vi "MultiOpto_1.1_Host.vi"() -> ()   [LabVIEW 2018]
uses:
  D:/NI LabVIEW/MultiOpto 1.1/AT lib/Spels.AutomationTools.Utility.Wcf.dll
  AT lib/Spels.AutomationTools.Utility.Wcf.dll
  D:/NI LabVIEW/MultiOpto 1.1/AT lib/AmateurStepperMotor.dll
  AT lib/AmateurStepperMotor.dll
  <instrlib>/niDMM/nidmm.llb/niDMM Resolution in Digits.ctl
  <instrlib>/niDMM/nidmm.llb/niDMM Function.ctl
  <instrlib>/niDCPower/nidcpower.llb/niDCPower Measurement Type.ctl
  <instrlib>/niDMM/nidmm.llb/niDMM Configure Measurement Digits.vi
  <instrlib>/niScope/Configure/Trigger/niScope Configure Trigger Window.vi
  <instrlib>/niScope/Acquire/Fetch/niScope Multi Fetch Cluster.vi
  <instrlib>/niScope/Acquire/Fetch/niScope Fetch.vi
panel:
  in  "Table Tab":enum32{"Glass Table", "Var"}(tab)
  in  "Add Log Remark":bool
  in  "Glass Table":string[][](table)=[["", "455 nm", "808 nm", "1550 nm"], ["Glass 1 (H-ZLaF90)", "", "", ""], ["Glass 2 (H-K9L)", "", "", ""], ["Glass 3 (H-ZF7LA)", "", "", ""], ["Glass 4 (H-LaK7A)", "", "", ""]]
  in  "Clear Table":bool
  out "Num of Meas":u32
  in  "Log Remark":string
  out "WL 808":dbl format="%#_4g"
  out "WL 455":dbl format="%#_4g"
  out "WL 1550":dbl format="%#_4g"
  out "WL 1550 Ref":dbl=1.0 format="%#_4g"
  out "WL 455 Ref":dbl=1.0 format="%#_4g"
  out "WL 808 Ref":dbl=1.0 format="%#_4g"
  out "WL 455 Absolute/Reference":string="-" caption="WL 455 Abs/Ref"
  out "WL 808 Absolute/Reference":string="-" caption="WL 808 Abs/Ref"
  out "WL 1550 Absolute/Reference":string="-" caption="WL 1550 Abs/Ref"
  in  "Set Last Meas As Ref":bool
  in  "HMI Stop":bool
  in  "NI Scope":refnum<k15>="PXI1Slot9_2" caption="Scope"
  in  "NI DMM 3":refnum<k15>="PXI1Slot6_3" caption="NI DMM 2"
  in  "Stepper Motor Control":enum32{"Stepper Motor", "System Panel", "Var"}(tab)
  out "Текущая позиция":dbl
  in  "Куда едем?":T1(ring)
  in  "Glass Meas":bool caption="Glass Measurement"
  out "Meas Running":bool
  out "Glass Meas Cycle Running":bool caption="Cycle Running"
  in  "Погнали!":bool
  out "Готово":bool
  in  "Glass Meas Cycle":bool caption="Glass Measament Cycle"
  out "Meas Progress Bar":u8(slide) caption="Measurement Progress Bar" scale=0.0..100.0
  out "Stepper Motor Status":bool=TRUE
  in  "StepDivisor":i32(ring)=8 items=["D1"=1, "D2"=2, "D4"=4, "D8"=8, "D16"=16, "D32"=32]
  in  "Speed":dbl=1000.0
  in  "StepMultiplicationFactor":dbl=1.0
  in  "Стоп_тест":bool
  in  "Тест":bool
  in  "Стоп GoTo":bool
  in  "Meas Wait":u32=500
  out "Av Cur Data String":string="0,000016350563\t"
  out "Glass Num Output File":refnum<file>
  out "Glass 1 Output File":refnum<file>
  out "CH Data String":string="1,200000000000\t0,040047418764\t"
  out "All Cur Data String":string="0,000016366024\t0,000016373619\t0,000016386890\t0,000016310874\t0,000016315407\t"
  out "Meas Time String":string="19:17:01:,978\t"
  out "Glass Meas Path":refnum<file>
  out "Glass 2 Output File":refnum<file>
  out "Glass 3 Output File":refnum<file>
  out "Glass 4 Output File":refnum<file>
  out "Glass Full Log Output File":refnum<file>
  out "Save Glass Log Done":bool=TRUE
  in  "Save Glass Log Data":bool
  out "WL-i":i32
  out "Single Meas Output File":refnum<file>
  in  "NI DMM 3 Tab":enum32{"Amp", "Ohm", "System Panel", "Var"}(tab)
  in  "NI DMM 3 Ampermeter path":path=path "D:/NI LabVIEW/MultiOpto 1.1/Logs/DMM 3" caption="Ampermeter Path"
  out "NI DMM 3 Current Char":dbl(graph)=0.00060711613514286
  in  "NI DMM 3 Current Wait":u32=100 caption="Wait"
  out "NI DMM 3 Current":dbl=0.00060711613514286 caption="Current" format="%_6g"
  in  "NI DMM 3 units":string(combo)="1000000" caption="Units"
  in  "NI DMM 3 Current Range":string(combo)="-1" caption="Range"
  in  "NI DMM 3 Ohmmeter path":path=path "C:/AAB/MultiOpto/NI DMM 2" caption="Ohmmeter Path"
  out "NI DMM 3 Resistance Char":dbl(graph)=6.67426339573744e-05
  in  "NI DMM 3 Resistance Wait":u32=100 caption="Wait"
  out "NI DMM 3 Resistance":dbl caption="Resistance" format="%_6g"
  in  "NI DMM 3 Resistance units":string(combo)="1" caption="Units"
  in  "NI DMM 3 Resistance Range":string(combo)="-1" caption="Range"
  out "NI DMM 3 Current output file":refnum<file>
  out "NI DMM 3 Resistance output file":refnum<file>
  in  "NI DMM 3 error in":errorcluster
  out "NI DMM 3 Status":bool=TRUE
  out "NI DMM 3 Option Return":enum32{"Ampermeter button", "Ohmmeter button"}(ring)
  out "NI DMM 3 error out":errorcluster
  out "DMM 3 Real Current":dbl=6.0711613514286e-10 format="%.5f"
  in  "NI DMM 1":refnum<k15>="PXI1Slot4"
  in  "NI DMM 2":refnum<k15>="PXI1Slot5"
  in  "All Glass Path":path=path "D:/NI LabVIEW/MultiOpto 1.1/Logs/All Glass"
  in  "Ophir 2 Tab":enum32{"Ophir 2", "System Panel"}(tab)
  out "Ophir 2 Initialization":bool caption="Initialization"
  in  "Ophir 2 Clear":bool caption="Clear"
  out "Ophir 2 MAX":dbl caption="MAX" format="%#_5g"
  out "Ophir 2 Optical Power":dbl caption="Power" format="%#_4g"
  in  "Ophir 2 units":string(combo)="1000" caption="Units"
  in  "Ophir 2 Info":u16(ring)=1 caption="Info" items=["Device : JUNO; s/n:903794", "Head : PD300-IRG-v1; s/n:908004"]
  in  "Ophir 2 Wait":u32=100 caption="Wait"
  out "Ophir 2 Char":dbl(graph)=6.67426339573744e-05
  out "Ophir 2 Over Range":bool caption="Over Range"
  out "Ophir 2 dup Visa Session":refnum<visa-resource-name>="USB0::0x0BD3::0x0777::NI-VISA-10003::RAW" caption="dup Visa Session"
  in  "Ophir 2 GPIB Address (10)":string="10" caption="GPIB Address (10)"
  in  "Ophir 2 Select Communication Protocol":u16(ring) caption="Select Communication Protocol" items=["USB", "RS232", "GPIB"]
  in  "Ophir 2 usb channel":i16 caption="usb channel"
  in  "Ophir 2 Baud Rate (3:9600)":i16(ring)=3 caption="Baud Rate (3:9600)" items=["300", "1200", "4800", "9600", "19200", "38400"]
  in  "Ophir 2 Port Number (default 2)":i16=2 caption="Port Number (default 2)" min=0 max=20
  out "Ophir 2 Status":bool caption="Status"
  out "Ophir 2 Real Optical Power":dbl format="%.6e"
  in  "Ophir 1 Tab":enum32{"Ophir 1", "System Panel"}(tab)
  out "Ophir 1 Initialization":bool caption="Initialization"
  in  "Ophir 1 units":string(combo)="1000" caption="Units"
  out "Ophir 1 Optical Power":dbl caption="Power" format="%#_4g"
  out "Ophir 1 MAX":dbl caption="MAX" format="%#_5g"
  in  "Ophir 1 Clear":bool caption="Clear"
  in  "Ophir 1 Info":u16(ring)=1 caption="Info" items=["Device : JUNO; s/n:903795", "Head : PD300R-IR   ; s/n:873888"]
  in  "Ophir 1 Wait":u32=100 caption="Wait"
  out "Ophir 1 Char":dbl(graph)=6.67426339573744e-05
  out "Ophir 1 Over Range":bool caption="Over Range"
  in  "Ophir 1 Select Communication Protocol":u16(ring) caption="Select Communication Protocol" items=["USB", "RS232", "GPIB"]
  in  "Ophir 1 usb channel":i16 caption="usb channel"
  in  "Ophir 1 Port Number (default 2)":i16=1 caption="Port Number (default 2)" min=0 max=20
  in  "Ophir 1 Baud Rate (3:9600)":i16(ring)=3 caption="Baud Rate (3:9600)" items=["300", "1200", "4800", "9600", "19200", "38400"]
  in  "Ophir 1 GPIB Address (10)":string="10" caption="GPIB Address (10)"
  out "Ophir 1 dup Visa Session":refnum<visa-resource-name>="USB0::0x0BD3::0x0777::NI-VISA-10003::RAW" caption="dup Visa Session"
  out "Ophir 1 Status":bool caption="Status"
  out "Ophir 1 Real Optical Power":dbl format="%.6e"
  out "Образец №":string="0"
  in  "NI DMM 2 Tab":enum32{"Amp", "Ohm", "System Panel", "Var"}(tab)
  out "NI DMM 2 Current":dbl=0.7074877999002638 caption="Current" format="%_4g"
  out "NI DMM 2 Current Char":dbl(graph)=0.7074877999002638
  in  "NI DMM 2 Ampermeter path":path=path "D:/NI LabVIEW/MultiOpto 1.1/Logs/DMM 2" caption="Ampermeter Path"
  in  "NI DMM 2 units":string(combo)="1000000" caption="Units"
  in  "NI DMM 2 Current Range":string(combo)="-1" caption="Range"
  in  "NI DMM 2 Current Wait":u32=100 caption="Wait"
  in  "NI DMM 2 Ohmmeter path":path=path "C:/AAB/MultiOpto/NI DMM 2" caption="Ohmmeter Path"
  out "NI DMM 2 Resistance":dbl caption="Resistance" format="%_6g"
  out "NI DMM 2 Resistance Char":dbl(graph)=6.67426339573744e-05
  in  "NI DMM 2 Resistance units":string(combo)="1" caption="Units"
  in  "NI DMM 2 Resistance Range":string(combo)="-1" caption="Range"
  in  "NI DMM 2 Resistance Wait":u32=100 caption="Wait"
  out "NI DMM 2 Status":bool=TRUE
  out "NI DMM 2 Current output file":refnum<file>
  out "NI DMM 2 error out":errorcluster
  in  "NI DMM 2 error in":errorcluster
  out "NI DMM 2 Option Return":enum32{"Ampermeter button", "Ohmmeter button"}(ring)
  out "NI DMM 2 Resistance output file":refnum<file>
  out "DMM 2 Real Current":dbl=7.074877999002638e-07 format="%.5f"
  in  "NI DMM 1 Tab":enum32{"Amp", "Ohm", "System Panel", "Var"}(tab)
  out "NI DMM 1 Current Char":dbl(graph)=0.6705812438667635
  out "NI DMM 1 Current":dbl=0.6705812438667635 caption="Current" format="%_6g"
  in  "NI DMM 1 Ampermeter path":path=path "D:/NI LabVIEW/MultiOpto 1.1/Logs/DMM 1" caption="Ampermeter Path"
  in  "NI DMM 1 units":string(combo)="1000000" caption="Units"
  in  "NI DMM 1 Current Range":string(combo)="-1" caption="Range"
  in  "NI DMM 1 Current Wait":u32=100 caption="Wait"
  in  "NI DMM 1 Ohmmeter path":path=path "C:/AAB/MultiOpto/NI DMM 1" caption="Ohmmeter Path"
  out "NI DMM 1 Resistance":dbl caption="Resistance" format="%_6g"
  out "NI DMM 1 Resistance Char":dbl(graph)=6.67426339573744e-05
  in  "NI DMM 1 Resistance units":string(combo)="1" caption="Units"
  in  "NI DMM 1 Resistance Range":string(combo)="-1" caption="Range"
  in  "NI DMM 1 Resistance Wait":u32=100 caption="Wait"
  out "NI DMM 1 Status":bool=TRUE
  out "NI DMM 1 Current output file":refnum<file>
  out "NI DMM 1 error out":errorcluster
  in  "NI DMM 1 error in":errorcluster
  out "NI DMM 1 Option Return":enum32{"Ampermeter button", "Ohmmeter button"}(ring)
  out "NI DMM 1 Resistance output file":refnum<file>
  out "DMM 1 Real Current":dbl=6.705812438667635e-07 format="%.5f"
  out "SEL":bool
  out "SEU":bool caption="SEL"
  in  "NI Scope Tab":enum32{"NI Scope", "System Panel"}(tab)
  in  "vertical range":dbl=2.0 caption="Vertical Range" format="%.2f"
  out "RealTime Waveform":T2(graph) caption="PC_MON Waveform"
  out "SEU Waveform":T2(graph) caption="SHUTDOWN Waveform"
  in  "Low Level":dbl=0.35 format="%.2f"
  in  "High Level":dbl=0.65 format="%.2f"
  in  "AC/DC/Groun":i32(ring)=1 items=["AC", "DC", "Ground"]
  in  "Trigger Source":string(combo)="0"
  in  "SEU path":path=path "D:/NI LabVIEW/MultiOpto 1.1/Logs/SEU" caption="SEU Path"
  in  "Channel for SEU":T3(radio)
  out "SEU Last Level":dbl
  out "SEU_Counter":u32 caption="SEU counter"
  out "SEU_warning":bool caption="Find SEL"
  out "SEU output file refnum":refnum<file>
  out "NI Scope Status":bool
  out "NI Scope error out":errorcluster
  in  "NI Scope error in":errorcluster
  in  "DC Power Tab":enum32{"DC-Power", "System Panel"}(tab)
  out "P2 CH1_warning":bool caption="VCC_warning"
  out "P2 CH1_counter":u32 caption="VCC_counter"
  in  "P2 CH1_selcur, A":dbl=0.6 caption="current limit" format="%_6p"
  in  "P2 CH1 Used":bool caption="CH1"
  in  "P2 CH1":bool
  out "P2 CH1_char":dbl(graph)=-6.586231837824974e-06
  in  "P2 CH1, V":dbl=20.0 caption="voltage level" min=0.0 max=20.0 format="%_6p"
  out "P2 CH1_cur, A":dbl=-6.586231837824974e-06 caption="measurement" format="%_6g"
  in  "P2 CH1_curlim, A":dbl=0.1 caption="current limit" min=0.01 max=1.0 format="%_6p"
  in  "P1 CH0_selcur, A":dbl=0.2 caption="current limit" format="%_6p"
  in  "P1 CH1_selcur, A":dbl=0.2 caption="current limit" format="%_6p"
  in  "P2 CH0_selcur, A":dbl=0.2 caption="current limit" format="%_6p"
  out "P2 CH0_counter":u32 caption="VCC_counter"
  out "P2 CH0_warning":bool caption="VCC_warning"
  out "P1 CH1_counter":u32 caption="VCC_counter"
  out "P1 CH1_warning":bool caption="VCC_warning"
  out "P1 CH0_counter":u32 caption="VCC_counter"
  out "P1 CH0_warning":bool caption="VCC_warning"
  in  "P2 CH0":bool
  in  "P1 CH1":bool
  in  "P1 CH0":bool
  in  "P2 CH0_curlim, A":dbl=0.04 caption="current limit" min=0.01 max=1.0 format="%_6p"
  out "P2 CH0_cur, A":dbl=0.00011627237241327378 caption="measurement" format="%_6g"
  in  "P2 CH0, V":dbl=1.2000000000000002 caption="voltage level" min=0.0 max=6.0 format="%_6p"
  out "P2 CH0_char":dbl(graph)=0.00011627237241327378
  in  "P1 CH1_curlim, A":dbl=0.1 caption="current limit" min=0.01 max=1.0 format="%_6p"
  out "P1 CH1_cur, A":dbl=9.464711192498274e-07 caption="measurement" format="%_6g"
  in  "P1 CH1, V":dbl=2.0 caption="voltage level" min=0.0 max=20.0 format="%_6p"
  out "P1 CH1_char":dbl(graph)=9.464711192498274e-07
  in  "P1 CH0_curlim, A":dbl=0.08 caption="current limit" min=0.01 max=1.0 format="%_6p"
  out "P1 CH0_cur, A":dbl=8.200132019086688e-05 caption="measurement" format="%_6g"
  in  "P1 CH0, V":dbl=3.3000000000000003 caption="voltage level" min=0.0 max=6.0 format="%_6p"
  out "P1 CH0_char":dbl(graph)=8.200132019086688e-05
  in  "DC POWER 2":refnum<k15>="PXI1Slot3_3" caption="PRBS"
  in  "DC POWER 1":refnum<k15>="PXI1Slot2_2" caption="VСС_+5"
  in  "P1 CH0 Used":bool caption="CH0"
  in  "P2 CH0 Used":bool caption="CH0"
  in  "P1 CH1 Used":bool caption="CH1"
  in  "SIM_SEL":bool
  in  "SEL path":path=path "D:/NI LabVIEW/MultiOpto 1.1/Logs/SEL" caption="SEL Path"
  in  "P1 CH2":bool
  out "P1 CH2_char":dbl(graph)=1.4003158139382402e-06
  in  "P1 CH2, V":dbl=-5.0 caption="voltage level" min=-20.0 max=0.0 format="%_6p"
  out "P1 CH2_cur, A":dbl=1.4003158139382402e-06 caption="measurement" format="%_6g"
  in  "P1 CH2_curlim, A":dbl=0.01 caption="current limit" min=0.01 max=1.0 format="%_6p"
  in  "P2 CH2":bool
  out "P2 CH2_char":dbl(graph)=-2.6497095286784e-07
  in  "P2 CH2, V":dbl caption="voltage level" min=-20.0 max=0.0 format="%_6p"
  out "P2 CH2_cur, A":dbl=-2.6497095286784e-07 caption="measurement" format="%_6g"
  in  "P2 CH2_curlim, A":dbl=0.015 caption="current limit" min=0.01 max=1.0 format="%_6p"
  in  "P1 CH2 Used":bool caption="CH2"
  in  "P2 CH2 Used":bool caption="CH2"
  in  "SEL Time Cycle":u32=100
  in  "P1 CH2_selcur, A":dbl=0.2 caption="current limit" format="%_6p"
  out "P1 CH2_warning":bool caption="VCC_warning"
  out "P1 CH2_counter":u32 caption="VCC_counter"
  out "P2 CH2_counter":u32 caption="VCC_counter"
  out "P2 CH2_warning":bool caption="VCC_warning"
  in  "P2 CH2_selcur, A":dbl=0.2 caption="current limit" format="%_6p"
  out "Power OFF":bool=TRUE
  in  "Считать SIM_SEL":bool
  out "Ready Status":bool=TRUE
  out "DC Power 2 error out":errorcluster
  out "DC Power 1 error out":errorcluster
  out "SEL output file refnum":refnum<file>
  out "Ophir 1 error out":errorcluster caption="error out"
  in  "Ophir 1 error in (no error)":errorcluster caption="error in (no error)"
  in  "Ophir 2 error in (no error)":errorcluster caption="error in (no error)"
  out "Ophir 2 error out":errorcluster caption="error out"
  in  "System Stop":bool=TRUE
  # "Че там?"
  # "P1 CH0, DMM1 = 455 нм"
  # "P1 CH1, DMM2 = 808 нм"
  # "P2 CH0, DMM3 = 1550 нм"
  # "P1 CH2 = Фотодиоды"
  # "P2 CH1 = Шаговик"
  # "Отожми кнопку для\nединичного промера!"
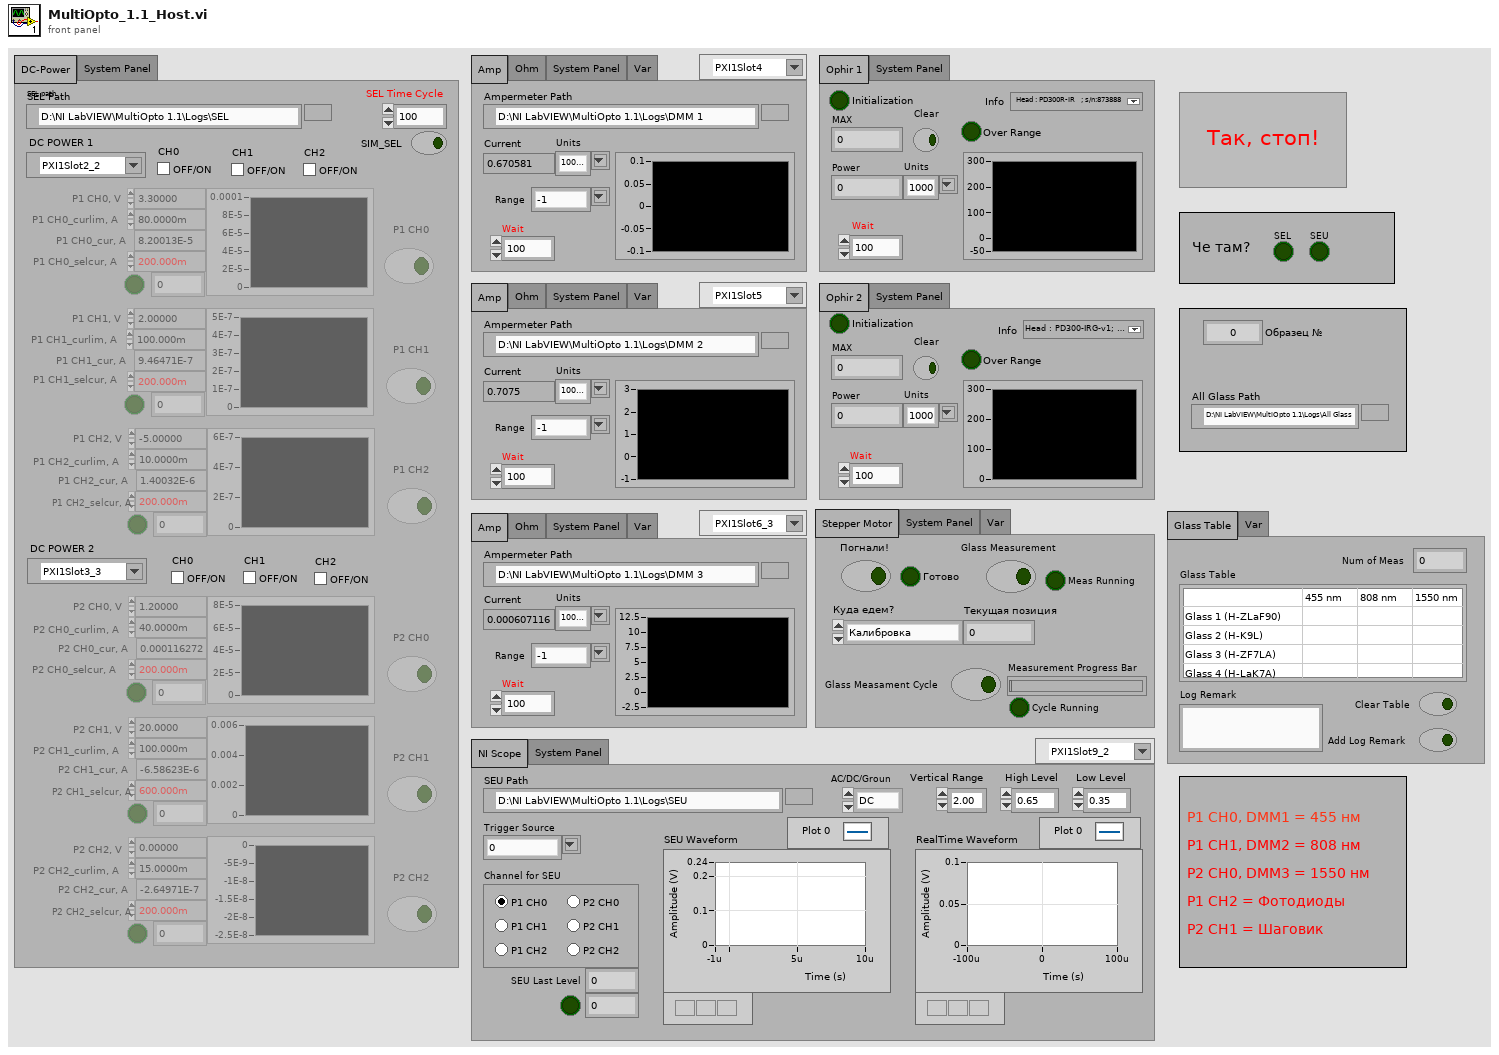
[diagram p1: front panel]
types:
  T1 = enum16{"Калибровка", "Первое стекло", "Второе стекло", "Третье стекло", "Четвертое стекло"}
  T2 = cluster{"relativeInitialX":dbl, "xIncrement":dbl, "wfm":dbl[]}[]
  T3 = enum32{"Radio Selection P1 CH0", "Radio Selection P1 CH1", "Radio Selection P2 CH0", "Radio Selection P2 CH1", "Radio Selection P2 CH2", "Radio Selection P1 CH2"}
  T4 = enum16{"open", "replace", "create", "open or create", "replace or create", "replace or create with confirmation"}
  T5 = enum8{"Enabled", "Disabled", "Disabled and Grayed Out"}
  T6 = typedef "niDMM Function.ctl" = enum16{"DC Volts", "AC Volts", "DC Current", "AC Current", "2-wire Resistance", "4-wire Resistance", "Diode", "Frequency", "Period", "AC Volts DC Coupled", "Capacitance", "Inductance", "Temperature"}
  T7 = typedef "niDMM Resolution in Digits.ctl" = dbl
  T8 = typedef "niDCPower Measurement Type.ctl" = i32
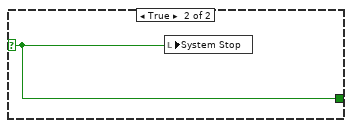
[diagram p3: hidden frame]
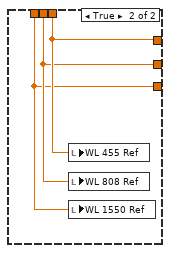
[diagram p7: hidden frame]
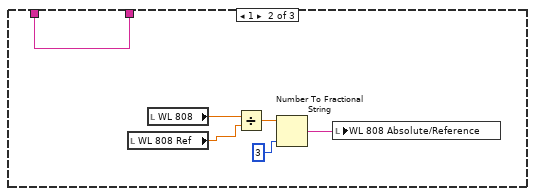
[diagram p8: hidden frame]
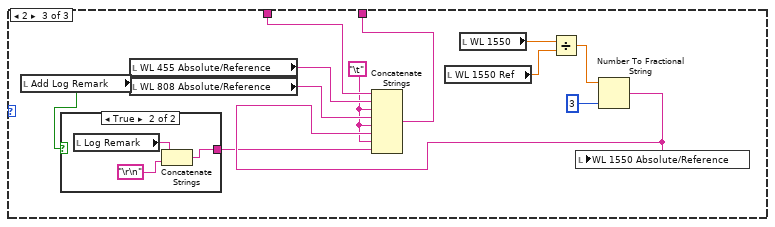
[diagram p9: hidden frame]
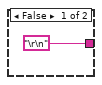
[diagram p10: hidden frame]
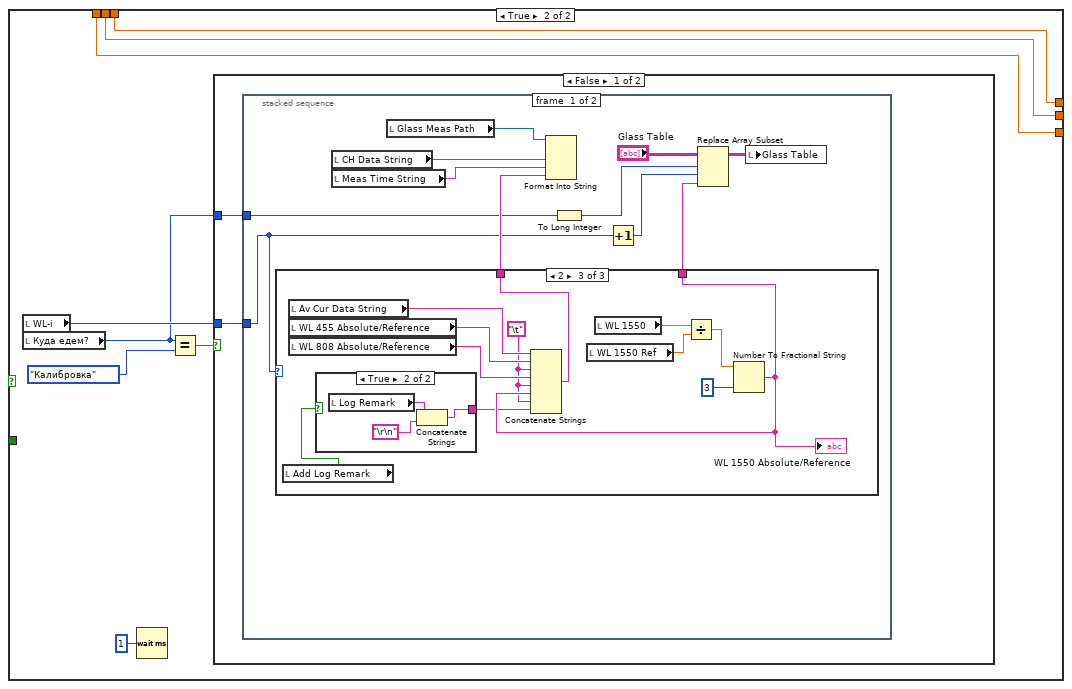
[diagram p11: hidden frame]
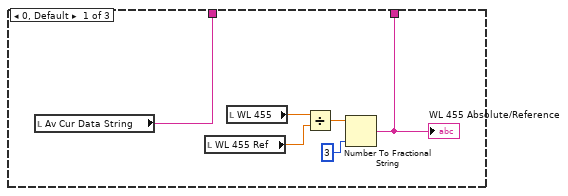
[diagram p12: hidden frame]
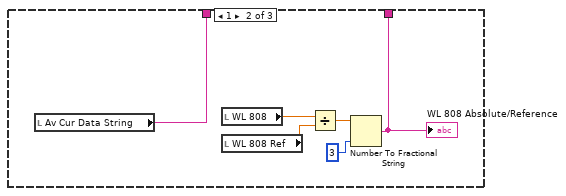
[diagram p13: hidden frame]
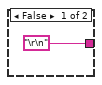
[diagram p14: hidden frame]
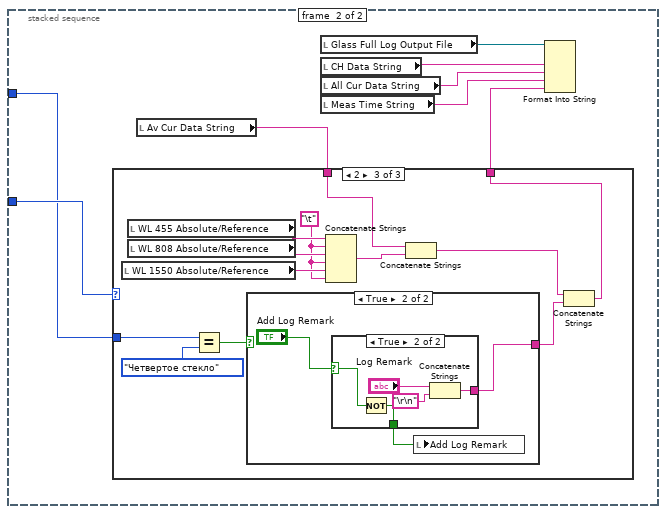
[diagram p15: hidden frame]
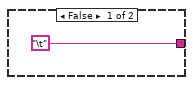
[diagram p18: hidden frame]
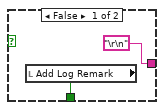
[diagram p19: hidden frame]
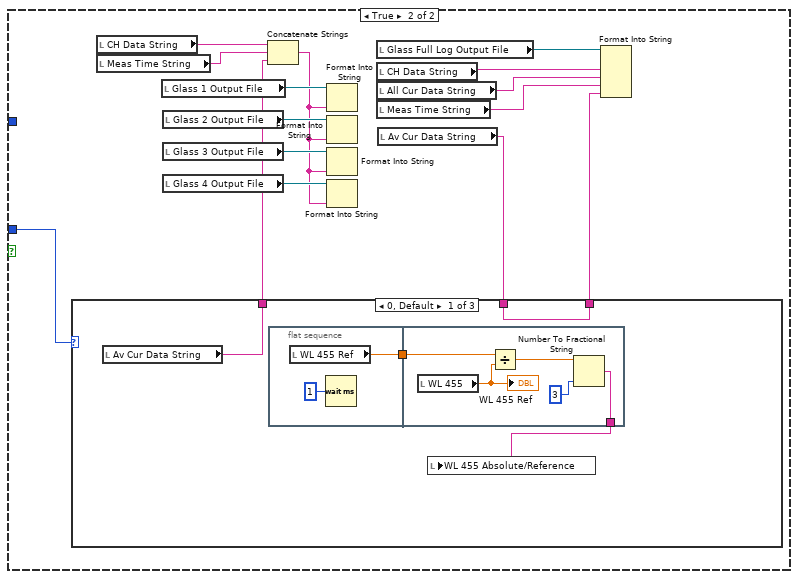
[diagram p20: hidden frame]
diagram:
  # "DMM 3"
  # "DMM 2"
  # "DMM 1"
  n1 = stacked-sequence {
    tunnel: [_ _ _ _ _ w322 _ _ _ _ _ _] -> w33
    tunnel: [_ _ _ _ _ w321 _ _ _ _ _ _] -> w32
    tunnel: [_ _ _ _ _ w320 _ _ _ _ _ _] -> w28
    tunnel: [_ _ _ _ _ w319 _ _ _ _ _ _] -> w27
    tunnel: [_ _ _ _ _ _ _ _ _ _ _ w661] -> w1
    tunnel: [_ _ _ _ _ _ _ _ _ _ _ w661] -> w3
    tunnel: [_ _ _ _ _ _ w335 _ _ _ _ _] -> w26
    tunnel: [_ _ _ _ _ _ _ w394 _ _ _ _] -> w25
    tunnel: [_ _ _ _ _ _ _ w397 _ _ _ _] -> w24
    tunnel: [_ _ _ _ _ _ w334 _ _ _ _ _] -> w23
    tunnel: [_ _ _ _ _ _ _ w393 _ _ _ _] -> w22
    tunnel: [_ _ _ _ _ _ _ w392 _ _ _ _] -> w21
    tunnel: [_ _ _ _ _ _ w333 _ _ _ _ _] -> w20
    tunnel: [_ _ _ _ _ _ _ w396 _ _ _ _] -> w19
    tunnel: [_ _ _ _ _ _ _ w395 _ _ _ _] -> w18
    tunnel: [_ _ _ _ _ _ _ _ w590 _ _ _] -> w17
    tunnel: [_ _ _ _ _ _ _ _ _ w613 _ _] -> w16
    tunnel: [_ _ _ _ _ _ _ w391 _ _ _ _] -> w2
    tunnel: [_ _ _ _ _ _ _ w390 _ _ _ _] -> w15
    tunnel: [_ _ _ _ _ _ _ w389 _ _ _ _] -> w14
    tunnel: [_ _ _ _ _ _ _ _ _ _ w639 _] -> w13
    tunnel: [_ _ _ _ _ _ _ _ _ _ w638 _] -> w12
    tunnel: [_ _ _ _ _ _ _ _ _ _ w637 _] -> w11
    tunnel: [_ _ _ _ _ _ _ _ _ _ w636 _] -> w10
    frame #0 {
      w49 = FALSE ("Clear Table")
      w52 = "-" ("WL 455 Absolute/Reference")
      w53 = 0.0 ("WL 455 Ref")
      w54 = 1.0 ("WL 455")
      w56 = "\t" ("Meas Time String")
      w58 = FALSE ("Save Glass Log Done")
      w60 = FALSE ("Погнали!")
      w64 = FALSE
      w63 = FALSE ("NI Scope Status")
      w67 = u32 0 ("SEU_Counter")
      w57 = FALSE ("STOP")
      # "Начальная конфигурация переменных"
      n2 = local write "Текущая позиция"(0.0 ("Текущая позиция")) -> ()
      n3 = local write "Куда едем?"(T1."Калибровка" ("Куда едем?")) -> ()
      n4 = local write "Погнали!"(w60) -> ()
      n5 = local write "Тест"(w60) -> ()
      n6 = local write "Стоп GoTo"(w60) -> ()
      n7 = local write "Стоп_тест"(w60) -> ()
      n8 = local write "Готово"(w60) -> ()
      n9 = local write "Num of Meas"(u32 0 ("Num of Meas")) -> ()
      n10 = local write "WL 455"(w54) -> ()
      n11 = local write "WL 808"(w54) -> ()
      n12 = local write "WL 1550"(w54) -> ()
      n13 = local write "WL 455 Ref"(w53) -> ()
      n14 = local write "WL 808 Ref"(w53) -> ()
      n15 = local write "WL 1550 Ref"(w53) -> ()
      n16 = local write "WL 455 Absolute/Reference"(w52) -> ()
      n17 = local write "WL 808 Absolute/Reference"(w52) -> ()
      n18 = local write "WL 1550 Absolute/Reference"(w52) -> ()
      n19 = local write "Ophir 2 Over Range"(w64) -> ()
      n20 = local write "Ophir 1 Over Range"(w64) -> ()
      n21 = local write "Ophir 1 Initialization"(w64) -> ()
      n22 = local write "Ophir 2 Initialization"(w64) -> ()
      n23 = local write "Ophir 1 Clear"(w64) -> ()
      n24 = local write "Ophir 2 Clear"(w64) -> ()
      n25 = local write "Meas Time String"(w56) -> ()
      n26 = local write "All Cur Data String"(w56) -> ()
      n27 = local write "Av Cur Data String"(w56) -> ()
      n28 = local write "CH Data String"(w56) -> ()
      n29 = local write "WL-i"(0 ("i-WL")) -> ()
      n30 = local write "Save Glass Log Data"(w58) -> ()
      n31 = local write "Save Glass Log Done"(w58) -> ()
      n32 = local write "Glass Meas Cycle"(w58) -> ()
      n33 = local write "Glass Meas"(w58) -> ()
      n34 = local write "Meas Running"(w58) -> ()
      n35 = local write "Glass Meas Cycle Running"(w58) -> ()
      n36 = local write "HMI Stop"(w57) -> ()
      n37 = local write "System Stop"(w57) -> ()
      n38 = local write "P1 CH0"(w57) -> ()
      n39 = local write "P1 CH1"(w57) -> ()
      n40 = local write "P2 CH0"(w57) -> ()
      n41 = local write "P2 CH1"(w57) -> ()
      n42 = local write "Power OFF"(w57) -> ()
      n43 = local write "P1 CH0 Used"(w57) -> ()
      n44 = local write "P1 CH1 Used"(w57) -> ()
      n45 = local write "P1 CH2 Used"(w57) -> ()
      n46 = local write "P2 CH0 Used"(w57) -> ()
      n47 = local write "P2 CH1 Used"(w57) -> ()
      n48 = local write "P2 CH2 Used"(w57) -> ()
      n49 = local write "Считать SIM_SEL"(w57) -> ()
      n50 = local write "SEL"(w57) -> ()
      n51 = local write "SEU"(w57) -> ()
      n52 = local write "SEU_warning"(w57) -> ()
      n53 = local write "P1 CH0_warning"(w57) -> ()
      n54 = local write "P1 CH1_warning"(w57) -> ()
      n55 = local write "P2 CH0_warning"(w57) -> ()
      n56 = local write "P2 CH1_warning"(w57) -> ()
      n57 = local write "SEU_warning"(w57) -> ()
      n58 = local write "Log Remark"("" ("Log Remark")) -> ()
      n59 = local write "Set Last Meas As Ref"(w49) -> ()
      n60 = local write "Clear Table"(w49) -> ()
      n61 = local write "Add Log Remark"(w49) -> ()
      n62 = local write "SEU Last Level"(0.0 ("SEU Level")) -> ()
      n63 = local write "SEU_Counter"(w67) -> ()
      n64 = local write "P1 CH0_counter"(w67) -> ()
      n65 = local write "P1 CH1_counter"(w67) -> ()
      n66 = local write "P2 CH0_counter"(w67) -> ()
      n67 = local write "P2 CH1_counter"(w67) -> ()
      n68 = local write "Образец №"("" ("Образец №")) -> ()
      n69 = local write "Ready Status"(FALSE ("Ready Status")) -> ()
      n70 = local write "NI Scope Status"(w63) -> ()
      n71 = local write "NI DMM 2 Status"(w63) -> ()
      n72 = local write "NI DMM 1 Status"(w63) -> ()
      n73 = local write "NI DMM 3 Status"(w63) -> ()
      n74 = local write "Ophir 1 Status"(w63) -> ()
      n75 = local write "Ophir 2 Status"(w63) -> ()
      n76 = local write "Stepper Motor Status"(w63) -> ()
      "Meas Progress Bar" <- u8 0 ("Measuering Progress Bar")
    }
    frame #1 {
      n77 = stacked-sequence {
        frame #0 {
          w69 = T5."Disabled and Grayed Out" ("Disabled")
          n78 = property on="P1 CH0" class="Bool (strict)"("DisabledEnum"=w69) -> ()  [unwired: 2 in, 2 out]
          n79 = property on="P1 CH0_char" class="WFChart (strict)"("DisabledEnum"=w69) -> ()  [unwired: 2 in, 2 out]
          n80 = property on="P1 CH0, V" class="DigNum (strict)"("DisabledEnum"=w69) -> ()  [unwired: 2 in, 2 out]
          n81 = property on="P1 CH0_curlim, A" class="DigNum (strict)"("DisabledEnum"=w69) -> ()  [unwired: 2 in, 2 out]
          n82 = property on="P1 CH0_cur, A" class="DigNum (strict)"("DisabledEnum"=w69) -> ()  [unwired: 2 in, 2 out]
          n83 = property on="P1 CH0_selcur, A" class="DigNum (strict)"("DisabledEnum"=w69) -> ()  [unwired: 2 in, 2 out]
          n84 = property on="P1 CH0_counter" class="DigNum (strict)"("DisabledEnum"=w69) -> ()  [unwired: 2 in, 2 out]
          n85 = property on="P1 CH0_warning" class="Bool (strict)"("DisabledEnum"=w69) -> ()  [unwired: 2 in, 2 out]
        }
        frame #1 {
          w70 = T5."Disabled and Grayed Out" ("Disabled")
          n86 = property on="P1 CH1" class="Bool (strict)"("DisabledEnum"=w70) -> ()  [unwired: 2 in, 2 out]
          n87 = property on="P1 CH1_char" class="WFChart (strict)"("DisabledEnum"=w70) -> ()  [unwired: 2 in, 2 out]
          n88 = property on="P1 CH1, V" class="DigNum (strict)"("DisabledEnum"=w70) -> ()  [unwired: 2 in, 2 out]
          n89 = property on="P1 CH1_curlim, A" class="DigNum (strict)"("DisabledEnum"=w70) -> ()  [unwired: 2 in, 2 out]
          n90 = property on="P1 CH1_cur, A" class="DigNum (strict)"("DisabledEnum"=w70) -> ()  [unwired: 2 in, 2 out]
          n91 = property on="P1 CH1_selcur, A" class="DigNum (strict)"("DisabledEnum"=w70) -> ()  [unwired: 2 in, 2 out]
          n92 = property on="P1 CH1_counter" class="DigNum (strict)"("DisabledEnum"=w70) -> ()  [unwired: 2 in, 2 out]
          n93 = property on="P1 CH1_warning" class="Bool (strict)"("DisabledEnum"=w70) -> ()  [unwired: 2 in, 2 out]
        }
        frame #2 {
          w71 = T5."Disabled and Grayed Out" ("Disabled")
          n94 = property on="P1 CH2" class="Bool (strict)"("DisabledEnum"=w71) -> ()  [unwired: 2 in, 2 out]
          n95 = property on="P1 CH2_char" class="WFChart (strict)"("DisabledEnum"=w71) -> ()  [unwired: 2 in, 2 out]
          n96 = property on="P1 CH2, V" class="DigNum (strict)"("DisabledEnum"=w71) -> ()  [unwired: 2 in, 2 out]
          n97 = property on="P1 CH2_curlim, A" class="DigNum (strict)"("DisabledEnum"=w71) -> ()  [unwired: 2 in, 2 out]
          n98 = property on="P1 CH2_cur, A" class="DigNum (strict)"("DisabledEnum"=w71) -> ()  [unwired: 2 in, 2 out]
          n99 = property on="P1 CH2_selcur, A" class="DigNum (strict)"("DisabledEnum"=w71) -> ()  [unwired: 2 in, 2 out]
          n100 = property on="P1 CH2_counter" class="DigNum (strict)"("DisabledEnum"=w71) -> ()  [unwired: 2 in, 2 out]
          n101 = property on="P1 CH2_warning" class="Bool (strict)"("DisabledEnum"=w71) -> ()  [unwired: 2 in, 2 out]
        }
        frame #3 {
          w72 = T5."Disabled and Grayed Out" ("Disabled")
          n102 = property on="P2 CH0" class="Bool (strict)"("DisabledEnum"=w72) -> ()  [unwired: 2 in, 2 out]
          n103 = property on="P2 CH0_char" class="WFChart (strict)"("DisabledEnum"=w72) -> ()  [unwired: 2 in, 2 out]
          n104 = property on="P2 CH0, V" class="DigNum (strict)"("DisabledEnum"=w72) -> ()  [unwired: 2 in, 2 out]
          n105 = property on="P2 CH0_curlim, A" class="DigNum (strict)"("DisabledEnum"=w72) -> ()  [unwired: 2 in, 2 out]
          n106 = property on="P2 CH0_cur, A" class="DigNum (strict)"("DisabledEnum"=w72) -> ()  [unwired: 2 in, 2 out]
          n107 = property on="P2 CH0_selcur, A" class="DigNum (strict)"("DisabledEnum"=w72) -> ()  [unwired: 2 in, 2 out]
          n108 = property on="P2 CH0_counter" class="DigNum (strict)"("DisabledEnum"=w72) -> ()  [unwired: 2 in, 2 out]
          n109 = property on="P2 CH0_warning" class="Bool (strict)"("DisabledEnum"=w72) -> ()  [unwired: 2 in, 2 out]
        }
        frame #4 {
          w73 = T5."Disabled and Grayed Out" ("Disabled")
          n110 = property on="P2 CH1" class="Bool (strict)"("DisabledEnum"=w73) -> ()  [unwired: 2 in, 2 out]
          n111 = property on="P2 CH1_char" class="WFChart (strict)"("DisabledEnum"=w73) -> ()  [unwired: 2 in, 2 out]
          n112 = property on="P2 CH1, V" class="DigNum (strict)"("DisabledEnum"=w73) -> ()  [unwired: 2 in, 2 out]
          n113 = property on="P2 CH1_curlim, A" class="DigNum (strict)"("DisabledEnum"=w73) -> ()  [unwired: 2 in, 2 out]
          n114 = property on="P2 CH1_cur, A" class="DigNum (strict)"("DisabledEnum"=w73) -> ()  [unwired: 2 in, 2 out]
          n115 = property on="P2 CH1_selcur, A" class="DigNum (strict)"("DisabledEnum"=w73) -> ()  [unwired: 2 in, 2 out]
          n116 = property on="P2 CH1_counter" class="DigNum (strict)"("DisabledEnum"=w73) -> ()  [unwired: 2 in, 2 out]
          n117 = property on="P2 CH1_warning" class="Bool (strict)"("DisabledEnum"=w73) -> ()  [unwired: 2 in, 2 out]
        }
        frame #5 {
          w74 = T5."Disabled and Grayed Out" ("Disabled")
          n118 = property on="P2 CH2" class="Bool (strict)"("DisabledEnum"=w74) -> ()  [unwired: 2 in, 2 out]
          n119 = property on="P2 CH2_char" class="WFChart (strict)"("DisabledEnum"=w74) -> ()  [unwired: 2 in, 2 out]
          n120 = property on="P2 CH2, V" class="DigNum (strict)"("DisabledEnum"=w74) -> ()  [unwired: 2 in, 2 out]
          n121 = property on="P2 CH2_curlim, A" class="DigNum (strict)"("DisabledEnum"=w74) -> ()  [unwired: 2 in, 2 out]
          n122 = property on="P2 CH2_cur, A" class="DigNum (strict)"("DisabledEnum"=w74) -> ()  [unwired: 2 in, 2 out]
          n123 = property on="P2 CH2_selcur, A" class="DigNum (strict)"("DisabledEnum"=w74) -> ()  [unwired: 2 in, 2 out]
          n124 = property on="P2 CH2_counter" class="DigNum (strict)"("DisabledEnum"=w74) -> ()  [unwired: 2 in, 2 out]
          n125 = property on="P2 CH2_warning" class="Bool (strict)"("DisabledEnum"=w74) -> ()  [unwired: 2 in, 2 out]
        }
        frame #6 {
          w75 = T5."Enabled" ("Disabled")
          n126 = property on="P1 CH0 Used" class="Bool (strict)"("DisabledEnum"=w75) -> ()  [unwired: 2 in, 2 out]
          n127 = property on="P1 CH1 Used" class="Bool (strict)"("DisabledEnum"=w75) -> ()  [unwired: 2 in, 2 out]
          n128 = property on="P1 CH2 Used" class="Bool (strict)"("DisabledEnum"=w75) -> ()  [unwired: 2 in, 2 out]
          n129 = property on="P2 CH0 Used" class="Bool (strict)"("DisabledEnum"=w75) -> ()  [unwired: 2 in, 2 out]
          n130 = property on="P2 CH1 Used" class="Bool (strict)"("DisabledEnum"=w75) -> ()  [unwired: 2 in, 2 out]
          n131 = property on="P2 CH2 Used" class="Bool (strict)"("DisabledEnum"=w75) -> ()  [unwired: 2 in, 2 out]
          n132 = property on="Glass Meas" class="Bool (strict)"("DisabledEnum"=w75) -> ()  [unwired: 2 in, 2 out]
        }
      }
    }
    frame #2 {
      n133 = call "MultiOpto_1.1_Begin.vi"() -> ("NI Scope Status"=→"NI Scope Status":bool, "Stepper Motor Status"=→"Stepper Motor Status":bool, "Ophir 2 Status"=→"Ophir 2 Status":bool, "Ophir 1 Status"=→"Ophir 1 Status":bool, "Текущий Образец №"=→"Образец №":string, "NI DMM 2 option return"=→"NI DMM 2 Option Return":enum32{"Ampermeter button", "Ohmmeter button"}, "NI DMM 3 option return"=→"NI DMM 3 Option Return":enum32{"Ampermeter button", "Ohmmeter button"}, "NI DMM 1 option return"=→"NI DMM 1 Option Return":enum32{"Ampermeter button", "Ohmmeter button"}, "NI DMM 3 Status"=→"NI DMM 3 Status":bool, "NI DMM 2 Status"=→"NI DMM 2 Status":bool, "NI DMM 1 Status"=→"NI DMM 1 Status":bool)  [unwired: 1 in]
    }
    frame #3 {
      n134 = local read "Образец №"() -> (w92:string)
      n135 = Build Path(base path="All Glass Path", name or relative path=w92) -> (appended path=w89:path)
      n136 = call <vilib>:"Check if File or Folder Exists.vi"("path"=w89) -> ("file or folder exists?"=w90:bool, "dup path"=w91:path)  [unwired: 8 in, 1 out]
      n137 = case shown="False" w90 {
        tunnel: w91 -> [w94 w95]
        tunnel: [w93 w95] -> w88
        frame False {
          n138 = Create Folder(path (use dialog)=w94) -> (created path=w93:path)  [unwired: 2 in, 2 out]
        }
        frame True {
        }
      }
      n139 = stacked-sequence {
        tunnel: w88 -> [w148 w178 w225]
        frame #0 {
          w146 = "\t"
          w98 = "\t"
          n140 = local read "Glass Table"() -> (w104:string[][])
          n141 = Index Array(array=w104, index (row)=4 ("disabled index (row)"), index (col)=0 ("disabled index (col)")) -> (element=w102:string)
          n142 = local read "Glass Table"() -> (w109:string[][])
          n143 = Index Array(array=w109, index (row)=3 ("disabled index (row)"), index (col)=0 ("disabled index (col)")) -> (element=w103:string)
          n144 = local read "Glass Table"() -> (w115:string[][])
          n145 = Index Array(array=w115, index (row)=2 ("disabled index (row)"), index (col)=0 ("disabled index (col)")) -> (element=w114:string)
          n146 = Build Path(base path=w148, name or relative path="Full Log") -> (appended path=w165:path)
          n147 = Get Date/Time In Seconds() -> (seconds since 1Jan1904=w161:timestamp)
          n148 = local read "Glass Table"() -> (w113:string[][])
          n149 = call <vilib>:"Check if File or Folder Exists.vi"("path"=w165) -> ("file or folder exists?"=w164:bool, "dup path"=w163:path)  [unwired: 8 in, 1 out]
          n150 = Index Array(array=w113, index (row)=1 ("disabled index (row)"), index (col)=0 ("disabled index (col)")) -> (element=w110:string)
          n151 = Format Date/Time String(time format string (%c)="Full Log %d %m %y %H.%M.%S", seconds (now)=w161) -> (date/time string=w160:string)  [unwired: 1 in]
          n152 = case shown="False" w164 {
            tunnel: w163 -> [w167 w168]
            tunnel: [w166 w168] -> w162
            frame False {
              n153 = Create Folder(path (use dialog)=w167) -> (created path=w166:path)  [unwired: 2 in, 2 out]
            }
            frame True {
            }
          }
          n154 = Concatenate Strings(w160, ".xls" ("string")) -> (w159:string)
          n155 = Build Path(base path=w162, name or relative path=w159) -> (appended path=w158:path)
          n156 = Concatenate Strings("P1 CH0, V" ("string"), w98, "P1 CH0 Current, A" ("string"), w98, "DMM1_1" ("string"), w98, "DMM1_2" ("string"), w98, "DMM1_3" ("string"), w98, "DMM1_4" ("string"), w98, "DMM1_5" ("string"), w98, "Time" ("string"), w98, "455 nm Current Averaged, A" ("string"), w98, "P2 CH0, V" ("string"), w98, "P2 CH0 Current, A" ("string"), w98, "DMM2_1" ("string"), w98, "DMM2_2" ("string"), w98, "DMM2_3" ("string"), w98, "DMM2_4" ("string"), w98, "DMM2_5" ("string"), w98, "Time" ("string"), w98, "808 nm Current Averaged, A" ("string"), w98, "P2 CH1, V" ("string"), w98, "P2 CH2 Current, A" ("string"), w98, "DMM3_1" ("string"), w98, "DMM3_2" ("string"), w98, "DMM3_3" ("string"), w98, "DMM3_4" ("string"), w98, "DMM3_5" ("string"), w98, "Time" ("string"), w98, "1550 nm Current Averaged, A" ("string"), w98, "455 nm Absolute/Reference" ("string"), w98, "808 nm Absolute/Reference" ("string"), w98, "1550 nm Absolute/Reference" ("string"), w98) -> (w145:string)
          n157 = Open/Create/Replace File(file path (use dialog)=w158, operation (0:open)=T4."open or create", access (0:read/write)=enum16{"read/write", "read-only", "write-only"}."read/write") -> (refnum out=w157:refnum<file>)  [unwired: 3 in, 2 out]
          n158 = Set File Position(refnum=w157, from (0:start)=enum16{"start", "end", "current"}."end") -> (refnum out=w155:refnum<file>)  [unwired: 2 in, 1 out]
          n159 = Concatenate Strings(w145, w110, w146, w145, w114, w146, w145, w103, w146, w145, w102, w146, w145, "Log Remarks" ("string"), "\r\n") -> (w154:string)
          n160 = Format Into String(initial string=w155, w154) -> (resulting string=→"Glass Full Log Output File":refnum<file>)  [unwired: 2 in, 1 out]
        }
        frame #1 {
          w171 = "\t"
          n161 = Build Path(base path=w178, name or relative path="Single Measurements") -> (appended path=w220:path)
          n162 = Get Date/Time In Seconds() -> (seconds since 1Jan1904=w216:timestamp)
          n163 = call <vilib>:"Check if File or Folder Exists.vi"("path"=w220) -> ("file or folder exists?"=w219:bool, "dup path"=w218:path)  [unwired: 8 in, 1 out]
          n164 = Format Date/Time String(time format string (%c)="Single Measurements %d %m %y %H.%M.%S", seconds (now)=w216) -> (date/time string=w215:string)  [unwired: 1 in]
          n165 = case shown="False" w219 {
            tunnel: w218 -> [w222 w223]
            tunnel: [w221 w223] -> w217
            frame False {
              n166 = Create Folder(path (use dialog)=w222) -> (created path=w221:path)  [unwired: 2 in, 2 out]
            }
            frame True {
            }
          }
          n167 = Concatenate Strings(w215, ".xls" ("string")) -> (w214:string)
          n168 = Build Path(base path=w217, name or relative path=w214) -> (appended path=w213:path)
          n169 = Concatenate Strings("P1 CH0, V" ("string"), w171, "P1 CH0 Current, A" ("string"), w171, "DMM1_1" ("string"), w171, "DMM1_2" ("string"), w171, "DMM1_3" ("string"), w171, "DMM1_4" ("string"), w171, "DMM1_5" ("string"), w171, "Time" ("string"), w171, "455 nm Current Averaged, A" ("string"), w171, "P1 CH1, V" ("string"), w171, "P1 CH1 Current, A" ("string"), w171, "DMM2_1" ("string"), w171, "DMM2_2" ("string"), w171, "DMM2_3" ("string"), w171, "DMM2_4" ("string"), w171, "DMM2_5" ("string"), w171, "Time" ("string"), w171, "808 nm Current Averaged, A" ("string"), w171, "P2 CH0, V" ("string"), w171, "P2 CH0 Current, A" ("string"), w171, "DMM3_1" ("string"), w171, "DMM3_2" ("string"), w171, "DMM3_3" ("string"), w171, "DMM3_4" ("string"), w171, "DMM3_5" ("string"), w171, "Time" ("string"), w171, "1550 nm Current Averaged, A" ("string"), w171, "455 nm Absolute/Reference" ("string"), w171, "808 nm Absolute/Reference" ("string"), w171, "1550 nm Absolute/Reference" ("string"), w171, "Log Remarks" ("string"), "\r\n") -> (w176:string)
          n170 = Open/Create/Replace File(file path (use dialog)=w213, operation (0:open)=T4."open or create", access (0:read/write)=enum16{"read/write", "read-only", "write-only"}."read/write") -> (refnum out=w212:refnum<file>)  [unwired: 3 in, 2 out]
          n171 = Set File Position(refnum=w212, from (0:start)=enum16{"start", "end", "current"}."end") -> (refnum out=w211:refnum<file>)  [unwired: 2 in, 1 out]
          n172 = Format Into String(initial string=w211, w176) -> (resulting string=→"Single Meas Output File":refnum<file>)  [unwired: 2 in, 1 out]
        }
        frame #2 {
          n173 = for {
            N: 4 -> [_]
            tunnel: w225 -> [w244]
            i -> [w236]
            w228 = "\t"
            w233 = "\t"
            n174 = local read "Glass Table"() -> (w239:string[][])
            n175 = Increment(x=w236) -> (x+1=w235:i32)
            n176 = Index Array(array=w239, index (row)=w235, index (col)=0 ("disabled index (col)")) -> (element=w238:string)
            n177 = Concatenate Strings(w238, " %d %m %y %H.%M.%S" ("time format string (%c)")) -> (w240:string)
            n178 = Build Path(base path=w244, name or relative path=w238) -> (appended path=w271:path)
            n179 = Get Date/Time In Seconds() -> (seconds since 1Jan1904=w267:timestamp)
            n180 = call <vilib>:"Check if File or Folder Exists.vi"("path"=w271) -> ("file or folder exists?"=w270:bool, "dup path"=w269:path)  [unwired: 8 in, 1 out]
            n181 = Format Date/Time String(time format string (%c)=w240, seconds (now)=w267) -> (date/time string=w266:string)  [unwired: 1 in]
            n182 = case shown="False" w270 {
              tunnel: w269 -> [w277 w278]
              tunnel: [w276 w278] -> w268
              frame False {
                n183 = Create Folder(path (use dialog)=w277) -> (created path=w276:path)  [unwired: 2 in, 2 out]
              }
              frame True {
              }
            }
            n184 = Concatenate Strings("P1 CH0, V" ("string"), w233, "P1 CH0 Current, A" ("string"), w233, "Time" ("string"), w233, "455 nm Current Averaged, A" ("string"), w233, "P1 CH1, V" ("string"), w233, "P1 CH1 Current, A" ("string"), w233, "Time" ("string"), w233, "808 nm Current Averaged, A" ("string"), w233, "P2 CH0, V" ("string"), w233, "P2 CH0 Current, A" ("string"), w233, "Time" ("string"), w233, "1550 nm Current Averaged, A" ("string"), w233) -> (w234:string)
            n185 = Concatenate Strings(w266, ".xls" ("string")) -> (w265:string)
            n186 = Build Path(base path=w268, name or relative path=w265) -> (appended path=w264:path)
            n187 = Open/Create/Replace File(file path (use dialog)=w264, operation (0:open)=T4."open or create", access (0:read/write)=enum16{"read/write", "read-only", "write-only"}."read/write") -> (refnum out=w263:refnum<file>)  [unwired: 3 in, 2 out]
            n188 = Concatenate Strings(w234, "455 nm Absolute/Reference" ("string"), w228, "808 nm Absolute/Reference" ("string"), w228, "1550 nm Absolute/Reference" ("string"), w228) -> (w229:string)
            n189 = Set File Position(refnum=w263, from (0:start)=enum16{"start", "end", "current"}."end") -> (refnum out=w258:refnum<file>)  [unwired: 2 in, 1 out]
            n190 = Concatenate Strings(w229, w238, "\t", w229, "Log Remarks" ("string"), "\r\n") -> (w245:string)
            n191 = Format Into String(initial string=w258, w245) -> (resulting string=w243:refnum<file>)  [unwired: 2 in, 1 out]
            n192 = case shown="3" w236 {
              tunnel: w243 -> [w272 w273 w274 w275]
              frame 0, Default {
                "Glass 1 Output File" <- w272
              }
              frame 1 {
                "Glass 2 Output File" <- w273
              }
              frame 2 {
                "Glass 3 Output File" <- w274
              }
              frame 3 {
                "Glass 4 Output File" <- w275
              }
            }
          }
        }
      }
    }
    frame #4 {
      w281 = "\t"
      # "Инициализация файла SEL"
      n193 = local read "Образец №"() -> (w300:string)
      n194 = Build Path(base path="SEL path", name or relative path=w300) -> (appended path=w315:path)
      n195 = Get Date/Time In Seconds() -> (seconds since 1Jan1904=w311:timestamp)
      n196 = call <vilib>:"Check if File or Folder Exists.vi"("path"=w315) -> ("file or folder exists?"=w314:bool, "dup path"=w313:path)  [unwired: 8 in, 1 out]
      n197 = Format Date/Time String(time format string (%c)="SEL %d %m %y %H.%M.%S", seconds (now)=w311) -> (date/time string=w310:string)  [unwired: 1 in]
      n198 = case shown="False" w314 {
        tunnel: w313 -> [w317 w318]
        tunnel: [w316 w318] -> w312
        frame False {
          n199 = Create Folder(path (use dialog)=w317) -> (created path=w316:path)  [unwired: 2 in, 2 out]
        }
        frame True {
        }
      }
      n200 = Concatenate Strings(w310, ".xls" ("string")) -> (w307:string)
      n201 = Build Path(base path=w312, name or relative path=w307) -> (appended path=w304:path)
      n202 = Open/Create/Replace File(file path (use dialog)=w304, operation (0:open)=T4."open or create", access (0:read/write)=enum16{"read/write", "read-only", "write-only"}."read/write") -> (refnum out=w303:refnum<file>)  [unwired: 3 in, 2 out]
      n203 = Set File Position(refnum=w303, from (0:start)=enum16{"start", "end", "current"}."end") -> (refnum out=w282:refnum<file>)  [unwired: 2 in, 1 out]
      n204 = Format Into String(initial string=w282, "Time" ("string"), w281, "P1 CH0, V" ("string"), w281, "P1 CH0_cur, A" ("string"), w281, "P1 CH0_counter" ("string"), w281, "!!!0" ("input 7"), w281, "P1 CH1, V" ("string"), w281, "P1 CH1_cur, A" ("string"), w281, "P1 CH1_counter" ("string"), w281, "!!!1" ("input 7"), w281, "P2 CH0, V" ("string"), w281, "P2 CH0_cur, A" ("string"), w281, "P2 CH0_counter" ("string"), w281, "!!!2" ("input 7"), w281, "P2 CH1, V" ("string"), w281, "P2 CH1_cur, A" ("string"), w281, "P2 CH1_counter" ("string"), "!!!3" ("input 7"), "\r\n") -> (resulting string=→"SEL output file refnum":refnum<file>)  [unwired: 2 in, 1 out]
    }
    frame #5 {
      # "Инициализация источника"
      n205 = call <instrlib>:"niDCPower Initialize.vi"("resource name"="DC POWER 1") -> ("error out"=w331:errorcluster, "instrument handle out"=w332:refnum<k15>)  [unwired: 3 in, 6 out]
      n206 = call <instrlib>:"niDCPower Initialize.vi"("resource name"="DC POWER 2") -> ("error out"=w328:errorcluster, "instrument handle out"=w329:refnum<k15>)  [unwired: 3 in, 6 out]
      n207 = call <instrlib>:"niDCPower Configure Voltage Level.vi"("error in (no error)"=w331, "voltage level"=0.0, "channel name"="0,1", "instrument handle"=w332) -> ("error out"=w320:errorcluster, "instrument handle out"=w322:refnum<k15>)  [unwired: 6 in]
      n208 = call <instrlib>:"niDCPower Configure Voltage Level.vi"("error in (no error)"=w328, "voltage level"=0.0, "channel name"="0,1", "instrument handle"=w329) -> ("error out"=w319:errorcluster, "instrument handle out"=w321:refnum<k15>)  [unwired: 6 in]
    }
    frame #6 {
      n209 = local read "NI Scope Status"() -> (w333:bool)
      n210 = case shown="True" w333 {
        tunnel: [refnum<k15> refnum ("instrument handle out") w341] -> w335
        tunnel: [errorcluster {"status"=FALSE, "code"=0, "source"=""} ("error out") w340] -> w334
        frame False {
          n211 = Wait (ms)(milliseconds to wait=u32 1) -> ()  [unwired: 1 out]
          n212 = property on="NI Scope Tab" class="TabCtl (strict)"("DisabledEnum"=T5."Disabled and Grayed Out" ("Disabled")) -> ()  [unwired: 2 in, 2 out]
        }
        frame True {
          n213 = stacked-sequence {
            tunnel: [_ w373] -> w341
            tunnel: [_ w372] -> w340
            frame #0 {
              w352 = "\t"
              # "Инициализация файла SEU"
              n214 = local read "Образец №"() -> (w357:string)
              n215 = Build Path(base path="SEU path", name or relative path=w357) -> (appended path=w367:path)
              n216 = Get Date/Time In Seconds() -> (seconds since 1Jan1904=w363:timestamp)
              n217 = call <vilib>:"Check if File or Folder Exists.vi"("path"=w367) -> ("file or folder exists?"=w366:bool, "dup path"=w365:path)  [unwired: 8 in, 1 out]
              n218 = Format Date/Time String(time format string (%c)="SEU %d %m %y %H.%M.%S", seconds (now)=w363) -> (date/time string=w362:string)  [unwired: 1 in]
              n219 = case shown="True" w366 {
                tunnel: w365 -> [w369 w370]
                tunnel: [w368 w370] -> w364
                frame False {
                  n220 = Create Folder(path (use dialog)=w369) -> (created path=w368:path)  [unwired: 2 in, 2 out]
                }
                frame True {
                }
              }
              n221 = Concatenate Strings(w362, ".xls" ("string")) -> (w361:string)
              n222 = Build Path(base path=w364, name or relative path=w361) -> (appended path=w360:path)
              n223 = Open/Create/Replace File(file path (use dialog)=w360, operation (0:open)=T4."open or create", access (0:read/write)=enum16{"read/write", "read-only", "write-only"}."read/write") -> (refnum out=w359:refnum<file>)  [unwired: 3 in, 2 out]
              n224 = property on="NI Scope Tab" class="TabCtl (strict)"("DisabledEnum"=T5."Enabled" ("Disabled")) -> ()  [unwired: 2 in, 2 out]
              n225 = Set File Position(refnum=w359, from (0:start)=enum16{"start", "end", "current"}."end") -> (refnum out=w356:refnum<file>)  [unwired: 2 in, 1 out]
              n226 = Format Into String(initial string=w356, "Time" ("string"), w352, "Voltage, V" ("string"), w352, "Current, A" ("string"), w352, "SEU counter" ("string"), w352, "!!!" ("input 7"), "\r\n") -> (resulting string=→"SEU output file refnum":refnum<file>)  [unwired: 2 in, 1 out]
            }
            frame #1 {
              w378 = 2 items=["None"=1, "Auto Trigger"=2] ("Triggering:Trigger Modifier")
              w376 = u32 0 items=["1 mega ohm"=0, "50 ohms"=2] ("Input Impedance")
              w374 = FALSE  # Reset Device
              n227 = call <instrlib>:"niScope Initialize.vi"("resource name"="NI Scope", "reset device"=w374, "error in"="NI Scope error in") -> ("instrument handle"=w385:refnum<k15>, "error out"=w384:errorcluster)  [unwired: 11 in]
              n228 = call <instrlib>:"niScope Configure Chan Characteristics.vi"("instrument handle"=w385, "channels"="0" ("Channel Name"), "input impedance"=w376, "maximum input frequency"=20000000.0 ("Maximum Input Frequency"), "error in"=w384) -> ("instrument handle out"=w387:refnum<k15>, "error out"=w383:errorcluster)  [unwired: 9 in]
              n229 = call <instrlib>:"niScope Configure Horizontal Timing.vi"("instrument handle"=w387, "enforce realtime"=TRUE ("Enforce Realtime"), "min sample rate"=250000000.0 ("Min Sample Rate"), "reference position"=50.0 ("Reference\nPosition"), "error in"=w383, "min record length"=1000000 ("Min Record Length")) -> ("instrument handle out"=w386:refnum<k15>, "error out"=w372:errorcluster)  [unwired: 8 in]
              n230 = property on="Property Node" class="niScope"(reference=w386, "Trigger Modifier"=w378) -> (reference out=w373:refnum<k15>)  [unwired: 1 in, 1 out]
            }
          }
        }
      }
    }
    frame #7 {
      # "Инициализация DMM"
      n231 = local read "NI DMM 1 Status"() -> (w396:bool)
      n232 = local read "NI DMM 2 Status"() -> (w395:bool)
      n233 = local read "NI DMM 3 Status"() -> (w391:bool)
      n234 = case shown="True" w391 {
        tunnel: [refnum<k15> refnum ("instrument handle out") w402] -> w389
        tunnel: [errorcluster {"status"=FALSE, "code"=0, "source"=""} ("error out") w403] -> w390
        frame False {
          n235 = property on="NI DMM 3 Tab" class="TabCtl (strict)"("DisabledEnum"=T5."Disabled and Grayed Out" ("Disabled")) -> ()  [unwired: 2 in, 2 out]
        }
        frame True {
          n236 = local read "NI DMM 3 Option Return"() -> (w404:enum32{"Ampermeter button", "Ohmmeter button"})
          n237 = property on="NI DMM 3 Tab" class="TabCtl (strict)"("DisabledEnum"=T5."Enabled" ("Disabled")) -> ()  [unwired: 2 in, 2 out]
          n238 = stacked-sequence {
            tunnel: w404 -> [w405 _]
            tunnel: [_ w459] -> w403
            tunnel: [_ w458] -> w402
            frame #0 {
              n239 = case shown="\"Ampermeter button\", Default" w405 {
                frame "Ampermeter button", Default {
                  # "Инициализация файла SEU"
                  n240 = local read "Образец №"() -> (w421:string)
                  n241 = Build Path(base path="NI DMM 3 Ampermeter path", name or relative path=w421) -> (appended path=w428:path)
                  n242 = Get Date/Time In Seconds() -> (seconds since 1Jan1904=w424:timestamp)
                  n243 = call <vilib>:"Check if File or Folder Exists.vi"("path"=w428) -> ("file or folder exists?"=w427:bool, "dup path"=w426:path)  [unwired: 8 in, 1 out]
                  n244 = Format Date/Time String(time format string (%c)="NI DMM 3 %d %m %y %H.%M.%S", seconds (now)=w424) -> (date/time string=w423:string)  [unwired: 1 in]
                  n245 = case shown="True" w427 {
                    tunnel: w426 -> [w430 w431]
                    tunnel: [w429 w431] -> w425
                    frame False {
                      n246 = Create Folder(path (use dialog)=w430) -> (created path=w429:path)  [unwired: 2 in, 2 out]
                    }
                    frame True {
                    }
                  }
                  n247 = Concatenate Strings(w423, ".xls" ("string")) -> (w422:string)
                  n248 = Build Path(base path=w425, name or relative path=w422) -> (appended path=w407:path)
                  n249 = Open/Create/Replace File(file path (use dialog)=w407, operation (0:open)=T4."open or create", access (0:read/write)=enum16{"read/write", "read-only", "write-only"}."read/write") -> (refnum out=w418:refnum<file>)  [unwired: 3 in, 2 out]
                  n250 = Set File Position(refnum=w418, from (0:start)=enum16{"start", "end", "current"}."end") -> (refnum out=w410:refnum<file>)  [unwired: 2 in, 1 out]
                  n251 = Format Into String(initial string=w410, "Time" ("string"), "\t", "Current, A" ("string"), "\r\n") -> (resulting string=→"NI DMM 3 Current output file":refnum<file>)  [unwired: 2 in, 1 out]
                  n252 = local write "NI DMM 3 Tab"(enum32{"Amp", "Ohm", "System Panel"}."Amp" ("NI DMM 2 Tab")) -> ()
                }
                frame "Ohmmeter button" {
                  n253 = local read "Образец №"() -> (w447:string)
                  n254 = Build Path(base path="NI DMM 3 Ohmmeter path", name or relative path=w447) -> (appended path=w454:path)
                  n255 = Get Date/Time In Seconds() -> (seconds since 1Jan1904=w450:timestamp)
                  n256 = call <vilib>:"Check if File or Folder Exists.vi"("path"=w454) -> ("file or folder exists?"=w453:bool, "dup path"=w452:path)  [unwired: 8 in, 1 out]
                  n257 = Format Date/Time String(time format string (%c)="NI DMM 3 %d %m %y %H.%M.%S", seconds (now)=w450) -> (date/time string=w449:string)  [unwired: 1 in]
                  n258 = case shown="True" w453 {
                    tunnel: w452 -> [w456 w457]
                    tunnel: [w455 w457] -> w451
                    frame False {
                      n259 = Create Folder(path (use dialog)=w456) -> (created path=w455:path)  [unwired: 2 in, 2 out]
                    }
                    frame True {
                    }
                  }
                  n260 = Concatenate Strings(w449, ".xls" ("string")) -> (w448:string)
                  n261 = Build Path(base path=w451, name or relative path=w448) -> (appended path=w433:path)
                  n262 = Open/Create/Replace File(file path (use dialog)=w433, operation (0:open)=T4."open or create", access (0:read/write)=enum16{"read/write", "read-only", "write-only"}."read/write") -> (refnum out=w444:refnum<file>)  [unwired: 3 in, 2 out]
                  n263 = Set File Position(refnum=w444, from (0:start)=enum16{"start", "end", "current"}."end") -> (refnum out=w436:refnum<file>)  [unwired: 2 in, 1 out]
                  n264 = Format Into String(initial string=w436, "Time" ("string"), "\t", "Current, A" ("string"), "\r\n") -> (resulting string=→"NI DMM 3 Resistance output file":refnum<file>)  [unwired: 2 in, 1 out]
                  n265 = local write "NI DMM 3 Tab"(enum32{"Amp", "Ohm", "System Panel"}."Ohm" ("NI DMM 2 Tab")) -> ()
                }
              }
            }
            frame #1 {
              n266 = call <instrlib>:"niDMM Initialize.vi"("error in (no error)"="NI DMM 3 error in", "Instrument Descriptor"="NI DMM 3") -> ("error out"=w459:errorcluster, "instrument handle out"=w458:refnum<k15>)  [unwired: 8 in]
            }
          }
        }
      }
      "NI DMM 3 error out" <- w390
      n267 = case shown="True" w396 {
        tunnel: [refnum<k15> refnum ("instrument handle out") w530] -> w394
        tunnel: [errorcluster {"status"=FALSE, "code"=0, "source"=""} ("error out") w529] -> w393
        frame False {
          n268 = property on="NI DMM 1 Tab" class="TabCtl (strict)"("DisabledEnum"=T5."Disabled and Grayed Out" ("Disabled")) -> ()  [unwired: 2 in, 2 out]
        }
        frame True {
          n269 = local read "NI DMM 1 Option Return"() -> (w532:enum32{"Ampermeter button", "Ohmmeter button"})
          n270 = property on="NI DMM 1 Tab" class="TabCtl (strict)"("DisabledEnum"=T5."Enabled" ("Disabled")) -> ()  [unwired: 2 in, 2 out]
          n271 = stacked-sequence {
            tunnel: w532 -> [w533 _]
            tunnel: [_ w587] -> w530
            tunnel: [_ w586] -> w529
            frame #0 {
              n272 = case shown="\"Ampermeter button\", Default" w533 {
                frame "Ampermeter button", Default {
                  n273 = local read "Образец №"() -> (w549:string)
                  n274 = Build Path(base path="NI DMM 1 Ampermeter path", name or relative path=w549) -> (appended path=w556:path)
                  n275 = Get Date/Time In Seconds() -> (seconds since 1Jan1904=w552:timestamp)
                  n276 = call <vilib>:"Check if File or Folder Exists.vi"("path"=w556) -> ("file or folder exists?"=w555:bool, "dup path"=w554:path)  [unwired: 8 in, 1 out]
                  n277 = Format Date/Time String(time format string (%c)="NI DMM 1 %d %m %y %H.%M.%S", seconds (now)=w552) -> (date/time string=w551:string)  [unwired: 1 in]
                  n278 = case shown="True" w555 {
                    tunnel: w554 -> [w558 w559]
                    tunnel: [w557 w559] -> w553
                    frame False {
                      n279 = Create Folder(path (use dialog)=w558) -> (created path=w557:path)  [unwired: 2 in, 2 out]
                    }
                    frame True {
                    }
                  }
                  n280 = Concatenate Strings(w551, ".xls" ("string")) -> (w550:string)
                  n281 = Build Path(base path=w553, name or relative path=w550) -> (appended path=w535:path)
                  n282 = Open/Create/Replace File(file path (use dialog)=w535, operation (0:open)=T4."open or create", access (0:read/write)=enum16{"read/write", "read-only", "write-only"}."read/write") -> (refnum out=w546:refnum<file>)  [unwired: 3 in, 2 out]
                  n283 = local write "NI DMM 1 Tab"(enum32{"Amp", "Ohm", "System Panel"}."Amp" ("NI DMM 1 Tab")) -> ()
                  n284 = Set File Position(refnum=w546, from (0:start)=enum16{"start", "end", "current"}."end") -> (refnum out=w538:refnum<file>)  [unwired: 2 in, 1 out]
                  n285 = Format Into String(initial string=w538, "Time" ("string"), "\t", "Current, A" ("string"), "\r\n") -> (resulting string=→"NI DMM 1 Current output file":refnum<file>)  [unwired: 2 in, 1 out]
                }
                frame "Ohmmeter button" {
                  # "Инициализация файла SEU"
                  n286 = local read "Образец №"() -> (w575:string)
                  n287 = Build Path(base path="NI DMM 1 Ohmmeter path", name or relative path=w575) -> (appended path=w582:path)
                  n288 = Get Date/Time In Seconds() -> (seconds since 1Jan1904=w578:timestamp)
                  n289 = call <vilib>:"Check if File or Folder Exists.vi"("path"=w582) -> ("file or folder exists?"=w581:bool, "dup path"=w580:path)  [unwired: 8 in, 1 out]
                  n290 = Format Date/Time String(time format string (%c)="NI DMM 1 %d %m %y %H.%M.%S", seconds (now)=w578) -> (date/time string=w577:string)  [unwired: 1 in]
                  n291 = case shown="False" w581 {
                    tunnel: w580 -> [w584 w585]
                    tunnel: [w583 w585] -> w579
                    frame False {
                      n292 = Create Folder(path (use dialog)=w584) -> (created path=w583:path)  [unwired: 2 in, 2 out]
                    }
                    frame True {
                    }
                  }
                  n293 = Concatenate Strings(w577, ".xls" ("string")) -> (w576:string)
                  n294 = Build Path(base path=w579, name or relative path=w576) -> (appended path=w561:path)
                  n295 = Open/Create/Replace File(file path (use dialog)=w561, operation (0:open)=T4."open or create", access (0:read/write)=enum16{"read/write", "read-only", "write-only"}."read/write") -> (refnum out=w572:refnum<file>)  [unwired: 3 in, 2 out]
                  n296 = local write "NI DMM 1 Tab"(enum32{"Amp", "Ohm", "System Panel"}."Ohm" ("NI DMM 1 Tab")) -> ()
                  n297 = Set File Position(refnum=w572, from (0:start)=enum16{"start", "end", "current"}."end") -> (refnum out=w564:refnum<file>)  [unwired: 2 in, 1 out]
                  n298 = Format Into String(initial string=w564, "Time" ("string"), "\t", "Current, A" ("string"), "\r\n") -> (resulting string=→"NI DMM 1 Resistance output file":refnum<file>)  [unwired: 2 in, 1 out]
                }
              }
            }
            frame #1 {
              n299 = call <instrlib>:"niDMM Initialize.vi"("error in (no error)"="NI DMM 1 error in", "Instrument Descriptor"="NI DMM 1") -> ("error out"=w586:errorcluster, "instrument handle out"=w587:refnum<k15>)  [unwired: 8 in]
            }
          }
        }
      }
      "NI DMM 1 error out" <- w393
      n300 = case shown="True" w395 {
        tunnel: [refnum<k15> refnum ("instrument handle out") w465] -> w397
        tunnel: [errorcluster {"status"=FALSE, "code"=0, "source"=""} ("error out") w466] -> w392
        frame False {
          n301 = property on="NI DMM 2 Tab" class="TabCtl (strict)"("DisabledEnum"=T5."Disabled and Grayed Out" ("Disabled")) -> ()  [unwired: 2 in, 2 out]
        }
        frame True {
          n302 = local read "NI DMM 2 Option Return"() -> (w468:enum32{"Ampermeter button", "Ohmmeter button"})
          n303 = property on="NI DMM 2 Tab" class="TabCtl (strict)"("DisabledEnum"=T5."Enabled" ("Disabled")) -> ()  [unwired: 2 in, 2 out]
          n304 = stacked-sequence {
            tunnel: w468 -> [w469 _]
            tunnel: [_ w523] -> w466
            tunnel: [_ w522] -> w465
            frame #0 {
              n305 = case shown="\"Ampermeter button\", Default" w469 {
                frame "Ampermeter button", Default {
                  n306 = local read "Образец №"() -> (w485:string)
                  n307 = Build Path(base path="NI DMM 2 Ampermeter path", name or relative path=w485) -> (appended path=w492:path)
                  n308 = Get Date/Time In Seconds() -> (seconds since 1Jan1904=w488:timestamp)
                  n309 = call <vilib>:"Check if File or Folder Exists.vi"("path"=w492) -> ("file or folder exists?"=w491:bool, "dup path"=w490:path)  [unwired: 8 in, 1 out]
                  n310 = Format Date/Time String(time format string (%c)="NI DMM 2 %d %m %y %H.%M.%S", seconds (now)=w488) -> (date/time string=w487:string)  [unwired: 1 in]
                  n311 = case shown="True" w491 {
                    tunnel: w490 -> [w494 w495]
                    tunnel: [w493 w495] -> w489
                    frame False {
                      n312 = Create Folder(path (use dialog)=w494) -> (created path=w493:path)  [unwired: 2 in, 2 out]
                    }
                    frame True {
                    }
                  }
                  n313 = Concatenate Strings(w487, ".xls" ("string")) -> (w486:string)
                  n314 = Build Path(base path=w489, name or relative path=w486) -> (appended path=w471:path)
                  n315 = Open/Create/Replace File(file path (use dialog)=w471, operation (0:open)=T4."open or create", access (0:read/write)=enum16{"read/write", "read-only", "write-only"}."read/write") -> (refnum out=w482:refnum<file>)  [unwired: 3 in, 2 out]
                  n316 = Set File Position(refnum=w482, from (0:start)=enum16{"start", "end", "current"}."end") -> (refnum out=w474:refnum<file>)  [unwired: 2 in, 1 out]
                  n317 = Format Into String(initial string=w474, "Time" ("string"), "\t", "Current, A" ("string"), "\r\n") -> (resulting string=→"NI DMM 2 Current output file":refnum<file>)  [unwired: 2 in, 1 out]
                  n318 = local write "NI DMM 2 Tab"(enum32{"Amp", "Ohm", "System Panel"}."Amp" ("NI DMM 2 Tab")) -> ()
                }
                frame "Ohmmeter button" {
                  # "Инициализация файла SEU"
                  n319 = local read "Образец №"() -> (w511:string)
                  n320 = Build Path(base path="NI DMM 2 Ohmmeter path", name or relative path=w511) -> (appended path=w518:path)
                  n321 = Get Date/Time In Seconds() -> (seconds since 1Jan1904=w514:timestamp)
                  n322 = call <vilib>:"Check if File or Folder Exists.vi"("path"=w518) -> ("file or folder exists?"=w517:bool, "dup path"=w516:path)  [unwired: 8 in, 1 out]
                  n323 = Format Date/Time String(time format string (%c)="NI DMM 2 %d %m %y %H.%M.%S", seconds (now)=w514) -> (date/time string=w513:string)  [unwired: 1 in]
                  n324 = case shown="True" w517 {
                    tunnel: w516 -> [w520 w521]
                    tunnel: [w519 w521] -> w515
                    frame False {
                      n325 = Create Folder(path (use dialog)=w520) -> (created path=w519:path)  [unwired: 2 in, 2 out]
                    }
                    frame True {
                    }
                  }
                  n326 = Concatenate Strings(w513, ".xls" ("string")) -> (w512:string)
                  n327 = Build Path(base path=w515, name or relative path=w512) -> (appended path=w497:path)
                  n328 = Open/Create/Replace File(file path (use dialog)=w497, operation (0:open)=T4."open or create", access (0:read/write)=enum16{"read/write", "read-only", "write-only"}."read/write") -> (refnum out=w508:refnum<file>)  [unwired: 3 in, 2 out]
                  n329 = Set File Position(refnum=w508, from (0:start)=enum16{"start", "end", "current"}."end") -> (refnum out=w500:refnum<file>)  [unwired: 2 in, 1 out]
                  n330 = Format Into String(initial string=w500, "Time" ("string"), "\t", "Current, A" ("string"), "\r\n") -> (resulting string=→"NI DMM 2 Resistance output file":refnum<file>)  [unwired: 2 in, 1 out]
                  n331 = local write "NI DMM 2 Tab"(enum32{"Amp", "Ohm", "System Panel"}."Ohm" ("NI DMM 2 Tab")) -> ()
                }
              }
            }
            frame #1 {
              n332 = call <instrlib>:"niDMM Initialize.vi"("error in (no error)"="NI DMM 2 error in", "Instrument Descriptor"="NI DMM 2") -> ("error out"=w523:errorcluster, "instrument handle out"=w522:refnum<k15>)  [unwired: 8 in]
            }
          }
        }
      }
      "NI DMM 2 error out" <- w392
    }
    frame #8 {
      n333 = local read "Ophir 1 Status"() -> (w590:bool)
      n334 = case shown="True" w590 {
        frame False {
          n335 = property on="Ophir 1 Tab" class="TabCtl (strict)"("DisabledEnum"=T5."Disabled and Grayed Out" ("Disabled")) -> ()  [unwired: 2 in, 2 out]
        }
        frame True {
          n336 = call "Ophir InitCom.vi"("GPIB Address (default 10)"="Ophir 1 GPIB Address (10)", "Communication (default USB 0)"="Ophir 1 Select Communication Protocol", "USB Channel number (default 0)"="Ophir 1 usb channel", "Port Number (default 2)"="Ophir 1 Port Number (default 2)", "error in (no error)"="Ophir 1 error in (no error)", "Baud Rate (3:9600)"="Ophir 1 Baud Rate (3:9600)") -> ("dup Visa Session"=w598:refnum<visa-resource-name>, "error out"=w597:errorcluster)  [unwired: 1 out]
          n337 = call "Ophir InstrInfo.vi"("Visa Session"=w598, "error in (no error)"=w597) -> ("dup Visa Session"=w611:refnum<visa-resource-name>, "Instrument Info"=w607:string, "error out"=w609:errorcluster)
          n338 = call "Ophir HeadInfo.vi"("Visa Session"=w611, "error in (no error)"=w609) -> ("error out"=w608:errorcluster, "dup Visa Session"=w610:refnum<visa-resource-name>, "Head Info"=w606:string)  [unwired: 6 out]
          n339 = call "Ophir InfoStrings.vi"("error in (no error)"=w608, "Head Info"=w606, "Instrument Info"=w607) -> ("error out"=w605:errorcluster, "Strings Array"=w604:string[])
          n340 = property on="Ophir 1 Info" class="Ring (strict)"("Strings []"=w604) -> ()  [unwired: 2 in, 2 out]
          n341 = property on="Ophir 1 Tab" class="TabCtl (strict)"("DisabledEnum"=T5."Enabled" ("Disabled")) -> ()  [unwired: 2 in, 2 out]
          n342 = call "Ophir ConfigDevice.vi"("Visa Session"=w610, "Measure Choice (0:Power)"=u16 0, "error in (no error)"=w605) -> ("dup Visa Session"=→"Ophir 1 dup Visa Session":refnum<visa-resource-name>, "OK ?"=→"Ophir 1 Initialization":bool, "error out"=→"Ophir 1 error out":errorcluster)  [unwired: 1 out]
        }
      }
    }
    frame #9 {
      n343 = local read "Ophir 2 Status"() -> (w613:bool)
      n344 = case shown="True" w613 {
        frame False {
          n345 = property on="Ophir 2 Tab" class="TabCtl (strict)"("DisabledEnum"=T5."Disabled and Grayed Out" ("Disabled")) -> ()  [unwired: 2 in, 2 out]
        }
        frame True {
          n346 = call "Ophir InitCom.vi"("GPIB Address (default 10)"="Ophir 2 GPIB Address (10)", "Communication (default USB 0)"="Ophir 2 Select Communication Protocol", "USB Channel number (default 0)"="Ophir 2 usb channel", "Port Number (default 2)"="Ophir 2 Port Number (default 2)", "error in (no error)"="Ophir 2 error in (no error)", "Baud Rate (3:9600)"="Ophir 2 Baud Rate (3:9600)") -> ("dup Visa Session"=w621:refnum<visa-resource-name>, "error out"=w620:errorcluster)  [unwired: 1 out]
          n347 = call "Ophir InstrInfo.vi"("Visa Session"=w621, "error in (no error)"=w620) -> ("dup Visa Session"=w634:refnum<visa-resource-name>, "Instrument Info"=w630:string, "error out"=w632:errorcluster)
          n348 = call "Ophir HeadInfo.vi"("Visa Session"=w634, "error in (no error)"=w632) -> ("error out"=w631:errorcluster, "dup Visa Session"=w633:refnum<visa-resource-name>, "Head Info"=w629:string)  [unwired: 6 out]
          n349 = call "Ophir InfoStrings.vi"("error in (no error)"=w631, "Head Info"=w629, "Instrument Info"=w630) -> ("error out"=w628:errorcluster, "Strings Array"=w627:string[])
          n350 = property on="Ophir 2 Info" class="Ring (strict)"("Strings []"=w627) -> ()  [unwired: 2 in, 2 out]
          n351 = property on="Ophir 2 Tab" class="TabCtl (strict)"("DisabledEnum"=T5."Enabled" ("Disabled")) -> ()  [unwired: 2 in, 2 out]
          n352 = call "Ophir ConfigDevice.vi"("Visa Session"=w633, "Measure Choice (0:Power)"=u16 0, "error in (no error)"=w628) -> ("dup Visa Session"=→"Ophir 2 dup Visa Session":refnum<visa-resource-name>, "OK ?"=→"Ophir 2 Initialization":bool, "error out"=→"Ophir 2 error out":errorcluster)  [unwired: 1 out]
        }
      }
    }
    frame #10 {
      n353 = local read "Stepper Motor Status"() -> (w639:bool)
      n354 = case shown="True" w639 {
        tunnel: [_ w648] -> w638
        tunnel: [_ w647] -> w637
        tunnel: [_ w646] -> w636
        frame False {
          n355 = property on="Stepper Motor Control" class="TabCtl (strict)"("DisabledEnum"=T5."Disabled and Grayed Out" ("Disabled")) -> ()  [unwired: 2 in, 2 out]
          n356 = property on="Table Tab" class="TabCtl (strict)"("DisabledEnum"=T5."Disabled and Grayed Out" ("Disabled")) -> ()  [unwired: 2 in, 2 out]
        }
        frame True {
          n357 = property on="Stepper Motor Control" class="TabCtl (strict)"("DisabledEnum"=T5."Enabled" ("Disabled")) -> ()  [unwired: 2 in, 2 out]
          n358 = constructor class="NetTcpUrl"("host"="localhost", "port"=u32 8001, "urlPath"="AmateurStepperMotorInternal") -> (reference out=w659:refnum<k24>)  [unwired: 3 in, 5 out]
          n359 = constructor class="AmateurStepperMotorWcfClient"("serviceUrl"=w659) -> (reference out=w660:refnum<k24>)  [unwired: 3 in, 3 out]
          n360 = invoke class="AmateurStepperMotorWcfClient" method="RefreshParameters"(reference=w660) -> (reference out=w649:refnum<k24>)  [unwired: 2 in, 2 out]
          n361 = property on="Table Tab" class="TabCtl (strict)"("DisabledEnum"=T5."Enabled" ("Disabled")) -> ()  [unwired: 2 in, 2 out]
          n362 = property on="Glass Meas" class="Bool (strict)"("DisabledEnum"=T5."Enabled" ("Disabled")) -> ()  [unwired: 2 in, 2 out]
          n363 = property on="Погнали!" class="Bool (strict)"("DisabledEnum"=T5."Enabled" ("Disabled")) -> ()  [unwired: 2 in, 2 out]
          n364 = property class="AmateurStepperMotorWcfClient"(reference=w649, "Speed"="Speed", "StepDivisor"="StepDivisor", "StepMultiplicationFactor"="StepMultiplicationFactor", "AccelerationTime"=0.5, "DecelerationTime"=0.5, "HoldOn"=FALSE) -> (reference out=w648:refnum<k24>, "Position"=w647:dbl, "PositioningPrecision"=w646:dbl)  [unwired: 1 in, 1 out]
        }
      }
    }
    frame #11 {
      w661 = TRUE ("Boolean")
      "Ready Status" <- w661
    }
  }
  n365 = case shown="True" w13 {
    tunnel: w12 -> [_ w667]
    tunnel: w11 -> [_ w666]
    tunnel: w10 -> [_ w665]
    tunnel: w3 -> [_ _]
    frame False {
    }
    frame True {
      n366 = flat-sequence {
        frame #0 {
          n367 = local read "WL 455 Ref"() -> (w688:dbl)
          n368 = local read "WL 808 Ref"() -> (w687:dbl)
          n369 = local read "WL 1550 Ref"() -> (w686:dbl)
          n370 = while {
            shift-right: ["Save Glass Log Data"] -> _
            shift-left: FALSE ("Погнали!") -> [w698]
            shift-right: [w695] -> _
            shift-left: w688 -> [w691]
            shift-right: [w694] -> _
            shift-left: w687 -> [w692]
            shift-right: [w693] -> _
            shift-left: w686 -> [w690]
            stop <- w696 stop-if-true
            n371 = Wait (ms)(milliseconds to wait=u32 1) -> ()  [unwired: 1 out]
            n372 = Greater?(x="Save Glass Log Data", y=w698) -> (0:w699:bool)
            n373 = case shown="True" w699 {
              tunnel: [w703 w712] -> w695
              tunnel: [w702 w711] -> w694
              tunnel: [w701 w710] -> w693
              tunnel: w692 -> [w702 w709]
              tunnel: w691 -> [w703 w708]
              tunnel: w690 -> [w701 w707]
              frame False {
              }
              frame True {
                n374 = flat-sequence {
                  tunnel: w708 -> [w720]
                  tunnel: w709 -> [w719]
                  tunnel: w707 -> [w718]
                  tunnel: [w716] -> w706
                  tunnel: [w715] -> w705
                  tunnel: [w714] -> w704
                  tunnel: [w909] -> w712
                  tunnel: [w908] -> w711
                  tunnel: [w907] -> w710
                  tunnel: w706 -> [w909]
                  tunnel: w705 -> [w908]
                  tunnel: w704 -> [w907]
                  frame #0 {
                    "Save Glass Log Done" <- FALSE ("Save Glass Log Done")
                  }
                  frame #1 {
                    n375 = local read "Glass Meas Cycle Running"() -> (w721:bool)
                    n376 = case shown="False" w721 {
                      tunnel: w720 -> [w728 w773]
                      tunnel: w719 -> [w727 w772]
                      tunnel: w718 -> [w726 w771]
                      tunnel: "Set Last Meas As Ref" -> [w725 _]
                      tunnel: [w724 w773] -> w716
                      tunnel: [w723 w772] -> w715
                      tunnel: [w722 w771] -> w714
                      frame False {
                        n377 = local read "WL-i"() -> (w729:i32)
                        n378 = case shown="False" w725 {
                          tunnel: w728 -> [_ w742]
                          tunnel: w727 -> [_ w741]
                          tunnel: w726 -> [_ w740]
                          tunnel: [w739 w742] -> w724
                          tunnel: [w738 w741] -> w723
                          tunnel: [w737 w740] -> w722
                          frame False {
                            n379 = local read "WL 455"() -> (w739:dbl)
                            n380 = local read "WL 808"() -> (w738:dbl)
                            n381 = local read "WL 1550"() -> (w737:dbl)
                          }
                          frame True {
                            n382 = local write "WL 455 Ref"(w742) -> ()
                            n383 = local write "WL 808 Ref"(w741) -> ()
                            n384 = local write "WL 1550 Ref"(w740) -> ()
                          }
                        }
                        n385 = Wait (ms)(milliseconds to wait=u32 5) -> ()  [unwired: 1 out]
                        n386 = local read "Single Meas Output File"() -> (w733:refnum<file>)
                        n387 = local read "CH Data String"() -> (w734:string)
                        n388 = local read "All Cur Data String"() -> (w735:string)
                        n389 = local read "Meas Time String"() -> (w736:string)
                        n390 = local read "Av Cur Data String"() -> (w731:string)
                        n391 = case shown="0, Default" w729 {
                          tunnel: [w745 w751 w766] -> w730
                          tunnel: w731 -> [w745 w751 w760]
                          frame 0, Default {
                            n392 = local read "WL 455 Ref"() -> (w743:dbl)
                            n393 = local read "WL 455"() -> (w746:dbl)
                            n394 = Divide(x=w746, y=w743) -> (x/y=w748:dbl)
                            n395 = Number To Fractional String(number=w748, precision (6)=i16 3) -> (F-format string=w744:string)  [unwired: 2 in]
                            n396 = local write "WL 455 Absolute/Reference"(w744) -> ()
                          }
                          frame 1 {
                            n397 = local read "WL 808 Ref"() -> (w749:dbl)
                            n398 = local read "WL 808"() -> (w754:dbl)
                            n399 = Divide(x=w754, y=w749) -> (x/y=w753:dbl)
                            n400 = Number To Fractional String(number=w753, precision (6)=i16 3) -> (F-format string=w750:string)  [unwired: 2 in]
                            n401 = local write "WL 808 Absolute/Reference"(w750) -> ()
                          }
                          frame 2 {
                            w757 = "\t"
                            n402 = local read "Add Log Remark"() -> (w758:bool)
                            n403 = case shown="True" w758 {
                              tunnel: ["\r\n" w770] -> w756
                              frame False {
                              }
                              frame True {
                                n404 = local read "Log Remark"() -> (w768:string)
                                n405 = Concatenate Strings(w768, "\r\n") -> (w770:string)
                              }
                            }
                            n406 = local read "WL 455 Absolute/Reference"() -> (w762:string)
                            n407 = local read "WL 808 Absolute/Reference"() -> (w761:string)
                            n408 = local read "WL 1550 Ref"() -> (w755:dbl)
                            n409 = local read "WL 1550"() -> (w765:dbl)
                            n410 = Divide(x=w765, y=w755) -> (x/y=w764:dbl)
                            n411 = Number To Fractional String(number=w764, precision (6)=i16 3) -> (F-format string=w759:string)  [unwired: 2 in]
                            n412 = Concatenate Strings(w760, w762, w757, w761, w757, w759, w757, w756) -> (w766:string)
                            n413 = local write "WL 1550 Absolute/Reference"(w759) -> ()
                          }
                        }
                        n414 = Format Into String(initial string=w733, w734, w735, w736, w730) -> ()  [unwired: 2 in, 2 out]
                      }
                      frame True {
                        n415 = local read "WL-i"() -> (w778:i32)
                        n416 = local read "Куда едем?"() -> (w777:T1)
                        n417 = Wait (ms)(milliseconds to wait=u32 1) -> ()  [unwired: 1 out]
                        n418 = Equal?(x=w777, y=T1."Калибровка") -> (x = y?=w776:bool)
                        n419 = case shown="False" w776 {
                          tunnel: w778 -> [w779 w859]
                          tunnel: w777 -> [w780 _]
                          frame False {
                            n420 = stacked-sequence {
                              tunnel: w780 -> [w783 w820]
                              tunnel: w779 -> [w782 w821]
                              frame #0 {
                                n421 = case shown="2" w782 {
                                tunnel: [w797 w803 w815] -> w788
                                tunnel: [w794 w798 w807] -> w781
                                frame 0, Default {
                                n422 = local read "Av Cur Data String"() -> (w797:string)
                                n423 = local read "WL 455 Ref"() -> (w792:dbl)
                                n424 = local read "WL 455"() -> (w793:dbl)
                                n425 = Divide(x=w793, y=w792) -> (x/y=w796:dbl)
                                n426 = Number To Fractional String(number=w796, precision (6)=i16 3) -> (F-format string=w794:string)  [unwired: 2 in]
                                "WL 455 Absolute/Reference" <- w794
                                }
                                frame 1 {
                                n427 = local read "Av Cur Data String"() -> (w803:string)
                                n428 = local read "WL 808"() -> (w802:dbl)
                                n429 = local read "WL 808 Ref"() -> (w801:dbl)
                                n430 = Divide(x=w802, y=w801) -> (x/y=w800:dbl)
                                n431 = Number To Fractional String(number=w800, precision (6)=i16 3) -> (F-format string=w798:string)  [unwired: 2 in]
                                "WL 808 Absolute/Reference" <- w798
                                }
                                frame 2 {
                                w806 = "\t"
                                n432 = local read "Add Log Remark"() -> (w804:bool)
                                n433 = local read "Av Cur Data String"() -> (w810:string)
                                n434 = local read "WL 455 Absolute/Reference"() -> (w809:string)
                                n435 = local read "WL 808 Absolute/Reference"() -> (w808:string)
                                n436 = case shown="True" w804 {
                                tunnel: ["\r\n" w819] -> w805
                                frame False {
                                }
                                frame True {
                                n437 = local read "Log Remark"() -> (w817:string)
                                n438 = Concatenate Strings(w817, "\r\n") -> (w819:string)
                                }
                                }
                                n439 = local read "WL 1550 Ref"() -> (w813:dbl)
                                n440 = local read "WL 1550"() -> (w814:dbl)
                                n441 = Divide(x=w814, y=w813) -> (x/y=w812:dbl)
                                n442 = Number To Fractional String(number=w812, precision (6)=i16 3) -> (F-format string=w807:string)  [unwired: 2 in]
                                "WL 1550 Absolute/Reference" <- w807
                                n443 = Concatenate Strings(w810, w809, w806, w808, w806, w807, w806, w805) -> (w815:string)
                                }
                                }
                                n444 = local read "CH Data String"() -> (w791:string)
                                n445 = local read "Meas Time String"() -> (w790:string)
                                n446 = local read "Glass Meas Path"() -> (w789:refnum<file>)
                                n447 = Format Into String(initial string=w789, w791, w790, w788) -> ()  [unwired: 2 in, 2 out]
                                n448 = To Long Integer(number=w783) -> (32bit integer=w785:i32)
                                n449 = Increment(x=w782) -> (x+1=w784:i32)
                                n450 = Replace Array Subset(array="Glass Table", new element=w781, index (row)=w785, index (col)=w784) -> (w786:string[][])
                                n451 = local write "Glass Table"(w786) -> ()
                              }
                              frame #1 {
                                n452 = local read "Av Cur Data String"() -> (w823:string)
                                n453 = case shown="2" w821 {
                                tunnel: w820 -> [_ _ w838]
                                tunnel: [w828 w829 w837] -> w822
                                tunnel: w823 -> [w828 w829 w833]
                                frame 0, Default {
                                }
                                frame 1 {
                                }
                                frame 2 {
                                w830 = "\t"
                                n454 = local read "WL 1550 Absolute/Reference"() -> (w836:string)
                                n455 = local read "WL 455 Absolute/Reference"() -> (w834:string)
                                n456 = local read "WL 808 Absolute/Reference"() -> (w835:string)
                                n457 = Equal?(x=w838, y=T1."Четвертое стекло") -> (x = y?=w840:bool)
                                n458 = case shown="True" w840 {
                                tunnel: ["\t" w844] -> w839
                                frame False {
                                }
                                frame True {
                                n459 = case shown="True" "Add Log Remark" {
                                selector: "Add Log Remark" -> [_ w849]
                                tunnel: ["\r\n" w850] -> w844
                                tunnel: [w846 w848] -> w843
                                frame False {
                                n460 = local read "Add Log Remark"() -> (w846:bool)
                                }
                                frame True {
                                n461 = Not(x=w849) -> (.not. x?=w848:bool)
                                n462 = Concatenate Strings("Log Remark", "\r\n") -> (w850:string)
                                }
                                }
                                n463 = local write "Add Log Remark"(w843) -> ()
                                }
                                }
                                n464 = Concatenate Strings(w834, w830, w835, w830, w836, w830) -> (w832:string)
                                n465 = Concatenate Strings(w833, w832) -> (w831:string)
                                n466 = Concatenate Strings(w831, w839) -> (w837:string)
                                }
                                }
                                n467 = local read "Glass Full Log Output File"() -> (w826:refnum<file>)
                                n468 = local read "CH Data String"() -> (w824:string)
                                n469 = local read "All Cur Data String"() -> (w825:string)
                                n470 = local read "Meas Time String"() -> (w827:string)
                                n471 = Format Into String(initial string=w826, w824, w825, w827, w822) -> ()  [unwired: 2 in, 2 out]
                              }
                            }
                          }
                          frame True {
                            n472 = local read "CH Data String"() -> (w867:string)
                            n473 = local read "Meas Time String"() -> (w866:string)
                            n474 = local read "Glass 1 Output File"() -> (w865:refnum<file>)
                            n475 = local read "Glass 2 Output File"() -> (w864:refnum<file>)
                            n476 = local read "Glass 3 Output File"() -> (w863:refnum<file>)
                            n477 = local read "Glass 4 Output File"() -> (w862:refnum<file>)
                            n478 = local read "Glass Full Log Output File"() -> (w857:refnum<file>)
                            n479 = local read "CH Data String"() -> (w855:string)
                            n480 = local read "All Cur Data String"() -> (w856:string)
                            n481 = local read "Meas Time String"() -> (w858:string)
                            n482 = local read "Av Cur Data String"() -> (w854:string)
                            n483 = case shown="0, Default" w859 {
                              tunnel: [w871 w882 w890] -> w860
                              tunnel: w854 -> [w869 w881 w891]
                              tunnel: [w869 w881 w890] -> w853
                              frame 0, Default {
                                n484 = local read "Av Cur Data String"() -> (w871:string)
                                n485 = flat-sequence {
                                tunnel: [w872] -> w870
                                tunnel: w870 -> [w878]
                                tunnel: [w874] -> w868
                                frame #0 {
                                n486 = local read "WL 455 Ref"() -> (w872:dbl)
                                n487 = Wait (ms)(milliseconds to wait=u32 1) -> ()  [unwired: 1 out]
                                }
                                frame #1 {
                                n488 = local read "WL 455"() -> (w877:dbl)
                                "WL 455 Ref" <- w877
                                n489 = Divide(x=w878, y=w877) -> (x/y=w875:dbl)
                                n490 = Number To Fractional String(number=w875, precision (6)=i16 3) -> (F-format string=w874:string)  [unwired: 2 in]
                                }
                                }
                                n491 = local write "WL 455 Absolute/Reference"(w868) -> ()
                              }
                              frame 1 {
                                n492 = local read "Av Cur Data String"() -> (w882:string)
                                n493 = flat-sequence {
                                tunnel: [w883] -> w880
                                tunnel: w880 -> [w887]
                                tunnel: [w885] -> w879
                                frame #0 {
                                n494 = local read "WL 808 Ref"() -> (w883:dbl)
                                n495 = Wait (ms)(milliseconds to wait=u32 1) -> ()  [unwired: 1 out]
                                }
                                frame #1 {
                                n496 = local read "WL 808"() -> (w886:dbl)
                                "WL 808 Ref" <- w886
                                n497 = Divide(x=w887, y=w886) -> (x/y=w888:dbl)
                                n498 = Number To Fractional String(number=w888, precision (6)=i16 3) -> (F-format string=w885:string)  [unwired: 2 in]
                                }
                                }
                                n499 = local write "WL 808 Absolute/Reference"(w879) -> ()
                              }
                              frame 2 {
                                n500 = flat-sequence {
                                tunnel: [w893] -> w892
                                tunnel: w892 -> [w897]
                                tunnel: w891 -> [w902]
                                tunnel: [w901] -> w890
                                frame #0 {
                                n501 = local read "WL 1550 Ref"() -> (w893:dbl)
                                n502 = Wait (ms)(milliseconds to wait=u32 1) -> ()  [unwired: 1 out]
                                }
                                frame #1 {
                                n503 = local read "WL 1550"() -> (w896:dbl)
                                "WL 1550 Ref" <- w896
                                n504 = Divide(x=w897, y=w896) -> (x/y=w898:dbl)
                                n505 = Number To Fractional String(number=w898, precision (6)=i16 3) -> (F-format string=w895:string)  [unwired: 2 in]
                                n506 = local write "WL 1550 Absolute/Reference"(w895) -> ()
                                }
                                frame #2 {
                                w900 = "\t"
                                w903 = "\t"
                                n507 = local read "WL 455 Absolute/Reference"() -> (w906:string)
                                n508 = local read "WL 808 Absolute/Reference"() -> (w905:string)
                                n509 = local read "WL 1550 Absolute/Reference"() -> (w904:string)
                                n510 = Concatenate Strings(w902, w906, w903, w905, w903, w904, w900, w900) -> (w901:string)
                                }
                                }
                              }
                            }
                            n511 = Concatenate Strings(w867, w866, w860) -> (w861:string)
                            n512 = Format Into String(initial string=w865, w861) -> ()  [unwired: 2 in, 2 out]
                            n513 = Format Into String(initial string=w864, w861) -> ()  [unwired: 2 in, 2 out]
                            n514 = Format Into String(initial string=w863, w861) -> ()  [unwired: 2 in, 2 out]
                            n515 = Format Into String(initial string=w862, w861) -> ()  [unwired: 2 in, 2 out]
                            n516 = Format Into String(initial string=w857, w855, w856, w858, w853) -> ()  [unwired: 2 in, 2 out]
                          }
                        }
                      }
                    }
                  }
                  frame #2 {
                    n517 = local write "Save Glass Log Done"(TRUE ("Save Glass Log Done")) -> ()
                  }
                }
              }
            }
            n518 = local read "System Stop"() -> (w696:bool)
          }
        }
        frame #1 {
          n519 = local read "Glass Full Log Output File"() -> (w912:refnum<file>)
          n520 = local read "Glass 1 Output File"() -> (w916:refnum<file>)
          n521 = local read "Glass 2 Output File"() -> (w915:refnum<file>)
          n522 = local read "Glass 3 Output File"() -> (w914:refnum<file>)
          n523 = local read "Glass 4 Output File"() -> (w913:refnum<file>)
          n524 = local read "Single Meas Output File"() -> (w911:refnum<file>)
          n525 = Close File(refnum=w912) -> ()  [unwired: 1 in, 2 out]
          n526 = Close File(refnum=w916) -> ()  [unwired: 1 in, 2 out]
          n527 = Close File(refnum=w915) -> ()  [unwired: 1 in, 2 out]
          n528 = Close File(refnum=w914) -> ()  [unwired: 1 in, 2 out]
          n529 = Close File(refnum=w913) -> ()  [unwired: 1 in, 2 out]
          n530 = Close File(refnum=w911) -> ()  [unwired: 1 in, 2 out]
        }
      }
      n531 = while {
        stop <- w918 stop-if-true
        n532 = Wait (ms)(milliseconds to wait=u32 1) -> ()  [unwired: 1 out]
        n533 = case shown="True" "Glass Meas Cycle" {
          frame False {
          }
          frame True {
            n534 = while {
              stop <- w923 stop-if-true
              n535 = stacked-sequence {
                tunnel: [_ _ _ w986] -> w921
                frame #0 {
                  n536 = flat-sequence {
                    tunnel: [w932] -> w927
                    tunnel: [w931] -> w924
                    tunnel: [w935] -> w928
                    tunnel: w927 -> [w935]
                    tunnel: [w934] -> w925
                    tunnel: w924 -> [w934]
                    tunnel: [w939] -> w929
                    tunnel: w928 -> [w939]
                    tunnel: [w938] -> w926
                    tunnel: w925 -> [w938]
                    tunnel: w929 -> [w943]
                    tunnel: w926 -> [w942]
                    frame #0 {
                      n537 = local read "P2 CH1 Used"() -> (w932:bool)
                      n538 = local read "P2 CH1"() -> (w931:bool)
                      "Glass Meas Cycle Running" <- TRUE ("Cycle Running")
                    }
                    frame #1 {
                      n539 = local write "Meas Progress Bar"(u8 0 ("Measuering Progress Bar")) -> ()
                      n540 = property on="Glass Meas" class="Bool (strict)"("DisabledEnum"=T5."Disabled and Grayed Out" ("Disabled")) -> ()  [unwired: 2 in, 2 out]
                      n541 = property on="Погнали!" class="Bool (strict)"("DisabledEnum"=T5."Disabled and Grayed Out" ("Disabled")) -> ()  [unwired: 2 in, 2 out]
                    }
                    frame #2 {
                      n542 = local write "P2 CH1 Used"(TRUE ("P1 CH0 Used")) -> ()
                      n543 = local write "P2 CH1"(TRUE ("P1 CH0")) -> ()
                    }
                    frame #3 {
                      n544 = Not(x=w943) -> (.not. x?=w945:bool)
                      n545 = Not(x=w942) -> (.not. x?=w944:bool)
                      n546 = Or(x=w945, y=w944) -> (x .or. y?=w946:bool)
                      n547 = case shown="True" w946 {
                        frame False {
                        }
                        frame True {
                          n548 = Wait (ms)(milliseconds to wait=u32 100) -> ()  [unwired: 1 out]
                        }
                      }
                    }
                  }
                }
                frame #1 {
                  n549 = for {
                    N: 5 -> [_]
                    i -> [w949]
                    n550 = flat-sequence {
                      tunnel: w949 -> [w950]
                      tunnel: w949 -> [w959]
                      tunnel: w949 -> [w973]
                      frame #0 {
                        n551 = local write "Куда едем?"(w950) -> ()
                      }
                      frame #1 {
                        n552 = local write "Погнали!"(TRUE ("Погнали!")) -> ()
                        n553 = Wait (ms)(milliseconds to wait=u32 200) -> ()  [unwired: 1 out]
                      }
                      frame #2 {
                        n554 = while {
                          stop <- w954 stop-if-true
                          n555 = local read "System Stop"() -> (w955:bool)
                          n556 = local read "Готово"() -> (w956:bool)
                          n557 = Wait (ms)(milliseconds to wait=u32 1) -> ()  [unwired: 1 out]
                          n558 = Compound Arithmetic op=OR(w956, w955) -> (w954:bool)
                        }
                      }
                      frame #3 {
                        n559 = local write "Погнали!"(FALSE ("Погнали!")) -> ()
                        n560 = Wait (ms)(milliseconds to wait=u32 200) -> ()  [unwired: 1 out]
                      }
                      frame #4 {
                        n561 = case shown="1" w959 {
                          frame 0, Default {
                          }
                          frame 1 {
                            n562 = local read "Glass 1 Output File"() -> (→"Glass Num Output File":refnum<file>)
                          }
                          frame 2 {
                            n563 = local read "Glass 2 Output File"() -> (w961:refnum<file>)
                            n564 = local write "Glass Num Output File"(w961) -> ()
                          }
                          frame 3 {
                            n565 = local read "Glass 3 Output File"() -> (w962:refnum<file>)
                            n566 = local write "Glass Num Output File"(w962) -> ()
                          }
                          frame 4 {
                            n567 = local read "Glass 4 Output File"() -> (w963:refnum<file>)
                            n568 = local write "Glass Num Output File"(w963) -> ()
                          }
                        }
                      }
                      frame #5 {
                        n569 = local write "Glass Meas"(TRUE ("Glass Measure")) -> ()
                        n570 = Wait (ms)(milliseconds to wait=u32 50) -> ()  [unwired: 1 out]
                      }
                      frame #6 {
                        n571 = while {
                          stop <- w969 stop-if-true
                          n572 = local read "Meas Running"() -> (w966:bool)
                          n573 = local read "System Stop"() -> (w970:bool)
                          n574 = Wait (ms)(milliseconds to wait=u32 1) -> ()  [unwired: 1 out]
                          n575 = Not(x=w966) -> (.not. x?=w967:bool)
                          n576 = Compound Arithmetic op=OR(w967, w970) -> (w969:bool)
                        }
                      }
                      frame #7 {
                        n577 = local write "Glass Meas"(FALSE ("Glass Measure")) -> ()
                      }
                      frame #8 {
                        n578 = Increment(x=w973) -> (x+1=w974:i32)
                        n579 = Multiply(x=w974, y=18) -> (x*y=w975:i32)
                        n580 = To Unsigned Byte Integer(number=w975) -> (unsigned 8bit integer=w976:u8)
                        n581 = local write "Meas Progress Bar"(w976) -> ()
                        n582 = Wait (ms)(milliseconds to wait=u32 100) -> ()  [unwired: 1 out]
                      }
                    }
                  }
                }
                frame #2 {
                  n583 = flat-sequence {
                    frame #0 {
                      n584 = local write "Куда едем?"(T1."Калибровка" ("Куда едем?")) -> ()
                    }
                    frame #1 {
                      n585 = local write "Погнали!"(TRUE ("Погнали!")) -> ()
                    }
                    frame #2 {
                      n586 = Wait (ms)(milliseconds to wait=u32 100) -> ()  [unwired: 1 out]
                    }
                    frame #3 {
                      n587 = local write "Погнали!"(FALSE ("Погнали!")) -> ()
                    }
                    frame #4 {
                      n588 = while {
                        stop <- w982 stop-if-true
                        n589 = local read "System Stop"() -> (w983:bool)
                        n590 = local read "Готово"() -> (w984:bool)
                        n591 = Compound Arithmetic op=OR(w984, w983) -> (w982:bool)
                      }
                    }
                    frame #5 {
                      n592 = Wait (ms)(milliseconds to wait=u32 200) -> ()  [unwired: 1 out]
                    }
                  }
                }
                frame #3 {
                  n593 = flat-sequence {
                    tunnel: [w998] -> w986
                    frame #0 {
                      n594 = local read "Glass Meas Cycle"() -> (w987:bool)
                      n595 = case shown="False" w987 {
                        frame False {
                          n596 = local write "P2 CH1 Used"(FALSE ("P1 CH0 Used")) -> ()
                        }
                        frame True {
                        }
                      }
                    }
                    frame #1 {
                      n597 = local read "Num of Meas"() -> (w990:u32)
                      n598 = local read "Meas Progress Bar"() -> (w994:u8)
                      n599 = Increment(x=w990) -> (x+1=→"Num of Meas":u32)
                      n600 = Add(x=w994, y=u8 10) -> (x+y=w993:u8)
                      n601 = local write "Meas Progress Bar"(w993) -> ()
                      n602 = Wait (ms)(milliseconds to wait=u32 100) -> ()  [unwired: 1 out]
                    }
                    frame #2 {
                      n603 = local write "Glass Meas Cycle Running"(FALSE ("Glass Meas Cycle Running")) -> ()
                      n604 = property on="Glass Meas" class="Bool (strict)"("DisabledEnum"=T5."Enabled" ("Disabled")) -> ()  [unwired: 2 in, 2 out]
                      n605 = property on="Погнали!" class="Bool (strict)"("DisabledEnum"=T5."Enabled" ("Disabled")) -> ()  [unwired: 2 in, 2 out]
                    }
                    frame #3 {
                      n606 = local read "Glass Meas Cycle"() -> (w999:bool)
                      n607 = Not(x=w999) -> (.not. x?=w998:bool)
                    }
                  }
                }
              }
              n608 = Wait (ms)(milliseconds to wait=u32 1) -> ()  [unwired: 1 out]
              n609 = local read "System Stop"() -> (w922:bool)
              n610 = Or(x=w921, y=w922) -> (x .or. y?=w923:bool)
            }
          }
        }
        n611 = local read "System Stop"() -> (w918:bool)
      }
      n612 = while {
        shift-right: ["Glass Meas"] -> _
        shift-left: FALSE ("Glass Measure") -> [w1001]
        stop <- w1004 stop-if-true
        n613 = Wait (ms)(milliseconds to wait=u32 1) -> ()  [unwired: 1 out]
        n614 = Greater?(x="Glass Meas", y=w1001) -> (0:w1002:bool)
        n615 = case shown="True" w1002 {
          frame False {
          }
          frame True {
            n616 = stacked-sequence {
              frame #0 {
                n617 = flat-sequence {
                  frame #0 {
                    w1005 = T5."Disabled and Grayed Out" ("Disabled")
                    n618 = property on="P1 CH0 Used" class="Bool (strict)"("DisabledEnum"=w1005) -> ()  [unwired: 2 in, 2 out]
                    n619 = property on="P1 CH1 Used" class="Bool (strict)"("DisabledEnum"=w1005) -> ()  [unwired: 2 in, 2 out]
                    n620 = property on="P1 CH2 Used" class="Bool (strict)"("DisabledEnum"=w1005) -> ()  [unwired: 2 in, 2 out]
                    n621 = property on="P2 CH0 Used" class="Bool (strict)"("DisabledEnum"=w1005) -> ()  [unwired: 2 in, 2 out]
                    n622 = property on="P2 CH1 Used" class="Bool (strict)"("DisabledEnum"=w1005) -> ()  [unwired: 2 in, 2 out]
                    n623 = property on="P2 CH2 Used" class="Bool (strict)"("DisabledEnum"=w1005) -> ()  [unwired: 2 in, 2 out]
                    "Meas Running" <- TRUE ("Done")
                  }
                  frame #1 {
                    n624 = local write "P1 CH2 Used"(TRUE ("P1 CH0 Used")) -> ()
                    n625 = local write "P1 CH2"(TRUE ("P1 CH2")) -> ()
                    n626 = Wait (ms)(milliseconds to wait=u32 100) -> ()  [unwired: 1 out]
                  }
                }
              }
              frame #1 {
                n627 = for {
                  N: 3 -> [_]
                  i -> [w1012]
                  n628 = flat-sequence {
                    tunnel: w1012 -> [w1017]
                    tunnel: w1012 -> [w1021]
                    tunnel: w1012 -> [w1030]
                    tunnel: [w1028] -> w1011
                    tunnel: [w1048] -> w1015
                    tunnel: [w1047] -> w1014
                    tunnel: [w1046] -> w1013
                    tunnel: w1012 -> [w1044]
                    tunnel: w1011 -> [w1043]
                    tunnel: w1015 -> [w1083]
                    tunnel: w1014 -> [w1081]
                    tunnel: w1013 -> [w1072]
                    tunnel: w1012 -> [w1070]
                    tunnel: w1012 -> [w1089]
                    frame #0 {
                      n629 = case shown="0, Default" w1017 {
                        frame 0, Default {
                          n630 = local write "P1 CH0 Used"(TRUE ("P1 CH0 Used")) -> ()
                        }
                        frame 1 {
                          n631 = local write "P1 CH1 Used"(TRUE ("P1 CH0 Used")) -> ()
                        }
                        frame 2 {
                          n632 = local write "P2 CH0 Used"(TRUE ("P1 CH0 Used")) -> ()
                        }
                      }
                      n633 = Wait (ms)(milliseconds to wait=u32 100) -> ()  [unwired: 1 out]
                    }
                    frame #1 {
                      n634 = case shown="2" w1021 {
                        frame 0, Default {
                          n635 = local write "P1 CH0"(TRUE ("P1 CH0")) -> ()
                          n636 = Wait (ms)(milliseconds to wait=u32 2000) -> ()  [unwired: 1 out]
                        }
                        frame 1 {
                          n637 = local write "P1 CH1"(TRUE ("P1 CH0")) -> ()
                          n638 = Wait (ms)(milliseconds to wait=u32 2000) -> ()  [unwired: 1 out]
                        }
                        frame 2 {
                          n639 = local write "P2 CH0"(TRUE ("P1 CH0")) -> ()
                          n640 = Wait (ms)(milliseconds to wait=u32 12000) -> ()  [unwired: 1 out]
                        }
                      }
                    }
                    frame #2 {
                      w1036 = "\t"
                      w1031 = i16 12 ("precision (6)")
                      n641 = case shown="0, Default" w1030 {
                        tunnel: [w1038 w1040 w1042] -> w1035
                        tunnel: [w1037 w1039 w1041] -> w1033
                        frame 0, Default {
                          n642 = local read "P1 CH0, V"() -> (w1038:dbl)
                          n643 = local read "P1 CH0_cur, A"() -> (w1037:dbl)
                        }
                        frame 1 {
                          n644 = local read "P1 CH1_cur, A"() -> (w1039:dbl)
                          n645 = local read "P1 CH1, V"() -> (w1040:dbl)
                        }
                        frame 2 {
                          n646 = local read "P2 CH0_cur, A"() -> (w1041:dbl)
                          n647 = local read "P2 CH0, V"() -> (w1042:dbl)
                        }
                      }
                      n648 = local read "Glass Meas Cycle Running"() -> (w1028:bool)
                      n649 = Number To Fractional String(number=w1035, precision (6)=w1031) -> (F-format string=w1034:string)  [unwired: 2 in]
                      n650 = Number To Fractional String(number=w1033, precision (6)=w1031) -> (F-format string=w1032:string)  [unwired: 2 in]
                      n651 = Concatenate Strings(w1034, w1036, w1032, w1036) -> (→"CH Data String":string)
                    }
                    frame #3 {
                      w1047 = 5
                      n652 = for {
                        N: w1047 -> [_]
                        shift-right: [w1064] -> w1046
                        shift-left: "" -> [w1063]
                        shift-right: [w1060] -> w1048
                        shift-left: 0.0 -> [w1058]
                        tunnel: w1044 -> [w1057]
                        n653 = case shown="0, Default" w1057 {
                          tunnel: [w1066 w1067 w1068] -> w1059
                          frame 0, Default {
                            n654 = local read "DMM 1 Real Current"() -> (w1066:dbl)
                          }
                          frame 1 {
                            n655 = local read "DMM 2 Real Current"() -> (w1067:dbl)
                          }
                          frame 2 {
                            n656 = local read "DMM 3 Real Current"() -> (w1068:dbl)
                          }
                        }
                        n657 = Wait (ms)(milliseconds to wait="Meas Wait") -> ()  [unwired: 1 out]
                        n658 = Add(x=w1058, y=w1059) -> (x+y=w1060:dbl)
                        n659 = Number To Fractional String(number=w1059, precision (6)=i16 12) -> (F-format string=w1062:string)  [unwired: 2 in]
                        n660 = Concatenate Strings(w1063, w1062, "\t") -> (w1064:string)
                      }
                      n661 = case shown="False" w1043 {
                        tunnel: w1044 -> [w1050 _]
                        frame False {
                          n662 = local read "Set Last Meas As Ref"() -> (w1051:bool)
                          n663 = case shown="False" w1051 {
                            tunnel: w1050 -> [w1052 _]
                            frame False {
                              n664 = case shown="0, Default" w1052 {
                                frame 0, Default {
                                n665 = local read "WL 455"() -> (w1053:dbl)
                                n666 = local write "WL 455 Ref"(w1053) -> ()
                                }
                                frame 1 {
                                n667 = local read "WL 808"() -> (w1054:dbl)
                                n668 = local write "WL 808 Ref"(w1054) -> ()
                                }
                                frame 2 {
                                n669 = local read "WL 1550"() -> (w1055:dbl)
                                n670 = local write "WL 1550 Ref"(w1055) -> ()
                                }
                              }
                            }
                            frame True {
                            }
                          }
                        }
                        frame True {
                        }
                      }
                    }
                    frame #4 {
                      n671 = local read "Glass Meas Cycle Running"() -> (w1071:bool)
                      n672 = To Double Precision Float(number=w1081) -> (double precision float=w1082:dbl)
                      n673 = Divide(x=w1083, y=w1082) -> (x/y=w1080:dbl)
                      n674 = Wait (ms)(milliseconds to wait=u32 1) -> ()  [unwired: 1 out]
                      n675 = Number To Fractional String(number=w1080, precision (6)=i16 12) -> (F-format string=w1075:string)  [unwired: 2 in]
                      n676 = case shown="0, Default" w1070 {
                        tunnel: w1080 -> [w1085 w1086 w1087]
                        frame 0, Default {
                          "WL 455" <- w1085
                        }
                        frame 1 {
                          "WL 808" <- w1086
                        }
                        frame 2 {
                          "WL 1550" <- w1087
                        }
                      }
                      n677 = case shown="True" w1071 {
                        frame False {
                        }
                        frame True {
                          n678 = local read "Glass Num Output File"() -> (→"Glass Meas Path":refnum<file>)
                        }
                      }
                      n679 = Concatenate Strings(w1075, "\t") -> (→"Av Cur Data String":string)
                      n680 = Format Date/Time String(time format string (%c)="%H:%M:%S:%3u") -> (date/time string=w1078:string)  [unwired: 2 in]
                      n681 = Concatenate Strings(w1078, "\t") -> (→"Meas Time String":string)
                      "All Cur Data String" <- w1072
                    }
                    frame #5 {
                      n682 = case shown="0, Default" w1089 {
                        frame 0, Default {
                          n683 = local write "P1 CH0 Used"(FALSE ("P1 CH0 Used")) -> ()
                        }
                        frame 1 {
                          n684 = local write "P1 CH1 Used"(FALSE ("P1 CH0 Used")) -> ()
                        }
                        frame 2 {
                          n685 = local write "P2 CH0 Used"(FALSE ("P1 CH0 Used")) -> ()
                        }
                      }
                      n686 = Wait (ms)(milliseconds to wait=u32 500) -> ()  [unwired: 1 out]
                    }
                    frame #6 {
                      n687 = local write "Save Glass Log Data"(TRUE ("Save Glass Log Data")) -> ()
                      n688 = Wait (ms)(milliseconds to wait=u32 50) -> ()  [unwired: 1 out]
                    }
                    frame #7 {
                      n689 = while {
                        stop <- w1097 stop-if-true
                        n690 = local read "System Stop"() -> (w1098:bool)
                        n691 = local read "Save Glass Log Done"() -> (w1099:bool)
                        n692 = Wait (ms)(milliseconds to wait=u32 1) -> ()  [unwired: 1 out]
                        n693 = Compound Arithmetic op=OR(w1099, w1098) -> (w1097:bool)
                      }
                    }
                    frame #8 {
                      n694 = local write "Save Glass Log Data"(FALSE ("Save Glass Log Data")) -> ()
                    }
                  }
                  "WL-i" <- w1012
                }
              }
              frame #2 {
                n695 = flat-sequence {
                  frame #0 {
                    n696 = local write "P1 CH2 Used"(FALSE ("P1 CH0 Used")) -> ()
                    n697 = Wait (ms)(milliseconds to wait=u32 100) -> ()  [unwired: 1 out]
                  }
                  frame #1 {
                    w1103 = T5."Enabled" ("Disabled")
                    n698 = local write "Meas Running"(FALSE ("Done")) -> ()
                    n699 = property on="P1 CH0 Used" class="Bool (strict)"("DisabledEnum"=w1103) -> ()  [unwired: 2 in, 2 out]
                    n700 = property on="P1 CH1 Used" class="Bool (strict)"("DisabledEnum"=w1103) -> ()  [unwired: 2 in, 2 out]
                    n701 = property on="P1 CH2 Used" class="Bool (strict)"("DisabledEnum"=w1103) -> ()  [unwired: 2 in, 2 out]
                    n702 = property on="P2 CH0 Used" class="Bool (strict)"("DisabledEnum"=w1103) -> ()  [unwired: 2 in, 2 out]
                    n703 = property on="P2 CH1 Used" class="Bool (strict)"("DisabledEnum"=w1103) -> ()  [unwired: 2 in, 2 out]
                    n704 = property on="P2 CH2 Used" class="Bool (strict)"("DisabledEnum"=w1103) -> ()  [unwired: 2 in, 2 out]
                  }
                }
              }
            }
          }
        }
        n705 = local read "System Stop"() -> (w1004:bool)
      }
      n706 = while {
        tunnel: w667 -> [w1151]
        shift-right: [w1141] -> _
        shift-left: FALSE ("Погнали!") -> [w1152]
        tunnel: [w1150] -> w668
        shift-right: [w1148] -> _
        shift-left: w666 -> [w1149]
        tunnel: w665 -> [w1147]
        stop <- w1144 stop-if-true
        n707 = Wait (ms)(milliseconds to wait=u32 1) -> ()  [unwired: 1 out]
        n708 = case shown="True" "Погнали!" {
          selector: "Погнали!" -> [w1153 _]
          tunnel: [w1153 w1154] -> w1141
          frame False {
          }
          frame True {
            n709 = local read "P2 CH1"() -> (w1155:bool)
            n710 = case shown="True" w1155 {
              selector: w1155 -> [_ w1159]
              tunnel: [w1156 w1159] -> w1154
              frame False {
                n711 = One Button Dialog(message="Power up the stepper motor.") -> (true=w1157:bool)  [unwired: 1 in]
                n712 = Not(x=w1157) -> (.not. x?=w1156:bool)
                n713 = local write "Погнали!"(w1156) -> ()
              }
              frame True {
              }
            }
          }
        }
        n714 = local read "System Stop"() -> (w1144:bool)
        n715 = case shown="\"Первое стекло\"" "Куда едем?" {
          tunnel: [0.0 -1550.0 -2700.0 -4100.0 -5250.0] -> w1145
          frame "Калибровка", Default {
          }
          frame "Первое стекло" {
          }
          frame "Второе стекло" {
          }
          frame "Третье стекло" {
          }
          frame "Четвертое стекло" {
          }
        }
        n716 = Greater?(x=w1141, y=w1152) -> (0:w1140:bool)
        n717 = case shown="True" w1140 {
          tunnel: w1145 -> [_ w1172]
          tunnel: w1151 -> [w1166 w1171]
          tunnel: [w1166 w1170] -> w1150
          tunnel: w1149 -> [w1165 _]
          tunnel: [w1165 w1169] -> w1148
          tunnel: w1147 -> [_ w1168]
          frame False {
            n718 = Wait (ms)(milliseconds to wait=u32 1) -> ()  [unwired: 1 out]
            "Текущая позиция" <- w1165
          }
          frame True {
            n719 = while {
              tunnel: w1172 -> [w1177]
              tunnel: w1171 -> [w1180]
              tunnel: [w1174] -> w1170
              tunnel: [w1179] -> w1169
              tunnel: w1168 -> [w1176]
              stop <- w1178 stop-if-true
              n720 = invoke class="AmateurStepperMotorWcfClient" method="GoTo"(reference=w1180, "destinationPosition"=w1177) -> (reference out=w1182:refnum<k24>, "GoTo"=w1183:refnum<k24>)  [unwired: 2 in, 2 out]
              n721 = invoke class="Task" method="ConfigureAwait"(reference=w1183, "continueOnCapturedContext"=FALSE) -> ()  [unwired: 2 in, 4 out]
              n722 = Wait (ms)(milliseconds to wait=u32 1) -> ()  [unwired: 1 out]
              n723 = while {
                tunnel: [w1186] -> w1179
                tunnel: w1182 -> [w1194]
                tunnel: [w1193] -> w1175
                tunnel: [w1185] -> w1178
                tunnel: w1177 -> [w1191]
                tunnel: w1176 -> [w1189]
                stop <- w1185 stop-if-true
                n724 = property class="AmateurStepperMotorWcfClient"(reference=w1194) -> (reference out=w1193:refnum<k24>, "Position"=w1186:dbl)  [unwired: 1 in, 1 out]
                n725 = Subtract(x=w1186, y=w1191) -> (x-y=w1192:dbl)
                n726 = Wait (ms)(milliseconds to wait=u32 1) -> ()  [unwired: 1 out]
                n727 = Absolute Value(x=w1192) -> (abs(x)=w1190:dbl)
                n728 = Less Or Equal?(x=w1190, y=w1189) -> (x <= y?=w1188:bool)
                n729 = local write "Текущая позиция"(w1186) -> ()
                n730 = Or(x=w1188, y="Стоп GoTo") -> (x .or. y?=w1185:bool)
                "Готово" <- w1185
              }
              n731 = invoke class="AmateurStepperMotorWcfClient" method="Stop"(reference=w1175) -> (reference out=w1174:refnum<k24>)  [unwired: 2 in, 2 out]
            }
          }
        }
      }
      n732 = while {
        stop <- w674 stop-if-true
        n733 = Wait (ms)(milliseconds to wait=u32 1) -> ()  [unwired: 1 out]
        n734 = case shown="True" "Clear Table" {
          frame False {
          }
          frame True {
            n735 = for {
              N: 4 -> [_]
              i -> [w677]
              n736 = for {
                N: 3 -> [_]
                tunnel: w677 -> [w679]
                i -> [w682]
                n737 = Increment(x=w679) -> (x+1=w680:i32)
                n738 = local read "Glass Table"() -> (w684:string[][])
                n739 = Increment(x=w682) -> (x+1=w681:i32)
                n740 = Replace Array Subset(array=w684, new element="" ("new element/subarray"), index (row)=w680, index (col)=w681) -> (w683:string[][])
                n741 = local write "Glass Table"(w683) -> ()
              }
            }
          }
        }
        n742 = local read "System Stop"() -> (w674:bool)
      }
      n743 = while {
        shift-right: [w1105] -> _
        shift-left: 0 ("t") -> [w1106]
        stop <- w1109 stop-if-true
        n744 = Wait (ms)(milliseconds to wait=u32 5) -> ()  [unwired: 1 out]
        n745 = case shown="True" "Тест" {
          tunnel: w1106 -> [w1112 w1119]
          tunnel: [w1112 w1116] -> w1105
          frame False {
          }
          frame True {
            n746 = flat-sequence {
              tunnel: w1119 -> [w1121]
              tunnel: [w1120] -> w1114
              tunnel: [w1126] -> w1115
              tunnel: w1114 -> [w1126]
              tunnel: [w1128] -> w1117
              tunnel: w1115 -> [w1128]
              tunnel: [w1129] -> w1118
              tunnel: w1117 -> [w1129]
              tunnel: w1118 -> [w1134]
              tunnel: [w1132] -> w1113
              tunnel: [w1139] -> w1116
              tunnel: w1113 -> [w1139]
              frame #0 {
                n747 = while {
                  tunnel: w1121 -> [w1124]
                  tunnel: [w1124] -> w1120
                  stop <- w1123 stop-if-true
                  n748 = local read "Готово"() -> (w1123:bool)
                  n749 = Wait (ms)(milliseconds to wait=u32 1) -> ()  [unwired: 1 out]
                }
              }
              frame #1 {
                n750 = local write "Куда едем?"(w1126) -> ()
                n751 = Wait (ms)(milliseconds to wait=u32 500) -> ()  [unwired: 1 out]
              }
              frame #2 {
                n752 = local write "Погнали!"(TRUE ("Погнали!")) -> ()
              }
              frame #3 {
                n753 = Wait (ms)(milliseconds to wait=u32 50) -> ()  [unwired: 1 out]
              }
              frame #4 {
                n754 = local write "Погнали!"(FALSE ("Погнали!")) -> ()
                n755 = Equal?(x=4, y=w1134) -> (x = y?=w1136:bool)
                n756 = Increment(x=w1134) -> (x+1=w1133:i32)
                n757 = Select(t=0, s=w1136, f=w1133) -> (s? t:f=w1132:i32)
              }
              frame #5 {
                n758 = Wait (ms)(milliseconds to wait=u32 50) -> ()  [unwired: 1 out]
              }
            }
          }
        }
        n759 = local read "System Stop"() -> (w1108:bool)
        n760 = Or(x=w1108, y="Стоп_тест") -> (x .or. y?=w1109:bool)
      }
      n761 = invoke class="AmateurStepperMotorWcfClient" method="Stop"(reference=w668) -> (reference out=w671:refnum<k24>, "Stop"=w672:refnum<k24>)  [unwired: 2 in, 1 out]
      n762 = invoke class="Task" method="Wait"(reference=w672) -> ()  [unwired: 2 in, 3 out]
      n763 = property class="AmateurStepperMotorWcfClient"(reference=w671, "HoldOn"=FALSE) -> (reference out=w670:refnum<k24>)  [unwired: 1 in, 1 out]
      n764 = invoke class="AmateurStepperMotorWcfClient" method="Dispose"(reference=w670) -> ()  [unwired: 2 in, 3 out]
    }
  }
  n765 = case shown="True" w19 {
    tunnel: w25 -> [_ w1201]
    tunnel: w3 -> [_ _]
    tunnel: w22 -> [_ w1198]
    frame False {
    }
    frame True {
      n766 = local read "NI DMM 1 Option Return"() -> (w1195:enum32{"Ampermeter button", "Ohmmeter button"})
      n767 = case shown="\"Ohmmeter button\"" w1195 {
        tunnel: w1201 -> [w1206 w1252]
        tunnel: [w1205 w1251] -> w1200
        tunnel: [w1204 w1250] -> w1199
        tunnel: w1198 -> [w1203 w1253]
        tunnel: [w1202 w1249] -> w1197
        frame "Ampermeter button", Default {
          n768 = while {
            tunnel: w1206 -> [w1218]
            tunnel: [w1216] -> w1205
            tunnel: [w1215] -> w1204
            tunnel: w1203 -> [w1213]
            tunnel: [w1209] -> w1202
            stop <- w1214 stop-if-true
            n769 = flat-sequence {
              tunnel: [w1224] -> w1219
              tunnel: w1218 -> [w1222]
              tunnel: w1213 -> [w1226]
              tunnel: [w1223] -> w1212
              tunnel: w1219 -> [w1229]
              tunnel: [w1234] -> w1217
              tunnel: w1212 -> [w1233]
              tunnel: [w1232] -> w1211
              tunnel: [w1228] -> w1207
              tunnel: w1217 -> [w1239]
              tunnel: [w1240] -> w1216
              tunnel: [w1239] -> w1215
              tunnel: [w1238] -> w1214
              tunnel: w1211 -> [w1237]
              tunnel: [w1237] -> w1210
              tunnel: w1207 -> [w1236]
              frame #0 {
                w1220 = T7 6.5 items=["3 1/2"=3.5, "4 1/2"=4.5, "5 1/2"=5.5, "6 1/2"=6.5, "7 1/2"=7.5] ("Resolution in Digits")
                n770 = Fract/Exp String To Number(string="NI DMM 1 Current Range") -> (number=w1225:dbl)  [unwired: 3 in, 1 out]
                n771 = call-poly <instrlib>:"niDMM Config Measurement.vi"("Range"=w1225, "Resolution in Digits"=w1220, "error in (no error)"=w1226, "Function"=niDMM_Function."DC Current" ("Measurement Type"), "instrument handle"=w1222) -> ("error out"=w1223:errorcluster, "instrument handle out"=w1224:refnum<k15>)  [unwired: 5 in]
              }
              frame #1 {
                n772 = call <instrlib>:"niDMM Read.vi"("error in (no error)"=w1233, "instrument handle"=w1229) -> ("error out"=w1232:errorcluster, "Measurement"=w1228:dbl, "instrument handle out"=w1234:refnum<k15>)  [unwired: 7 in]
                "DMM 1 Real Current" <- w1228
                n773 = Fract/Exp String To Number(string="NI DMM 1 units") -> (number=w1230:dbl)  [unwired: 3 in, 1 out]
                n774 = Multiply(x=w1230, y=w1228) -> (x*y=→"NI DMM 1 Current" →"NI DMM 1 Current Char":dbl)
              }
              frame #2 {
                w1248 = 6
                n775 = local read "NI DMM 1 Current output file"() -> (w1241:refnum<file>)
                n776 = Format Date/Time String(time format string (%c)="%H:%M:%S:%3u") -> (date/time string=w1246:string)  [unwired: 2 in]
                n777 = Number To Fractional String(number=w1236, width (-)=w1248, precision (6)=w1248) -> (F-format string=w1243:string)  [unwired: 1 in]
                n778 = local read "System Stop"() -> (w1238:bool)
                n779 = Concatenate Strings(w1246, "\t", w1243, "\r\n") -> (w1244:string)
                n780 = Format Into String(initial string=w1241, w1244) -> (resulting string=w1240:refnum<file>)  [unwired: 2 in, 1 out]
              }
            }
            n781 = Wait (ms)(milliseconds to wait="NI DMM 1 Current Wait") -> ()  [unwired: 1 out]
            n782 = call <vilib>:"Simple Error Handler.vi"("error in (no error)"=w1210) -> ("error out"=w1209:errorcluster)  [unwired: 1 in, 7 out]
          }
        }
        frame "Ohmmeter button" {
          n783 = while {
            tunnel: w1252 -> [w1265]
            tunnel: [w1263] -> w1251
            tunnel: [w1262] -> w1250
            tunnel: w1253 -> [w1260]
            tunnel: [w1256] -> w1249
            stop <- w1261 stop-if-true
            n784 = flat-sequence {
              tunnel: [w1272] -> w1266
              tunnel: w1265 -> [w1271]
              tunnel: w1260 -> [w1270]
              tunnel: [w1269] -> w1259
              tunnel: w1266 -> [w1282]
              tunnel: [w1280] -> w1264
              tunnel: w1259 -> [w1279]
              tunnel: [w1278] -> w1258
              tunnel: [w1275] -> w1254
              tunnel: w1264 -> [w1287]
              tunnel: [w1288] -> w1263
              tunnel: [w1287] -> w1262
              tunnel: [w1286] -> w1261
              tunnel: [w1285] -> w1257
              tunnel: w1258 -> [w1285]
              tunnel: w1254 -> [w1284]
              frame #0 {
                w1274 = T7 6.5 items=["3 1/2"=3.5, "4 1/2"=4.5, "5 1/2"=5.5, "6 1/2"=6.5, "7 1/2"=7.5] ("Resolution in Digits")
                n785 = Fract/Exp String To Number(string="NI DMM 1 Resistance Range") -> (number=w1267:dbl)  [unwired: 3 in, 1 out]
                n786 = call-poly <instrlib>:"niDMM Config Measurement.vi"("Range"=w1267, "Resolution in Digits"=w1274, "error in (no error)"=w1270, "Function"=niDMM_Function."2-wire Resistance" ("Measurement Type"), "instrument handle"=w1271) -> ("error out"=w1269:errorcluster, "instrument handle out"=w1272:refnum<k15>)  [unwired: 5 in]
              }
              frame #1 {
                n787 = call <instrlib>:"niDMM Read.vi"("error in (no error)"=w1279, "instrument handle"=w1282) -> ("error out"=w1278:errorcluster, "Measurement"=w1275:dbl, "instrument handle out"=w1280:refnum<k15>)  [unwired: 7 in]
                n788 = Fract/Exp String To Number(string="NI DMM 1 Resistance units") -> (number=w1276:dbl)  [unwired: 3 in, 1 out]
                n789 = Multiply(x=w1276, y=w1275) -> (x*y=→"NI DMM 1 Resistance" →"NI DMM 1 Resistance Char":dbl)
              }
              frame #2 {
                w1289 = 12
                n790 = local read "NI DMM 1 Resistance output file"() -> (w1295:refnum<file>)
                n791 = Format Date/Time String(time format string (%c)="%H:%M:%S:%3u") -> (date/time string=w1291:string)  [unwired: 2 in]
                n792 = Number To Fractional String(number=w1284, width (-)=w1289, precision (6)=w1289) -> (F-format string=w1283:string)  [unwired: 1 in]
                n793 = Concatenate Strings(w1291, "\t", w1283, "\r\n") -> (w1293:string)
                n794 = local read "System Stop"() -> (w1286:bool)
                n795 = Format Into String(initial string=w1295, w1293) -> (resulting string=w1288:refnum<file>)  [unwired: 2 in, 1 out]
              }
            }
            n796 = Wait (ms)(milliseconds to wait="NI DMM 1 Resistance Wait") -> ()  [unwired: 1 out]
            n797 = call <vilib>:"Simple Error Handler.vi"("error in (no error)"=w1257) -> ("error out"=w1256:errorcluster)  [unwired: 1 in, 7 out]
          }
        }
      }
      n798 = call <instrlib>:"niDMM Close.vi"("error in (no error)"=w1197, "instrument handle"=w1199) -> ("error out"=w1196:errorcluster)  [unwired: 9 in]
      n799 = local write "NI DMM 1 error out"(w1196) -> ()
      n800 = Close File(refnum=w1200) -> ()  [unwired: 1 in, 2 out]
      n801 = call <vilib>:"Simple Error Handler.vi"("error in (no error)"=w1196) -> ()  [unwired: 1 in, 8 out]
    }
  }
  n802 = case shown="True" w18 {
    tunnel: w24 -> [_ w1302]
    tunnel: w3 -> [_ _]
    tunnel: w21 -> [_ w1299]
    frame False {
    }
    frame True {
      n803 = local read "NI DMM 2 Option Return"() -> (w1296:enum32{"Ampermeter button", "Ohmmeter button"})
      n804 = case shown="\"Ohmmeter button\"" w1296 {
        tunnel: w1302 -> [w1307 w1354]
        tunnel: [w1306 w1352] -> w1301
        tunnel: [w1305 w1351] -> w1300
        tunnel: w1299 -> [w1304 w1353]
        tunnel: [w1303 w1350] -> w1298
        frame "Ampermeter button", Default {
          n805 = while {
            tunnel: w1307 -> [w1319]
            tunnel: [w1317] -> w1306
            tunnel: [w1316] -> w1305
            tunnel: w1304 -> [w1314]
            tunnel: [w1310] -> w1303
            stop <- w1315 stop-if-true
            n806 = flat-sequence {
              tunnel: [w1323] -> w1320
              tunnel: w1319 -> [w1321]
              tunnel: w1314 -> [w1327]
              tunnel: [w1322] -> w1313
              tunnel: w1320 -> [w1330]
              tunnel: [w1335] -> w1318
              tunnel: w1313 -> [w1334]
              tunnel: [w1333] -> w1312
              tunnel: [w1329] -> w1308
              tunnel: w1318 -> [w1340]
              tunnel: [w1341] -> w1317
              tunnel: [w1340] -> w1316
              tunnel: [w1339] -> w1315
              tunnel: [w1338] -> w1311
              tunnel: w1312 -> [w1338]
              tunnel: w1308 -> [w1337]
              frame #0 {
                w1324 = T7 6.5 items=["3 1/2"=3.5, "4 1/2"=4.5, "5 1/2"=5.5, "6 1/2"=6.5, "7 1/2"=7.5] ("Resolution in Digits")
                n807 = Fract/Exp String To Number(string="NI DMM 2 Current Range") -> (number=w1326:dbl)  [unwired: 3 in, 1 out]
                n808 = call-poly <instrlib>:"niDMM Config Measurement.vi"("Range"=w1326, "Resolution in Digits"=w1324, "error in (no error)"=w1327, "Function"=niDMM_Function."DC Current" ("Measurement Type"), "instrument handle"=w1321) -> ("error out"=w1322:errorcluster, "instrument handle out"=w1323:refnum<k15>)  [unwired: 5 in]
              }
              frame #1 {
                n809 = call <instrlib>:"niDMM Read.vi"("error in (no error)"=w1334, "instrument handle"=w1330) -> ("error out"=w1333:errorcluster, "Measurement"=w1329:dbl, "instrument handle out"=w1335:refnum<k15>)  [unwired: 7 in]
                "DMM 2 Real Current" <- w1329
                n810 = Fract/Exp String To Number(string="NI DMM 2 units") -> (number=w1331:dbl)  [unwired: 3 in, 1 out]
                n811 = Multiply(x=w1331, y=w1329) -> (x*y=→"NI DMM 2 Current" →"NI DMM 2 Current Char":dbl)
              }
              frame #2 {
                w1342 = 6
                n812 = local read "NI DMM 2 Current output file"() -> (w1349:refnum<file>)
                n813 = Format Date/Time String(time format string (%c)="%H:%M:%S:%3u") -> (date/time string=w1344:string)  [unwired: 2 in]
                n814 = Number To Fractional String(number=w1337, width (-)=w1342, precision (6)=w1342) -> (F-format string=w1347:string)  [unwired: 1 in]
                n815 = local read "System Stop"() -> (w1339:bool)
                n816 = Concatenate Strings(w1344, "\t", w1347, "\r\n") -> (w1346:string)
                n817 = Format Into String(initial string=w1349, w1346) -> (resulting string=w1341:refnum<file>)  [unwired: 2 in, 1 out]
              }
            }
            n818 = Wait (ms)(milliseconds to wait="NI DMM 2 Current Wait") -> ()  [unwired: 1 out]
            n819 = call <vilib>:"Simple Error Handler.vi"("error in (no error)"=w1311) -> ("error out"=w1310:errorcluster)  [unwired: 1 in, 7 out]
          }
        }
        frame "Ohmmeter button" {
          n820 = while {
            tunnel: w1354 -> [w1366]
            tunnel: [w1364] -> w1352
            tunnel: [w1363] -> w1351
            tunnel: w1353 -> [w1361]
            tunnel: [w1357] -> w1350
            stop <- w1362 stop-if-true
            n821 = flat-sequence {
              tunnel: [w1373] -> w1367
              tunnel: w1366 -> [w1372]
              tunnel: w1361 -> [w1371]
              tunnel: [w1370] -> w1360
              tunnel: w1367 -> [w1378]
              tunnel: [w1377] -> w1365
              tunnel: w1360 -> [w1382]
              tunnel: [w1381] -> w1359
              tunnel: [w1376] -> w1355
              tunnel: w1365 -> [w1388]
              tunnel: [w1389] -> w1364
              tunnel: [w1388] -> w1363
              tunnel: [w1387] -> w1362
              tunnel: [w1386] -> w1358
              tunnel: w1359 -> [w1386]
              tunnel: w1355 -> [w1385]
              frame #0 {
                w1375 = T7 6.5 items=["3 1/2"=3.5, "4 1/2"=4.5, "5 1/2"=5.5, "6 1/2"=6.5, "7 1/2"=7.5] ("Resolution in Digits")
                n822 = Fract/Exp String To Number(string="NI DMM 2 Resistance Range") -> (number=w1369:dbl)  [unwired: 3 in, 1 out]
                n823 = call-poly <instrlib>:"niDMM Config Measurement.vi"("Range"=w1369, "Resolution in Digits"=w1375, "error in (no error)"=w1371, "Function"=niDMM_Function."2-wire Resistance" ("Measurement Type"), "instrument handle"=w1372) -> ("error out"=w1370:errorcluster, "instrument handle out"=w1373:refnum<k15>)  [unwired: 5 in]
              }
              frame #1 {
                n824 = call <instrlib>:"niDMM Read.vi"("error in (no error)"=w1382, "instrument handle"=w1378) -> ("error out"=w1381:errorcluster, "Measurement"=w1376:dbl, "instrument handle out"=w1377:refnum<k15>)  [unwired: 7 in]
                n825 = Fract/Exp String To Number(string="NI DMM 2 Resistance units") -> (number=w1379:dbl)  [unwired: 3 in, 1 out]
                n826 = Multiply(x=w1379, y=w1376) -> (x*y=→"NI DMM 2 Resistance" →"NI DMM 2 Resistance Char":dbl)
              }
              frame #2 {
                w1390 = 12
                n827 = local read "NI DMM 2 Resistance output file"() -> (w1396:refnum<file>)
                n828 = Format Date/Time String(time format string (%c)="%H:%M:%S:%3u") -> (date/time string=w1392:string)  [unwired: 2 in]
                n829 = Number To Fractional String(number=w1385, width (-)=w1390, precision (6)=w1390) -> (F-format string=w1384:string)  [unwired: 1 in]
                n830 = Concatenate Strings(w1392, "\t", w1384, "\r\n") -> (w1394:string)
                n831 = Format Into String(initial string=w1396, w1394) -> (resulting string=w1389:refnum<file>)  [unwired: 2 in, 1 out]
                n832 = local read "System Stop"() -> (w1387:bool)
              }
            }
            n833 = Wait (ms)(milliseconds to wait="NI DMM 2 Resistance Wait") -> ()  [unwired: 1 out]
            n834 = call <vilib>:"Simple Error Handler.vi"("error in (no error)"=w1358) -> ("error out"=w1357:errorcluster)  [unwired: 1 in, 7 out]
          }
        }
      }
      n835 = call <instrlib>:"niDMM Close.vi"("error in (no error)"=w1298, "instrument handle"=w1300) -> ("error out"=w1297:errorcluster)  [unwired: 9 in]
      n836 = local write "NI DMM 2 error out"(w1297) -> ()
      n837 = Close File(refnum=w1301) -> ()  [unwired: 1 in, 2 out]
      n838 = call <vilib>:"Simple Error Handler.vi"("error in (no error)"=w1297) -> ()  [unwired: 1 in, 8 out]
    }
  }
  n839 = case shown="True" w2 {
    tunnel: w14 -> [_ w1403]
    tunnel: w15 -> [_ w1400]
    tunnel: w3 -> [_ _]
    frame False {
    }
    frame True {
      n840 = local read "NI DMM 3 Option Return"() -> (w1397:enum32{"Ampermeter button", "Ohmmeter button"})
      n841 = case shown="\"Ampermeter button\", Default" w1397 {
        tunnel: w1403 -> [w1408 w1455]
        tunnel: [w1407 w1453] -> w1402
        tunnel: [w1406 w1452] -> w1401
        tunnel: w1400 -> [w1405 w1454]
        tunnel: [w1404 w1451] -> w1399
        frame "Ampermeter button", Default {
          n842 = while {
            tunnel: w1408 -> [w1420]
            tunnel: [w1418] -> w1407
            tunnel: [w1417] -> w1406
            tunnel: w1405 -> [w1415]
            tunnel: [w1411] -> w1404
            stop <- w1416 stop-if-true
            n843 = flat-sequence {
              tunnel: [w1424] -> w1421
              tunnel: w1420 -> [w1422]
              tunnel: w1415 -> [w1428]
              tunnel: [w1423] -> w1414
              tunnel: w1421 -> [w1430]
              tunnel: [w1436] -> w1419
              tunnel: w1414 -> [w1435]
              tunnel: [w1434] -> w1413
              tunnel: [w1431] -> w1409
              tunnel: w1419 -> [w1442]
              tunnel: [w1443] -> w1418
              tunnel: [w1442] -> w1417
              tunnel: [w1441] -> w1416
              tunnel: [w1440] -> w1412
              tunnel: w1413 -> [w1440]
              tunnel: w1409 -> [w1439]
              frame #0 {
                w1425 = T7 6.5 items=["3 1/2"=3.5, "4 1/2"=4.5, "5 1/2"=5.5, "6 1/2"=6.5, "7 1/2"=7.5] ("Resolution in Digits")
                n844 = Fract/Exp String To Number(string="NI DMM 3 Current Range") -> (number=w1427:dbl)  [unwired: 3 in, 1 out]
                n845 = call-poly <instrlib>:"niDMM Config Measurement.vi"("Range"=w1427, "Resolution in Digits"=w1425, "error in (no error)"=w1428, "Function"=niDMM_Function."DC Current" ("Measurement Type"), "instrument handle"=w1422) -> ("error out"=w1423:errorcluster, "instrument handle out"=w1424:refnum<k15>)  [unwired: 5 in]
              }
              frame #1 {
                n846 = call <instrlib>:"niDMM Read.vi"("error in (no error)"=w1435, "instrument handle"=w1430) -> ("error out"=w1434:errorcluster, "Measurement"=w1431:dbl, "instrument handle out"=w1436:refnum<k15>)  [unwired: 7 in]
                "DMM 3 Real Current" <- w1431
                n847 = Fract/Exp String To Number(string="NI DMM 3 units") -> (number=w1432:dbl)  [unwired: 3 in, 1 out]
                n848 = Multiply(x=w1432, y=w1431) -> (x*y=→"NI DMM 3 Current" →"NI DMM 3 Current Char":dbl)
              }
              frame #2 {
                w1444 = 12
                n849 = local read "NI DMM 3 Current output file"() -> (w1450:refnum<file>)
                n850 = Format Date/Time String(time format string (%c)="%H:%M:%S:%3u") -> (date/time string=w1446:string)  [unwired: 2 in]
                n851 = Number To Fractional String(number=w1439, width (-)=w1444, precision (6)=w1444) -> (F-format string=w1438:string)  [unwired: 1 in]
                n852 = Concatenate Strings(w1446, "\t", w1438, "\r\n") -> (w1448:string)
                n853 = Format Into String(initial string=w1450, w1448) -> (resulting string=w1443:refnum<file>)  [unwired: 2 in, 1 out]
                n854 = local read "System Stop"() -> (w1441:bool)
              }
            }
            n855 = Wait (ms)(milliseconds to wait="NI DMM 3 Current Wait") -> ()  [unwired: 1 out]
            n856 = call <vilib>:"Simple Error Handler.vi"("error in (no error)"=w1412) -> ("error out"=w1411:errorcluster)  [unwired: 1 in, 7 out]
          }
        }
        frame "Ohmmeter button" {
          n857 = while {
            tunnel: w1455 -> [w1467]
            tunnel: [w1465] -> w1453
            tunnel: [w1464] -> w1452
            tunnel: w1454 -> [w1462]
            tunnel: [w1458] -> w1451
            stop <- w1463 stop-if-true
            n858 = flat-sequence {
              tunnel: [w1474] -> w1468
              tunnel: w1467 -> [w1473]
              tunnel: w1462 -> [w1472]
              tunnel: [w1471] -> w1461
              tunnel: w1468 -> [w1479]
              tunnel: [w1478] -> w1466
              tunnel: w1461 -> [w1483]
              tunnel: [w1482] -> w1460
              tunnel: [w1477] -> w1456
              tunnel: w1466 -> [w1488]
              tunnel: [w1489] -> w1465
              tunnel: [w1488] -> w1464
              tunnel: [w1487] -> w1463
              tunnel: [w1486] -> w1459
              tunnel: w1460 -> [w1486]
              tunnel: w1456 -> [w1485]
              frame #0 {
                w1476 = T7 6.5 items=["3 1/2"=3.5, "4 1/2"=4.5, "5 1/2"=5.5, "6 1/2"=6.5, "7 1/2"=7.5] ("Resolution in Digits")
                n859 = Fract/Exp String To Number(string="NI DMM 3 Resistance Range") -> (number=w1470:dbl)  [unwired: 3 in, 1 out]
                n860 = call-poly <instrlib>:"niDMM Config Measurement.vi"("Range"=w1470, "Resolution in Digits"=w1476, "error in (no error)"=w1472, "Function"=niDMM_Function."2-wire Resistance" ("Measurement Type"), "instrument handle"=w1473) -> ("error out"=w1471:errorcluster, "instrument handle out"=w1474:refnum<k15>)  [unwired: 5 in]
              }
              frame #1 {
                n861 = call <instrlib>:"niDMM Read.vi"("error in (no error)"=w1483, "instrument handle"=w1479) -> ("error out"=w1482:errorcluster, "Measurement"=w1477:dbl, "instrument handle out"=w1478:refnum<k15>)  [unwired: 7 in]
                n862 = Fract/Exp String To Number(string="NI DMM 3 Resistance units") -> (number=w1480:dbl)  [unwired: 3 in, 1 out]
                n863 = Multiply(x=w1480, y=w1477) -> (x*y=→"NI DMM 3 Resistance" →"NI DMM 3 Resistance Char":dbl)
              }
              frame #2 {
                w1490 = 6
                n864 = local read "NI DMM 3 Resistance output file"() -> (w1497:refnum<file>)
                n865 = Format Date/Time String(time format string (%c)="%H:%M:%S:%3u") -> (date/time string=w1492:string)  [unwired: 2 in]
                n866 = Number To Fractional String(number=w1485, width (-)=w1490, precision (6)=w1490) -> (F-format string=w1495:string)  [unwired: 1 in]
                n867 = local read "System Stop"() -> (w1487:bool)
                n868 = Concatenate Strings(w1492, "\t", w1495, "\r\n") -> (w1494:string)
                n869 = Format Into String(initial string=w1497, w1494) -> (resulting string=w1489:refnum<file>)  [unwired: 2 in, 1 out]
              }
            }
            n870 = Wait (ms)(milliseconds to wait="NI DMM 3 Resistance Wait") -> ()  [unwired: 1 out]
            n871 = call <vilib>:"Simple Error Handler.vi"("error in (no error)"=w1459) -> ("error out"=w1458:errorcluster)  [unwired: 1 in, 7 out]
          }
        }
      }
      n872 = call <instrlib>:"niDMM Close.vi"("error in (no error)"=w1399, "instrument handle"=w1401) -> ("error out"=w1398:errorcluster)  [unwired: 9 in]
      n873 = local write "NI DMM 3 error out"(w1398) -> ()
      n874 = Close File(refnum=w1402) -> ()  [unwired: 1 in, 2 out]
      n875 = call <vilib>:"Simple Error Handler.vi"("error in (no error)"=w1398) -> ()  [unwired: 1 in, 8 out]
    }
  }
  n876 = case shown="True" w20 {
    tunnel: w3 -> [_ w1503]
    tunnel: w26 -> [_ w1499]
    tunnel: w23 -> [_ w1498]
    frame False {
    }
    frame True {
      n877 = while {
        tunnel: w1499 -> [w1530]
        tunnel: [w1535] -> w1502
        tunnel: [w1524] -> w1501
        tunnel: [w1509] -> w1500
        tunnel: w1503 -> [_]
        tunnel: w1498 -> [w1511]
        stop <- w1531 stop-if-true
        n878 = flat-sequence {
          tunnel: w1530 -> [w1543]
          tunnel: [w1540] -> w1519
          tunnel: w1511 -> [w1537]
          tunnel: [w1536] -> w1517
          tunnel: [w1550] -> w1534
          tunnel: w1519 -> [w1549]
          tunnel: w1517 -> [w1546]
          tunnel: [w1545] -> w1516
          tunnel: [w1559] -> w1533
          tunnel: w1534 -> [w1558]
          tunnel: w1516 -> [w1557]
          tunnel: [w1556] -> w1515
          tunnel: w1533 -> [w1563]
          tunnel: [w1562] -> w1532
          tunnel: w1515 -> [w1561]
          tunnel: [w1560] -> w1514
          tunnel: [w1580] -> w1528
          tunnel: w1532 -> [w1582]
          tunnel: [w1579] -> w1526
          tunnel: [w1572] -> w1522
          tunnel: [w1574] -> w1521
          tunnel: [w1573] -> w1520
          tunnel: [w1569] -> w1518
          tunnel: w1514 -> [w1568]
          tunnel: [w1567] -> w1512
          tunnel: w1528 -> [w1644]
          tunnel: [w1644] -> w1527
          tunnel: w1526 -> [w1627]
          tunnel: [w1634] -> w1525
          tunnel: [w1632] -> w1523
          tunnel: w1522 -> [w1631]
          tunnel: w1521 -> [w1630]
          tunnel: w1520 -> [w1629]
          tunnel: w1518 -> [w1625]
          tunnel: [w1622] -> w1513
          tunnel: w1512 -> [w1622]
          tunnel: [w1650] -> w1535
          tunnel: w1527 -> [w1650]
          tunnel: [w1651] -> w1531
          tunnel: w1525 -> [w1649]
          tunnel: [w1649] -> w1524
          tunnel: w1523 -> [_]
          tunnel: w1513 -> [w1648]
          tunnel: [w1648] -> w1510
          frame #0 {
            n879 = call <instrlib>:"niScope Configure Vertical.vi"("instrument handle"=w1543, "probe attenuation"=1.0 ("Probe Attenuation"), "vertical coupling"="AC/DC/Groun", "channels"="0" ("Channel Name"), "vertical range"="vertical range", "vertical offset"=0.0, "error in"=w1537) -> ("instrument handle out"=w1540:refnum<k15>, "error out"=w1536:errorcluster)  [unwired: 7 in]
          }
          frame #1 {
            w1555 = 0 items=["Positive", "Negative"] ("Trigger Slope")
            w1554 = u16 1 items=["AC"=0, "DC"=1, "HF Reject"=3, "LF Reject"=4, "AC Plus HF Reject"=1001] ("Coupling")
            n880 = call-poly <instrlib>:"niScope Configure Trigger (poly).vi"("instrument handle"=w1549, "trigger window mode"=w1555, "trigger coupling"=w1554, "trigger source"="Trigger Source", "low level"="Low Level", "high level"="High Level", "error in"=w1546, "trigger holdoff"=0.0, "trigger delay"=0.0 ("Trigger Delay")) -> ("instrument handle out"=w1550:refnum<k15>, "error out"=w1545:errorcluster)  [unwired: 5 in]
          }
          frame #2 {
            n881 = call <instrlib>:"niScope Initiate Acquisition.vi"("instrument handle"=w1558, "error in"=w1557) -> ("instrument handle out"=w1559:refnum<k15>, "error out"=w1556:errorcluster)  [unwired: 12 in]
          }
          frame #3 {
            n882 = call-poly <instrlib>:"niScope Fetch (poly).vi"("timeout"=1.0, "error in"=w1561, "channels"="0", "instrument handle"=w1563) -> ("error out"=w1560:errorcluster, "waveform"=→"RealTime Waveform":T2, "instrument handle out"=w1562:refnum<k15>)  [unwired: 4 in, 1 out]
          }
          frame #4 {
            # "Во время триггера FALSE"
            n883 = property class="niScope" props=["Auto Triggered", "Trigger Hysteresis"](reference=w1582) -> (reference out=w1581:refnum<k15>, "Auto Triggered"=w1578:bool)  [unwired: 1 in, 2 out]
            n884 = case shown="\"Radio Selection P1 CH1\"" "Channel for SEU" {
              tunnel: [w1584 w1590 w1592 w1596] -> w1574
              tunnel: [w1585 w1589 w1593 w1597] -> w1573
              tunnel: [w1586 w1588 w1594 w1598] -> w1572
              tunnel: [w1583 w1587 w1591 w1595] -> w1570
              frame "Radio Selection P1 CH0", Default {
                n885 = local read "P1 CH0_warning"() -> (w1583:bool)
                n886 = local read "P1 CH0_cur, A"() -> (w1584:dbl)
                n887 = local read "P1 CH0, V"() -> (w1585:dbl)
                n888 = Get Date/Time In Seconds() -> (seconds since 1Jan1904=w1586:timestamp)
              }
              frame "Radio Selection P1 CH1" {
                n889 = local read "P1 CH1_warning"() -> (w1587:bool)
                n890 = local read "P1 CH1_cur, A"() -> (w1590:dbl)
                n891 = local read "P1 CH1, V"() -> (w1589:dbl)
                n892 = Get Date/Time In Seconds() -> (seconds since 1Jan1904=w1588:timestamp)
              }
              frame "Radio Selection P2 CH0" {
                n893 = local read "P2 CH0_warning"() -> (w1591:bool)
                n894 = local read "P2 CH0_cur, A"() -> (w1592:dbl)
                n895 = local read "P2 CH0, V"() -> (w1593:dbl)
                n896 = Get Date/Time In Seconds() -> (seconds since 1Jan1904=w1594:timestamp)
              }
              frame "Radio Selection P2 CH1" {
                n897 = local read "P1 CH1_warning"() -> (w1595:bool)
                n898 = local read "P2 CH1_cur, A"() -> (w1596:dbl)
                n899 = local read "P2 CH1, V"() -> (w1597:dbl)
                n900 = Get Date/Time In Seconds() -> (seconds since 1Jan1904=w1598:timestamp)
              }
            }
            n901 = Not(x=w1578) -> (.not. x?=w1577:bool)
            n902 = Not(x=w1570) -> (.not. x?=w1575:bool)
            n903 = And(x=w1575, y=w1577) -> (x .and. y?=w1576:bool)
            n904 = case shown="True" w1576 {
              tunnel: w1581 -> [w1602 w1617]
              tunnel: [w1602 w1609] -> w1580
              tunnel: [FALSE TRUE] -> w1579
              tunnel: ["" w1606] -> w1569
              tunnel: w1568 -> [w1599 w1605]
              tunnel: [w1599 w1603] -> w1567
              frame False {
              }
              frame True {
                w1608 = 6
                # "Регистрация SEU"
                n905 = call-poly <instrlib>:"niScope Fetch (poly).vi"("timeout"=1.0, "error in"=w1605, "channels"="0", "instrument handle"=w1617) -> ("error out"=w1604:errorcluster, "waveform"=→"SEU Waveform":T2, "instrument handle out"=w1610:refnum<k15>)  [unwired: 4 in, 1 out]
                n906 = call-poly <instrlib>:"niScope Fetch (poly).vi"("timeout"=1.0, "error in"=w1604, "numSamples"=1, "channels"="0", "instrument handle"=w1610) -> ("error out"=w1603:errorcluster, "wfm"=w1615:dbl[], "instrument handle out"=w1609:refnum<k15>)  [unwired: 3 in, 1 out]
                n907 = Index Array(array=w1615, index=0) -> (element=w1607:dbl)
                "SEU Last Level" <- w1607
                n908 = Number To Fractional String(number=w1607, width (-)=w1608, precision (6)=w1608) -> (F-format string=w1606:string)  [unwired: 1 in]
              }
            }
          }
          frame #5 {
            w1635 = 6
            w1639 = 0
            w1638 = 6
            w1626 = "\t"
            # "Регистрация SEU"
            n909 = case shown="True" w1627 {
              tunnel: [w1645 w1646] -> w1628
              frame False {
                n910 = local read "SEU_Counter"() -> (w1645:u32)
              }
              frame True {
                n911 = local read "SEU_Counter"() -> (w1647:u32)
                n912 = Increment(x=w1647) -> (x+1=w1646:u32)
                "SEU_Counter" <- w1646
              }
            }
            n913 = Format Date/Time String(time format string (%c)="%H:%M:%S:%3u", seconds (now)=w1631) -> (date/time string=w1641:string)  [unwired: 1 in]
            n914 = local read "SEU output file refnum"() -> (w1621:refnum<file>)
            n915 = Number To Fractional String(number=w1629, width (-)=w1635, precision (6)=w1635) -> (F-format string=w1640:string)  [unwired: 1 in]
            n916 = Number To Fractional String(number=w1630, width (-)=w1638, precision (6)=w1638) -> (F-format string=w1642:string)  [unwired: 1 in]
            n917 = Number To Fractional String(number=w1628, width (-)=w1639, precision (6)=w1639) -> (F-format string=w1643:string)  [unwired: 1 in]
            n918 = Select(t="???", s=w1627, f="") -> (s? t:f=w1624:string)
            n919 = Concatenate Strings(w1641, w1626, w1640, w1626, w1642, w1626, w1643, w1626, w1625, w1626, w1624, "\r\n") -> (w1632:string)
            n920 = Format Into String(initial string=w1621, w1632) -> (resulting string=w1634:refnum<file>)  [unwired: 2 in, 1 out]
            "SEU_warning" <- w1627
            "SEU" <- w1627
          }
          frame #6 {
            n921 = local read "System Stop"() -> (w1651:bool)
          }
        }
        n922 = Wait (ms)(milliseconds to wait=u32 1) -> ()  [unwired: 1 out]
        n923 = call <vilib>:"Simple Error Handler.vi"("error in (no error)"=w1510) -> ("error out"=w1509:errorcluster)  [unwired: 1 in, 7 out]
        "NI Scope error out" <- w1509
      }
      n924 = flat-sequence {
        tunnel: w1502 -> [w1508]
        tunnel: w1501 -> [w1507]
        tunnel: w1500 -> [w1506]
        frame #0 {
          n925 = Close File(refnum=w1507) -> ()  [unwired: 1 in, 2 out]
          n926 = call <instrlib>:"niScope Close.vi"("instrument handle"=w1508, "error in"=w1506) -> ("error out"=w1505:errorcluster)  [unwired: 13 in]
          n927 = call <vilib>:"Simple Error Handler.vi"("error in (no error)"=w1505) -> ("error out"=w1504:errorcluster)  [unwired: 1 in, 7 out]
          n928 = local write "NI Scope error out"(w1504) -> ()
        }
      }
    }
  }
  n929 = while {
    tunnel: w33 -> [w1663]
    tunnel: [w1662] -> _
    tunnel: w32 -> [w1660]
    tunnel: [w1659] -> w35
    tunnel: [w1658] -> w34
    tunnel: [w1654] -> w30
    tunnel: [w1652] -> w29
    tunnel: w28 -> [w1657]
    tunnel: w27 -> [w1656]
    tunnel: w1 -> [_]
    stop <- w1662 stop-if-true
    # "Инициализация источников"
    n930 = Wait (ms)(milliseconds to wait=u32 1) -> ()  [unwired: 1 out]
    n931 = flat-sequence {
      tunnel: w1663 -> [w1665]
      tunnel: [w1748] -> w1662
      tunnel: w1660 -> [w1664]
      tunnel: [w1707] -> w1659
      tunnel: [w1706] -> w1658
      tunnel: [w1705] -> w1655
      tunnel: [w1704] -> w1653
      tunnel: w1657 -> [w1703]
      tunnel: w1656 -> [w1700]
      frame #0 {
        w1666 = T8 0 items=["Current", "Voltage"] ("measurement type")
        n932 = local read "Power OFF"() -> (w1725:bool)
        n933 = call <instrlib>:"niDCPower Configure Current Limit.vi"("error in (no error)"=w1703, "current limit"="P1 CH0_curlim, A", "channel name"="0", "instrument handle"=w1665) -> ("error out"=w1702:errorcluster, "instrument handle out"=w1762:refnum<k15>)  [unwired: 6 in]
        n934 = call <instrlib>:"niDCPower Configure Current Limit.vi"("current limit"="P1 CH1_curlim, A", "channel name"="1", "instrument handle"=w1665) -> ("instrument handle out"=w1759:refnum<k15>)  [unwired: 7 in, 1 out]
        n935 = call <instrlib>:"niDCPower Configure Current Limit.vi"("error in (no error)"=w1700, "current limit"="P2 CH0_curlim, A", "channel name"="0", "instrument handle"=w1664) -> ("error out"=w1701:errorcluster, "instrument handle out"=w1738:refnum<k15>)  [unwired: 6 in]
        n936 = call <instrlib>:"niDCPower Configure Current Limit.vi"("current limit"="P2 CH1_curlim, A", "channel name"="1", "instrument handle"=w1664) -> ("instrument handle out"=w1717:refnum<k15>)  [unwired: 7 in, 1 out]
        n937 = call <instrlib>:"niDCPower Configure Current Limit.vi"("current limit"="P1 CH2_curlim, A", "channel name"="2", "instrument handle"=w1665) -> ("error out"=w1699:errorcluster, "instrument handle out"=w1672:refnum<k15>)  [unwired: 7 in]
        n938 = call <instrlib>:"niDCPower Configure Current Limit.vi"("current limit"="P2 CH2_curlim, A", "channel name"="2", "instrument handle"=w1664) -> ("instrument handle out"=w1689:refnum<k15>)  [unwired: 7 in, 1 out]
        n939 = local read "Power OFF"() -> (w1747:bool)
        n940 = local read "Power OFF"() -> (w1710:bool)
        n941 = local read "Power OFF"() -> (w1696:bool)
        n942 = local read "Power OFF"() -> (w1730:bool)
        n943 = local read "Power OFF"() -> (w1680:bool)
        n944 = call <instrlib>:"niDCPower Configure Voltage Level.vi"("error in (no error)"=w1702, "voltage level"="P1 CH0, V", "channel name"="0", "instrument handle"=w1762) -> ("error out"=w1767:errorcluster, "instrument handle out"=w1768:refnum<k15>)  [unwired: 6 in]
        n945 = call <instrlib>:"niDCPower Configure Voltage Level.vi"("voltage level"="P1 CH1, V", "channel name"="1", "instrument handle"=w1759) -> ("error out"=w1765:errorcluster, "instrument handle out"=w1766:refnum<k15>)  [unwired: 7 in]
        n946 = call <instrlib>:"niDCPower Configure Voltage Level.vi"("error in (no error)"=w1701, "voltage level"="P2 CH0, V", "channel name"="0", "instrument handle"=w1738) -> ("error out"=w1735:errorcluster, "instrument handle out"=w1734:refnum<k15>)  [unwired: 6 in]
        n947 = call <instrlib>:"niDCPower Configure Voltage Level.vi"("voltage level"="P2 CH1, V", "channel name"="1", "instrument handle"=w1717) -> ("error out"=w1720:errorcluster, "instrument handle out"=w1721:refnum<k15>)  [unwired: 7 in]
        n948 = call <instrlib>:"niDCPower Configure Voltage Level.vi"("error in (no error)"=w1699, "voltage level"="P1 CH2, V", "channel name"="2", "instrument handle"=w1672) -> ("error out"=w1675:errorcluster, "instrument handle out"=w1676:refnum<k15>)  [unwired: 6 in]
        n949 = call <instrlib>:"niDCPower Configure Voltage Level.vi"("voltage level"="P2 CH2, V", "channel name"="2", "instrument handle"=w1689) -> ("error out"=w1686:errorcluster, "instrument handle out"=w1685:refnum<k15>)  [unwired: 7 in]
        n950 = Select(t=FALSE, s=w1725, f="P1 CH0") -> (s? t:f=w1724:bool)
        n951 = Select(t=FALSE, s=w1747, f="P1 CH1") -> (s? t:f=w1744:bool)
        n952 = Select(t=FALSE, s=w1710, f="P2 CH1") -> (s? t:f=w1708:bool)
        n953 = Select(t=FALSE, s=w1696, f="P2 CH2") -> (s? t:f=w1698:bool)
        n954 = Select(t=FALSE, s=w1730, f="P2 CH0") -> (s? t:f=w1729:bool)
        n955 = Select(t=FALSE, s=w1680, f="P1 CH2") -> (s? t:f=w1681:bool)
        n956 = call <instrlib>:"niDCPower Configure Output Enabled.vi"("error in (no error)"=w1767, "output enabled"=w1724, "channel name"="0", "instrument handle"=w1768) -> ("error out"=w1770:errorcluster, "instrument handle out"=w1769:refnum<k15>)  [unwired: 6 in]
        n957 = call <instrlib>:"niDCPower Configure Output Enabled.vi"("error in (no error)"=w1765, "output enabled"=w1744, "channel name"="1", "instrument handle"=w1766) -> ("error out"=w1772:errorcluster, "instrument handle out"=w1771:refnum<k15>)  [unwired: 6 in]
        n958 = call <instrlib>:"niDCPower Configure Output Enabled.vi"("error in (no error)"=w1735, "output enabled"=w1729, "channel name"="0", "instrument handle"=w1734) -> ("error out"=w1732:errorcluster, "instrument handle out"=w1733:refnum<k15>)  [unwired: 6 in]
        n959 = call <instrlib>:"niDCPower Configure Output Enabled.vi"("error in (no error)"=w1720, "output enabled"=w1708, "channel name"="1", "instrument handle"=w1721) -> ("error out"=w1723:errorcluster, "instrument handle out"=w1722:refnum<k15>)  [unwired: 6 in]
        n960 = call <instrlib>:"niDCPower Configure Output Enabled.vi"("error in (no error)"=w1675, "output enabled"=w1681, "channel name"="2", "instrument handle"=w1676) -> ("error out"=w1678:errorcluster, "instrument handle out"=w1677:refnum<k15>)  [unwired: 6 in]
        n961 = call <instrlib>:"niDCPower Configure Output Enabled.vi"("error in (no error)"=w1686, "output enabled"=w1698, "channel name"="2", "instrument handle"=w1685) -> ("error out"=w1683:errorcluster, "instrument handle out"=w1684:refnum<k15>)  [unwired: 6 in]
        n962 = call <instrlib>:"niDCPower Measure.vi"("error in (no error)"=w1770, "measurement type"=w1666, "channel name"="0", "instrument handle"=w1769) -> ("error out"=w1705:errorcluster, "measurement"=→"P1 CH0_cur, A" →"P1 CH0_char":dbl, "instrument handle out"=w1707:refnum<k15>)  [unwired: 5 in]
        n963 = call <instrlib>:"niDCPower Measure.vi"("error in (no error)"=w1772, "measurement type"=w1666, "channel name"="1", "instrument handle"=w1771) -> ("measurement"=→"P1 CH1_cur, A" →"P1 CH1_char":dbl)  [unwired: 5 in, 2 out]
        n964 = call <instrlib>:"niDCPower Measure.vi"("error in (no error)"=w1732, "measurement type"=w1666, "channel name"="0", "instrument handle"=w1733) -> ("error out"=w1704:errorcluster, "measurement"=→"P2 CH0_cur, A" →"P2 CH0_char":dbl, "instrument handle out"=w1706:refnum<k15>)  [unwired: 5 in]
        n965 = call <instrlib>:"niDCPower Measure.vi"("error in (no error)"=w1723, "measurement type"=w1666, "channel name"="1", "instrument handle"=w1722) -> ("measurement"=→"P2 CH1_cur, A" →"P2 CH1_char":dbl)  [unwired: 5 in, 2 out]
        n966 = call <instrlib>:"niDCPower Measure.vi"("error in (no error)"=w1678, "measurement type"=w1666, "channel name"="2", "instrument handle"=w1677) -> ("measurement"=→"P1 CH2_cur, A" →"P1 CH2_char":dbl)  [unwired: 5 in, 2 out]
        n967 = call <instrlib>:"niDCPower Measure.vi"("error in (no error)"=w1683, "measurement type"=w1666, "channel name"="2", "instrument handle"=w1684) -> ("measurement"=→"P2 CH2_cur, A" →"P2 CH2_char":dbl)  [unwired: 5 in, 2 out]
        n968 = local read "Power OFF"() -> (w1748:bool)
      }
    }
    n969 = call <vilib>:"Simple Error Handler.vi"("error in (no error)"=w1653) -> ("error out"=w1652:errorcluster)  [unwired: 1 in, 7 out]
    "DC Power 2 error out" <- w1652
    n970 = call <vilib>:"Simple Error Handler.vi"("error in (no error)"=w1655) -> ("error out"=w1654:errorcluster)  [unwired: 1 in, 7 out]
    "DC Power 1 error out" <- w1654
  }
  n971 = while {
    tunnel: w3 -> [_]
    stop <- w1792 stop-if-true
    n972 = Wait (ms)(milliseconds to wait=u32 100) -> ()  [unwired: 1 out]
    n973 = local read "System Stop"() -> (w1785:bool)
    n974 = local read "System Stop"() -> (w1782:bool)
    n975 = Or(x="P2 CH0 Used", y=w1785) -> (x .or. y?=w1787:bool)
    n976 = Or(x="P1 CH0 Used", y=w1782) -> (x .or. y?=w1784:bool)
    n977 = case shown="True" w1784 {
      frame False {
        w1799 = T5."Disabled and Grayed Out" ("Disabled")
        n978 = property on="P1 CH0" class="Bool (strict)"("DisabledEnum"=w1799) -> ()  [unwired: 2 in, 2 out]
        n979 = property on="P1 CH0_char" class="WFChart (strict)"("DisabledEnum"=w1799) -> ()  [unwired: 2 in, 2 out]
        n980 = property on="P1 CH0, V" class="DigNum (strict)"("DisabledEnum"=w1799) -> ()  [unwired: 2 in, 2 out]
        n981 = property on="P1 CH0_curlim, A" class="DigNum (strict)"("DisabledEnum"=w1799) -> ()  [unwired: 2 in, 2 out]
        n982 = property on="P1 CH0_cur, A" class="DigNum (strict)"("DisabledEnum"=w1799) -> ()  [unwired: 2 in, 2 out]
        n983 = property on="P1 CH0_selcur, A" class="DigNum (strict)"("DisabledEnum"=w1799) -> ()  [unwired: 2 in, 2 out]
        n984 = property on="P1 CH0_counter" class="DigNum (strict)"("DisabledEnum"=w1799) -> ()  [unwired: 2 in, 2 out]
        n985 = property on="P1 CH0_warning" class="Bool (strict)"("DisabledEnum"=w1799) -> ()  [unwired: 2 in, 2 out]
      }
      frame True {
        w1800 = T5."Enabled" ("Disabled")
        n986 = property on="P1 CH0" class="Bool (strict)"("DisabledEnum"=w1800) -> ()  [unwired: 2 in, 2 out]
        n987 = property on="P1 CH0_char" class="WFChart (strict)"("DisabledEnum"=w1800) -> ()  [unwired: 2 in, 2 out]
        n988 = property on="P1 CH0, V" class="DigNum (strict)"("DisabledEnum"=w1800) -> ()  [unwired: 2 in, 2 out]
        n989 = property on="P1 CH0_curlim, A" class="DigNum (strict)"("DisabledEnum"=w1800) -> ()  [unwired: 2 in, 2 out]
        n990 = property on="P1 CH0_cur, A" class="DigNum (strict)"("DisabledEnum"=w1800) -> ()  [unwired: 2 in, 2 out]
        n991 = property on="P1 CH0_selcur, A" class="DigNum (strict)"("DisabledEnum"=w1800) -> ()  [unwired: 2 in, 2 out]
        n992 = property on="P1 CH0_counter" class="DigNum (strict)"("DisabledEnum"=w1800) -> ()  [unwired: 2 in, 2 out]
        n993 = property on="P1 CH0_warning" class="Bool (strict)"("DisabledEnum"=w1800) -> ()  [unwired: 2 in, 2 out]
      }
    }
    n994 = case shown="True" w1787 {
      frame False {
        w1801 = T5."Disabled and Grayed Out" ("Disabled")
        n995 = property on="P2 CH0" class="Bool (strict)"("DisabledEnum"=w1801) -> ()  [unwired: 2 in, 2 out]
        n996 = property on="P2 CH0_char" class="WFChart (strict)"("DisabledEnum"=w1801) -> ()  [unwired: 2 in, 2 out]
        n997 = property on="P2 CH0, V" class="DigNum (strict)"("DisabledEnum"=w1801) -> ()  [unwired: 2 in, 2 out]
        n998 = property on="P2 CH0_curlim, A" class="DigNum (strict)"("DisabledEnum"=w1801) -> ()  [unwired: 2 in, 2 out]
        n999 = property on="P2 CH0_cur, A" class="DigNum (strict)"("DisabledEnum"=w1801) -> ()  [unwired: 2 in, 2 out]
        n1000 = property on="P2 CH0_selcur, A" class="DigNum (strict)"("DisabledEnum"=w1801) -> ()  [unwired: 2 in, 2 out]
        n1001 = property on="P2 CH0_counter" class="DigNum (strict)"("DisabledEnum"=w1801) -> ()  [unwired: 2 in, 2 out]
        n1002 = property on="P2 CH0_warning" class="Bool (strict)"("DisabledEnum"=w1801) -> ()  [unwired: 2 in, 2 out]
      }
      frame True {
        w1802 = T5."Enabled" ("Disabled")
        n1003 = property on="P2 CH0" class="Bool (strict)"("DisabledEnum"=w1802) -> ()  [unwired: 2 in, 2 out]
        n1004 = property on="P2 CH0_char" class="WFChart (strict)"("DisabledEnum"=w1802) -> ()  [unwired: 2 in, 2 out]
        n1005 = property on="P2 CH0, V" class="DigNum (strict)"("DisabledEnum"=w1802) -> ()  [unwired: 2 in, 2 out]
        n1006 = property on="P2 CH0_curlim, A" class="DigNum (strict)"("DisabledEnum"=w1802) -> ()  [unwired: 2 in, 2 out]
        n1007 = property on="P2 CH0_cur, A" class="DigNum (strict)"("DisabledEnum"=w1802) -> ()  [unwired: 2 in, 2 out]
        n1008 = property on="P2 CH0_selcur, A" class="DigNum (strict)"("DisabledEnum"=w1802) -> ()  [unwired: 2 in, 2 out]
        n1009 = property on="P2 CH0_counter" class="DigNum (strict)"("DisabledEnum"=w1802) -> ()  [unwired: 2 in, 2 out]
        n1010 = property on="P2 CH0_warning" class="Bool (strict)"("DisabledEnum"=w1802) -> ()  [unwired: 2 in, 2 out]
      }
    }
    n1011 = local read "System Stop"() -> (w1788:bool)
    n1012 = local read "System Stop"() -> (w1779:bool)
    n1013 = Or(x="P2 CH1 Used", y=w1788) -> (x .or. y?=w1789:bool)
    n1014 = Or(x="P1 CH1 Used", y=w1779) -> (x .or. y?=w1781:bool)
    n1015 = case shown="True" w1789 {
      frame False {
        w1803 = T5."Disabled and Grayed Out" ("Disabled")
        n1016 = property on="P2 CH1" class="Bool (strict)"("DisabledEnum"=w1803) -> ()  [unwired: 2 in, 2 out]
        n1017 = property on="P2 CH1_char" class="WFChart (strict)"("DisabledEnum"=w1803) -> ()  [unwired: 2 in, 2 out]
        n1018 = property on="P2 CH1, V" class="DigNum (strict)"("DisabledEnum"=w1803) -> ()  [unwired: 2 in, 2 out]
        n1019 = property on="P2 CH1_curlim, A" class="DigNum (strict)"("DisabledEnum"=w1803) -> ()  [unwired: 2 in, 2 out]
        n1020 = property on="P2 CH1_cur, A" class="DigNum (strict)"("DisabledEnum"=w1803) -> ()  [unwired: 2 in, 2 out]
        n1021 = property on="P2 CH1_selcur, A" class="DigNum (strict)"("DisabledEnum"=w1803) -> ()  [unwired: 2 in, 2 out]
        n1022 = property on="P2 CH1_counter" class="DigNum (strict)"("DisabledEnum"=w1803) -> ()  [unwired: 2 in, 2 out]
        n1023 = property on="P2 CH1_warning" class="Bool (strict)"("DisabledEnum"=w1803) -> ()  [unwired: 2 in, 2 out]
      }
      frame True {
        w1804 = T5."Enabled" ("Disabled")
        n1024 = property on="P2 CH1" class="Bool (strict)"("DisabledEnum"=w1804) -> ()  [unwired: 2 in, 2 out]
        n1025 = property on="P2 CH1_char" class="WFChart (strict)"("DisabledEnum"=w1804) -> ()  [unwired: 2 in, 2 out]
        n1026 = property on="P2 CH1, V" class="DigNum (strict)"("DisabledEnum"=w1804) -> ()  [unwired: 2 in, 2 out]
        n1027 = property on="P2 CH1_curlim, A" class="DigNum (strict)"("DisabledEnum"=w1804) -> ()  [unwired: 2 in, 2 out]
        n1028 = property on="P2 CH1_cur, A" class="DigNum (strict)"("DisabledEnum"=w1804) -> ()  [unwired: 2 in, 2 out]
        n1029 = property on="P2 CH1_selcur, A" class="DigNum (strict)"("DisabledEnum"=w1804) -> ()  [unwired: 2 in, 2 out]
        n1030 = property on="P2 CH1_counter" class="DigNum (strict)"("DisabledEnum"=w1804) -> ()  [unwired: 2 in, 2 out]
        n1031 = property on="P2 CH1_warning" class="Bool (strict)"("DisabledEnum"=w1804) -> ()  [unwired: 2 in, 2 out]
      }
    }
    n1032 = case shown="True" w1781 {
      frame False {
        w1797 = T5."Disabled and Grayed Out" ("Disabled")
        n1033 = property on="P1 CH1" class="Bool (strict)"("DisabledEnum"=w1797) -> ()  [unwired: 2 in, 2 out]
        n1034 = property on="P1 CH1_char" class="WFChart (strict)"("DisabledEnum"=w1797) -> ()  [unwired: 2 in, 2 out]
        n1035 = property on="P1 CH1, V" class="DigNum (strict)"("DisabledEnum"=w1797) -> ()  [unwired: 2 in, 2 out]
        n1036 = property on="P1 CH1_curlim, A" class="DigNum (strict)"("DisabledEnum"=w1797) -> ()  [unwired: 2 in, 2 out]
        n1037 = property on="P1 CH1_cur, A" class="DigNum (strict)"("DisabledEnum"=w1797) -> ()  [unwired: 2 in, 2 out]
        n1038 = property on="P1 CH1_selcur, A" class="DigNum (strict)"("DisabledEnum"=w1797) -> ()  [unwired: 2 in, 2 out]
        n1039 = property on="P1 CH1_counter" class="DigNum (strict)"("DisabledEnum"=w1797) -> ()  [unwired: 2 in, 2 out]
        n1040 = property on="P1 CH1_warning" class="Bool (strict)"("DisabledEnum"=w1797) -> ()  [unwired: 2 in, 2 out]
      }
      frame True {
        w1798 = T5."Enabled" ("Disabled")
        n1041 = property on="P1 CH1" class="Bool (strict)"("DisabledEnum"=w1798) -> ()  [unwired: 2 in, 2 out]
        n1042 = property on="P1 CH1_char" class="WFChart (strict)"("DisabledEnum"=w1798) -> ()  [unwired: 2 in, 2 out]
        n1043 = property on="P1 CH1, V" class="DigNum (strict)"("DisabledEnum"=w1798) -> ()  [unwired: 2 in, 2 out]
        n1044 = property on="P1 CH1_curlim, A" class="DigNum (strict)"("DisabledEnum"=w1798) -> ()  [unwired: 2 in, 2 out]
        n1045 = property on="P1 CH1_cur, A" class="DigNum (strict)"("DisabledEnum"=w1798) -> ()  [unwired: 2 in, 2 out]
        n1046 = property on="P1 CH1_selcur, A" class="DigNum (strict)"("DisabledEnum"=w1798) -> ()  [unwired: 2 in, 2 out]
        n1047 = property on="P1 CH1_counter" class="DigNum (strict)"("DisabledEnum"=w1798) -> ()  [unwired: 2 in, 2 out]
        n1048 = property on="P1 CH1_warning" class="Bool (strict)"("DisabledEnum"=w1798) -> ()  [unwired: 2 in, 2 out]
      }
    }
    n1049 = local read "System Stop"() -> (w1775:bool)
    n1050 = local read "System Stop"() -> (w1778:bool)
    n1051 = Or(x="P1 CH2 Used", y=w1778) -> (x .or. y?=w1776:bool)
    n1052 = Or(x="P2 CH2 Used", y=w1775) -> (x .or. y?=w1774:bool)
    n1053 = case shown="True" w1776 {
      frame False {
        w1795 = T5."Disabled and Grayed Out" ("Disabled")
        n1054 = property on="P1 CH2" class="Bool (strict)"("DisabledEnum"=w1795) -> ()  [unwired: 2 in, 2 out]
        n1055 = property on="P1 CH2_char" class="WFChart (strict)"("DisabledEnum"=w1795) -> ()  [unwired: 2 in, 2 out]
        n1056 = property on="P1 CH2, V" class="DigNum (strict)"("DisabledEnum"=w1795) -> ()  [unwired: 2 in, 2 out]
        n1057 = property on="P1 CH2_curlim, A" class="DigNum (strict)"("DisabledEnum"=w1795) -> ()  [unwired: 2 in, 2 out]
        n1058 = property on="P1 CH2_cur, A" class="DigNum (strict)"("DisabledEnum"=w1795) -> ()  [unwired: 2 in, 2 out]
        n1059 = property on="P1 CH2_selcur, A" class="DigNum (strict)"("DisabledEnum"=w1795) -> ()  [unwired: 2 in, 2 out]
        n1060 = property on="P1 CH2_counter" class="DigNum (strict)"("DisabledEnum"=w1795) -> ()  [unwired: 2 in, 2 out]
        n1061 = property on="P1 CH2_warning" class="Bool (strict)"("DisabledEnum"=w1795) -> ()  [unwired: 2 in, 2 out]
      }
      frame True {
        w1796 = T5."Enabled" ("Disabled")
        n1062 = property on="P1 CH2_char" class="WFChart (strict)"("DisabledEnum"=w1796) -> ()  [unwired: 2 in, 2 out]
        n1063 = property on="P1 CH2, V" class="DigNum (strict)"("DisabledEnum"=w1796) -> ()  [unwired: 2 in, 2 out]
        n1064 = property on="P1 CH2_curlim, A" class="DigNum (strict)"("DisabledEnum"=w1796) -> ()  [unwired: 2 in, 2 out]
        n1065 = property on="P1 CH2_cur, A" class="DigNum (strict)"("DisabledEnum"=w1796) -> ()  [unwired: 2 in, 2 out]
        n1066 = property on="P1 CH2_selcur, A" class="DigNum (strict)"("DisabledEnum"=w1796) -> ()  [unwired: 2 in, 2 out]
        n1067 = property on="P1 CH2_counter" class="DigNum (strict)"("DisabledEnum"=w1796) -> ()  [unwired: 2 in, 2 out]
        n1068 = property on="P1 CH2_warning" class="Bool (strict)"("DisabledEnum"=w1796) -> ()  [unwired: 2 in, 2 out]
        n1069 = property on="P1 CH2" class="Bool (strict)"("DisabledEnum"=w1796) -> ()  [unwired: 2 in, 2 out]
      }
    }
    n1070 = case shown="True" w1774 {
      frame False {
        w1793 = T5."Disabled and Grayed Out" ("Disabled")
        n1071 = property on="P2 CH2" class="Bool (strict)"("DisabledEnum"=w1793) -> ()  [unwired: 2 in, 2 out]
        n1072 = property on="P2 CH2_char" class="WFChart (strict)"("DisabledEnum"=w1793) -> ()  [unwired: 2 in, 2 out]
        n1073 = property on="P2 CH2, V" class="DigNum (strict)"("DisabledEnum"=w1793) -> ()  [unwired: 2 in, 2 out]
        n1074 = property on="P2 CH2_curlim, A" class="DigNum (strict)"("DisabledEnum"=w1793) -> ()  [unwired: 2 in, 2 out]
        n1075 = property on="P2 CH2_cur, A" class="DigNum (strict)"("DisabledEnum"=w1793) -> ()  [unwired: 2 in, 2 out]
        n1076 = property on="P2 CH2_selcur, A" class="DigNum (strict)"("DisabledEnum"=w1793) -> ()  [unwired: 2 in, 2 out]
        n1077 = property on="P2 CH2_counter" class="DigNum (strict)"("DisabledEnum"=w1793) -> ()  [unwired: 2 in, 2 out]
        n1078 = property on="P2 CH2_warning" class="Bool (strict)"("DisabledEnum"=w1793) -> ()  [unwired: 2 in, 2 out]
      }
      frame True {
        w1794 = T5."Enabled" ("Disabled")
        n1079 = property on="P2 CH2" class="Bool (strict)"("DisabledEnum"=w1794) -> ()  [unwired: 2 in, 2 out]
        n1080 = property on="P2 CH2_char" class="WFChart (strict)"("DisabledEnum"=w1794) -> ()  [unwired: 2 in, 2 out]
        n1081 = property on="P2 CH2, V" class="DigNum (strict)"("DisabledEnum"=w1794) -> ()  [unwired: 2 in, 2 out]
        n1082 = property on="P2 CH2_curlim, A" class="DigNum (strict)"("DisabledEnum"=w1794) -> ()  [unwired: 2 in, 2 out]
        n1083 = property on="P2 CH2_cur, A" class="DigNum (strict)"("DisabledEnum"=w1794) -> ()  [unwired: 2 in, 2 out]
        n1084 = property on="P2 CH2_selcur, A" class="DigNum (strict)"("DisabledEnum"=w1794) -> ()  [unwired: 2 in, 2 out]
        n1085 = property on="P2 CH2_counter" class="DigNum (strict)"("DisabledEnum"=w1794) -> ()  [unwired: 2 in, 2 out]
        n1086 = property on="P2 CH2_warning" class="Bool (strict)"("DisabledEnum"=w1794) -> ()  [unwired: 2 in, 2 out]
      }
    }
    n1087 = local read "System Stop"() -> (w1792:bool)
  }
  n1088 = while {
    shift-right: [w1824] -> _
    shift-left: FALSE -> [w1830]
    shift-right: [w1823] -> _
    shift-left: FALSE -> [w1829]
    shift-right: [w1825] -> _
    shift-left: FALSE -> [w1828]
    shift-right: [w1826] -> _
    shift-left: FALSE -> [w1827]
    shift-right: [w1819] -> _
    shift-left: FALSE -> [w1820]
    shift-right: [w1817] -> _
    shift-left: FALSE -> [w1818]
    shift-right: [w1815] -> _
    shift-left: FALSE -> [w1816]
    shift-right: [w1813] -> _
    shift-left: FALSE -> [w1814]
    tunnel: w3 -> [_]
    shift-right: [w1810] -> _
    shift-left: FALSE -> [w1809]
    shift-right: [w1812] -> _
    shift-left: FALSE -> [w1811]
    shift-right: [w1807] -> _
    shift-left: FALSE -> [w1808]
    shift-right: [w1805] -> _
    shift-left: FALSE -> [w1806]
    stop <- w1821 stop-if-true
    # "Включение / выключение каналов"
    n1089 = stacked-sequence {
      tunnel: w1830 -> [w1896 _]
      tunnel: [w1892 _] -> w1824
      tunnel: w1829 -> [w1888 _]
      tunnel: [w1887 _] -> w1823
      tunnel: w1828 -> [w1886 _]
      tunnel: w1827 -> [w1880 _]
      tunnel: [w1878 _] -> w1826
      tunnel: [w1877 _] -> w1825
      tunnel: [_ w1921] -> w1821
      tunnel: w1820 -> [w1874 _]
      tunnel: [w1871 _] -> w1819
      tunnel: w1818 -> [w1870 _]
      tunnel: [w1865 _] -> w1817
      tunnel: w1816 -> [w1860 _]
      tunnel: [w1859 _] -> w1815
      tunnel: w1814 -> [w1854 _]
      tunnel: [w1855 _] -> w1813
      tunnel: w1809 -> [w1843 _]
      tunnel: [w1847 _] -> w1810
      tunnel: w1811 -> [w1851 _]
      tunnel: [w1850 _] -> w1812
      tunnel: w1808 -> [w1842 _]
      tunnel: [w1838 _] -> w1807
      tunnel: w1806 -> [w1834 _]
      tunnel: [w1835 _] -> w1805
      frame #0 {
        n1090 = local read "P1 CH0 Used"() -> (w1871:bool)
        n1091 = local read "P1 CH1 Used"() -> (w1865:bool)
        n1092 = local read "P1 CH2 Used"() -> (w1835:bool)
        n1093 = local read "P2 CH0 Used"() -> (w1859:bool)
        n1094 = local read "P2 CH1 Used"() -> (w1855:bool)
        n1095 = local read "P2 CH2 Used"() -> (w1850:bool)
        n1096 = local read "P1 CH1"() -> (w1877:bool)
        n1097 = local read "P1 CH2"() -> (w1838:bool)
        n1098 = local read "P2 CH1"() -> (w1892:bool)
        n1099 = local read "P2 CH2"() -> (w1847:bool)
        n1100 = local read "P2 CH0"() -> (w1887:bool)
        n1101 = local read "P1 CH0"() -> (w1878:bool)
        n1102 = local read "System Stop"() -> (w1867:bool)
        n1103 = local read "System Stop"() -> (w1832:bool)
        n1104 = local read "System Stop"() -> (w1831:bool)
        n1105 = local read "System Stop"() -> (w1862:bool)
        n1106 = local read "System Stop"() -> (w1875:bool)
        n1107 = Less?(x=w1877, y=w1886) -> (x < y?=w1868:bool)
        n1108 = Less?(x=w1838, y=w1842) -> (x < y?=w1837:bool)
        n1109 = Less?(x=w1892, y=w1896) -> (x < y?=w1858:bool)
        n1110 = Less?(x=w1847, y=w1843) -> (x < y?=w1848:bool)
        n1111 = Less?(x=w1887, y=w1888) -> (x < y?=w1864:bool)
        n1112 = Less?(x=w1859, y=w1860) -> (x < y?=w1861:bool)
        n1113 = Less?(x=w1878, y=w1880) -> (x < y?=w1876:bool)
        n1114 = Not(x=w1867) -> (.not. x?=w1885:bool)
        n1115 = Greater?(x=w1877, y=w1886) -> (0:w1884:bool)
        n1116 = Not(x=w1832) -> (.not. x?=w1840:bool)
        n1117 = Not(x="System Stop") -> (.not. x?=w1894:bool)
        n1118 = Not(x=w1831) -> (.not. x?=w1845:bool)
        n1119 = Not(x=w1862) -> (.not. x?=w1890:bool)
        n1120 = Greater?(x=w1838, y=w1842) -> (0:w1839:bool)
        n1121 = Greater?(x=w1892, y=w1896) -> (0:w1893:bool)
        n1122 = Greater?(x=w1847, y=w1843) -> (0:w1846:bool)
        n1123 = Not(x=w1875) -> (.not. x?=w1881:bool)
        n1124 = Greater?(x=w1887, y=w1888) -> (0:w1891:bool)
        n1125 = Greater?(x=w1878, y=w1880) -> (0:w1882:bool)
        n1126 = Less?(x=w1835, y=w1834) -> (x < y?=w1833:bool)
        n1127 = Less?(x=w1855, y=w1854) -> (x < y?=w1853:bool)
        n1128 = Less?(x=w1850, y=w1851) -> (x < y?=w1852:bool)
        n1129 = Less?(x=w1871, y=w1874) -> (x < y?=w1873:bool)
        n1130 = Less?(x=w1865, y=w1870) -> (x < y?=w1866:bool)
        n1131 = And(x=w1885, y=w1884) -> (x .and. y?=w1883:bool)
        n1132 = And(x=w1840, y=w1839) -> (x .and. y?=w1841:bool)
        n1133 = Compound Arithmetic op=OR(w1864, w1862, w1861) -> (w1863:bool)
        n1134 = And(x=w1894, y=w1893) -> (x .and. y?=w1895:bool)
        n1135 = And(x=w1845, y=w1846) -> (x .and. y?=w1844:bool)
        n1136 = And(x=w1890, y=w1891) -> (x .and. y?=w1889:bool)
        n1137 = Compound Arithmetic op=OR(w1837, w1832, w1833) -> (w1836:bool)
        n1138 = Compound Arithmetic op=OR(w1858, "System Stop", w1853) -> (w1856:bool)
        n1139 = Compound Arithmetic op=OR(w1848, w1831, w1852) -> (w1849:bool)
        n1140 = And(x=w1881, y=w1882) -> (x .and. y?=w1879:bool)
        n1141 = Compound Arithmetic op=OR(w1876, w1875, w1873) -> (w1872:bool)
        n1142 = Compound Arithmetic op=OR(w1868, w1867, w1866) -> (w1869:bool)
        n1143 = stacked-sequence {
          tunnel: w1879 -> [w1910]
          tunnel: w1872 -> [w1909]
          frame #0 {
            n1144 = case shown="True" w1910 {
              frame False {
              }
              frame True {
                # "ON"
                n1145 = local write "P1 CH0"(TRUE ("P1 CH0")) -> ()
              }
            }
            n1146 = case shown="True" w1909 {
              frame False {
              }
              frame True {
                # "OFF"
                n1147 = local write "P1 CH0"(FALSE ("P1 CH0")) -> ()
              }
            }
          }
        }
        n1148 = stacked-sequence {
          tunnel: w1883 -> [w1906]
          tunnel: w1869 -> [w1905]
          frame #0 {
            n1149 = case shown="True" w1906 {
              frame False {
              }
              frame True {
                # "ON"
                n1150 = local write "P1 CH1"(TRUE ("P1 CH1")) -> ()
              }
            }
            n1151 = case shown="True" w1905 {
              frame False {
              }
              frame True {
                # "OFF"
                n1152 = local write "P1 CH1"(FALSE ("P1 CH0")) -> ()
              }
            }
          }
        }
        n1153 = stacked-sequence {
          tunnel: w1889 -> [w1914]
          tunnel: w1863 -> [w1913]
          frame #0 {
            n1154 = case shown="True" w1914 {
              frame False {
              }
              frame True {
                # "ON"
                n1155 = local write "P2 CH0"(TRUE ("P2 CH0")) -> ()
              }
            }
            n1156 = case shown="True" w1913 {
              frame False {
              }
              frame True {
                # "OFF"
                n1157 = local write "P2 CH0"(FALSE ("P1 CH0")) -> ()
              }
            }
          }
        }
        n1158 = stacked-sequence {
          tunnel: w1841 -> [w1898]
          tunnel: w1836 -> [w1897]
          frame #0 {
            n1159 = case shown="True" w1898 {
              frame False {
              }
              frame True {
                # "ON"
                n1160 = local write "P1 CH2"(TRUE ("P2 CH1")) -> ()
              }
            }
            n1161 = case shown="True" w1897 {
              frame False {
              }
              frame True {
                # "OFF"
                n1162 = local write "P1 CH2"(FALSE ("P1 CH0")) -> ()
              }
            }
          }
        }
        n1163 = stacked-sequence {
          tunnel: w1895 -> [w1918]
          tunnel: w1856 -> [w1917]
          frame #0 {
            n1164 = case shown="True" w1918 {
              frame False {
              }
              frame True {
                # "ON"
                n1165 = local write "P2 CH1"(TRUE ("P2 CH1")) -> ()
              }
            }
            n1166 = case shown="True" w1917 {
              frame False {
              }
              frame True {
                # "OFF"
                n1167 = local write "P2 CH1"(FALSE ("P1 CH0")) -> ()
              }
            }
          }
        }
        n1168 = stacked-sequence {
          tunnel: w1844 -> [w1902]
          tunnel: w1849 -> [w1901]
          frame #0 {
            n1169 = case shown="True" w1902 {
              frame False {
              }
              frame True {
                # "ON"
                n1170 = local write "P2 CH2"(TRUE ("P2 CH1")) -> ()
              }
            }
            n1171 = case shown="True" w1901 {
              frame False {
              }
              frame True {
                # "OFF"
                n1172 = local write "P2 CH2"(FALSE ("P1 CH0")) -> ()
              }
            }
          }
        }
      }
      frame #1 {
        n1173 = local read "System Stop"() -> (w1921:bool)
      }
    }
    "Power OFF" <- w1821
    n1174 = Wait (ms)(milliseconds to wait=u32 1) -> ()  [unwired: 1 out]
  }
  n1175 = while {
    shift-right: [w1934] -> _
    shift-left: FALSE -> [w1936]
    tunnel: [w1926] -> _
    tunnel: [w1935] -> w40
    shift-right: [w1932] -> _
    shift-left: FALSE -> [w1933]
    shift-right: [w1930] -> _
    shift-left: FALSE -> [w1931]
    shift-right: [w1929] -> _
    shift-left: FALSE -> [w1928]
    tunnel: [w1926] -> w31
    tunnel: w3 -> [_]
    tunnel: w3 -> [_]
    tunnel: w3 -> [_]
    shift-right: [w1923] -> _
    shift-left: FALSE -> [w1925]
    shift-right: [w1922] -> _
    shift-left: FALSE -> [w1924]
    stop <- w1926 stop-if-true
    n1176 = Wait (ms)(milliseconds to wait="SEL Time Cycle") -> ()  [unwired: 1 out]
    n1177 = stacked-sequence {
      seq-local: [w1946 _ _ _] -> [_ _ w2187 _]
      seq-local: [w1945 _ _ _] -> [_ _ w2184 _]
      seq-local: [w1944 _ _ _] -> [_ _ w2182 _]
      seq-local: [w1943 _ _ _] -> [_ _ w2181 _]
      seq-local: [w1942 _ _ _] -> [_ _ w2174 _]
      seq-local: [w1937 _ _ _] -> [_ _ w2175 _]
      tunnel: w1936 -> [w1954 _ _ _]
      tunnel: [_ _ _ w2226] -> w1926
      tunnel: [_ w2164 _ _] -> w1935
      tunnel: [_ _ w2189 _] -> w1934
      tunnel: w1933 -> [w1952 _ _ _]
      tunnel: [_ _ w2183 _] -> w1932
      tunnel: w1931 -> [w1951 _ _ _]
      tunnel: [_ _ w2185 _] -> w1930
      tunnel: [_ _ w2186 _] -> w1929
      tunnel: w1928 -> [w1947 _ _ _]
      tunnel: w1925 -> [w1941 _ _ _]
      tunnel: w1924 -> [w1938 _ _ _]
      tunnel: [_ _ w2173 _] -> w1923
      tunnel: [_ _ w2172 _] -> w1922
      frame #0 {
        # "Детектирование SEL"
        n1178 = local read "P2 CH0"() -> (w1945:bool)
        n1179 = local read "P2 CH2"() -> (w1937:bool)
        n1180 = local read "P1 CH1"() -> (w1944:bool)
        n1181 = local read "P2 CH1"() -> (w1946:bool)
        n1182 = local read "P1 CH2"() -> (w1942:bool)
        n1183 = flat-sequence {
          tunnel: w1949 -> [w2019]
          frame #0 {
            n1184 = case shown="True" w2019 {
              frame False {
              }
              frame True {
                n1185 = Wait (ms)(milliseconds to wait=u32 50) -> ()  [unwired: 1 out]
              }
            }
          }
          frame #1 {
            n1186 = local read "P1 CH1_cur, A"() -> (w2024:dbl)
            n1187 = local read "SIM_SEL"() -> (w2022:bool)
            n1188 = Greater Or Equal?(x=w2024, y="P1 CH1_selcur, A") -> (x >= y?=w2025:bool)
            n1189 = Or(x=w2022, y=w2025) -> (x .or. y?=→"P1 CH1_warning":bool)
          }
          frame #2 {
            n1190 = local read "Считать SIM_SEL"() -> (w2031:bool)
            n1191 = local read "SIM_SEL"() -> (w2030:bool)
            n1192 = local read "P1 CH1_warning"() -> (w2026:bool)
            n1193 = Not(x=w2030) -> (.not. x?=w2029:bool)
            n1194 = Select(t=TRUE, s=w2031, f=w2029) -> (s? t:f=w2027:bool)
            n1195 = And(x=w2026, y=w2027) -> (x .and. y?=w2032:bool)
            n1196 = case shown="True" w2032 {
              frame False {
              }
              frame True {
                n1197 = local read "P1 CH1_counter"() -> (w2034:u32)
                n1198 = Increment(x=w2034) -> (x+1=→"P1 CH1_counter":u32)
              }
            }
          }
        }
        n1199 = flat-sequence {
          tunnel: w1950 -> [w2003]
          frame #0 {
            n1200 = case shown="True" w2003 {
              frame False {
              }
              frame True {
                n1201 = Wait (ms)(milliseconds to wait=u32 50) -> ()  [unwired: 1 out]
              }
            }
          }
          frame #1 {
            n1202 = local read "P2 CH0_cur, A"() -> (w2009:dbl)
            n1203 = local read "SIM_SEL"() -> (w2006:bool)
            n1204 = Greater Or Equal?(x=w2009, y="P2 CH0_selcur, A") -> (x >= y?=w2008:bool)
            n1205 = Or(x=w2006, y=w2008) -> (x .or. y?=→"P2 CH0_warning":bool)
          }
          frame #2 {
            n1206 = local read "Считать SIM_SEL"() -> (w2013:bool)
            n1207 = local read "SIM_SEL"() -> (w2014:bool)
            n1208 = local read "P2 CH0_warning"() -> (w2010:bool)
            n1209 = Not(x=w2014) -> (.not. x?=w2015:bool)
            n1210 = Select(t=TRUE, s=w2013, f=w2015) -> (s? t:f=w2012:bool)
            n1211 = And(x=w2010, y=w2012) -> (x .and. y?=w2011:bool)
            n1212 = case shown="True" w2011 {
              frame False {
              }
              frame True {
                n1213 = local read "P2 CH0_counter"() -> (w2018:u32)
                n1214 = Increment(x=w2018) -> (x+1=→"P2 CH0_counter":u32)
              }
            }
          }
        }
        n1215 = flat-sequence {
          tunnel: w1953 -> [w2035]
          frame #0 {
            n1216 = case shown="True" w2035 {
              frame False {
              }
              frame True {
                n1217 = Wait (ms)(milliseconds to wait=u32 50) -> ()  [unwired: 1 out]
              }
            }
          }
          frame #1 {
            n1218 = local read "P1 CH0_cur, A"() -> (w2041:dbl)
            n1219 = Greater Or Equal?(x=w2041, y="P1 CH0_selcur, A") -> (x >= y?=w2040:bool)
            n1220 = Or(x="SIM_SEL", y=w2040) -> (x .or. y?=→"P1 CH0_warning":bool)
          }
          frame #2 {
            n1221 = local read "SIM_SEL"() -> (w2047:bool)
            n1222 = local read "P1 CH0_warning"() -> (w2042:bool)
            n1223 = Not(x=w2047) -> (.not. x?=w2046:bool)
            n1224 = Select(t=TRUE, s="Считать SIM_SEL", f=w2046) -> (s? t:f=w2043:bool)
            n1225 = And(x=w2042, y=w2043) -> (x .and. y?=w2048:bool)
            n1226 = case shown="True" w2048 {
              frame False {
              }
              frame True {
                n1227 = local read "P1 CH0_counter"() -> (w2050:u32)
                n1228 = Increment(x=w2050) -> (x+1=→"P1 CH0_counter":u32)
              }
            }
          }
        }
        n1229 = flat-sequence {
          tunnel: w1939 -> [w1955]
          frame #0 {
            n1230 = case shown="True" w1955 {
              frame False {
              }
              frame True {
                n1231 = Wait (ms)(milliseconds to wait=u32 50) -> ()  [unwired: 1 out]
              }
            }
          }
          frame #1 {
            n1232 = local read "P2 CH2_cur, A"() -> (w1959:dbl)
            n1233 = local read "SIM_SEL"() -> (w1957:bool)
            n1234 = Greater Or Equal?(x=w1959, y="P2 CH2_selcur, A") -> (x >= y?=w1960:bool)
            n1235 = Or(x=w1957, y=w1960) -> (x .or. y?=→"P2 CH2_warning":bool)
          }
          frame #2 {
            n1236 = local read "Считать SIM_SEL"() -> (w1968:bool)
            n1237 = local read "SIM_SEL"() -> (w1967:bool)
            n1238 = local read "P2 CH2_warning"() -> (w1962:bool)
            n1239 = Not(x=w1967) -> (.not. x?=w1966:bool)
            n1240 = Select(t=TRUE, s=w1968, f=w1966) -> (s? t:f=w1964:bool)
            n1241 = And(x=w1962, y=w1964) -> (x .and. y?=w1963:bool)
            n1242 = case shown="True" w1963 {
              frame False {
              }
              frame True {
                n1243 = local read "P2 CH2_counter"() -> (w1970:u32)
                n1244 = Increment(x=w1970) -> (x+1=→"P2 CH2_counter":u32)
              }
            }
          }
        }
        n1245 = flat-sequence {
          tunnel: w1948 -> [w1987]
          frame #0 {
            n1246 = case shown="True" w1987 {
              frame False {
              }
              frame True {
                n1247 = Wait (ms)(milliseconds to wait=u32 50) -> ()  [unwired: 1 out]
              }
            }
          }
          frame #1 {
            n1248 = local read "P2 CH1_cur, A"() -> (w1991:dbl)
            n1249 = local read "SIM_SEL"() -> (w1989:bool)
            n1250 = Greater Or Equal?(x=w1991, y="P2 CH1_selcur, A") -> (x >= y?=w1992:bool)
            n1251 = Or(x=w1989, y=w1992) -> (x .or. y?=→"P2 CH1_warning":bool)
          }
          frame #2 {
            n1252 = local read "Считать SIM_SEL"() -> (w2000:bool)
            n1253 = local read "SIM_SEL"() -> (w1999:bool)
            n1254 = local read "P2 CH1_warning"() -> (w1994:bool)
            n1255 = Not(x=w1999) -> (.not. x?=w1998:bool)
            n1256 = Select(t=TRUE, s=w2000, f=w1998) -> (s? t:f=w1996:bool)
            n1257 = And(x=w1994, y=w1996) -> (x .and. y?=w1995:bool)
            n1258 = case shown="True" w1995 {
              frame False {
              }
              frame True {
                n1259 = local read "P2 CH1_counter"() -> (w2002:u32)
                n1260 = Increment(x=w2002) -> (x+1=→"P2 CH1_counter":u32)
              }
            }
          }
        }
        n1261 = local read "P1 CH0"() -> (w1943:bool)
        n1262 = flat-sequence {
          tunnel: w1940 -> [w1971]
          frame #0 {
            n1263 = case shown="True" w1971 {
              frame False {
              }
              frame True {
                n1264 = Wait (ms)(milliseconds to wait=u32 50) -> ()  [unwired: 1 out]
              }
            }
          }
          frame #1 {
            n1265 = local read "P1 CH2_cur, A"() -> (w1975:dbl)
            n1266 = local read "SIM_SEL"() -> (w1973:bool)
            n1267 = Greater Or Equal?(x=w1975, y="P1 CH2_selcur, A") -> (x >= y?=w1976:bool)
            n1268 = Or(x=w1973, y=w1976) -> (x .or. y?=→"P1 CH2_warning":bool)
          }
          frame #2 {
            n1269 = local read "Считать SIM_SEL"() -> (w1984:bool)
            n1270 = local read "SIM_SEL"() -> (w1983:bool)
            n1271 = local read "P1 CH2_warning"() -> (w1978:bool)
            n1272 = Not(x=w1983) -> (.not. x?=w1982:bool)
            n1273 = Select(t=TRUE, s=w1984, f=w1982) -> (s? t:f=w1980:bool)
            n1274 = And(x=w1978, y=w1980) -> (x .and. y?=w1979:bool)
            n1275 = case shown="True" w1979 {
              frame False {
              }
              frame True {
                n1276 = local read "P1 CH2_counter"() -> (w1986:u32)
                n1277 = Increment(x=w1986) -> (x+1=→"P1 CH2_counter":u32)
              }
            }
          }
        }
        n1278 = Greater?(x=w1945, y=w1951) -> (0:w1950:bool)
        n1279 = Greater?(x=w1943, y=w1954) -> (0:w1953:bool)
        n1280 = Greater?(x=w1937, y=w1938) -> (0:w1939:bool)
        n1281 = Greater?(x=w1944, y=w1952) -> (0:w1949:bool)
        n1282 = Greater?(x=w1946, y=w1947) -> (0:w1948:bool)
        n1283 = Greater?(x=w1942, y=w1941) -> (0:w1940:bool)
      }
      frame #1 {
        w2073 = "\t"
        w2056 = "\t"
        w2059 = 0
        w2060 = 6
        w2064 = 6
        w2090 = "\t"
        w2074 = "\t"
        w2076 = 0
        w2077 = 6
        w2082 = 6
        w2093 = "\t"
        w2103 = "\t"
        w2105 = "\t"
        w2107 = "\t"
        w2094 = "\t"
        w2095 = "\t"
        w2096 = "\t"
        w2097 = "\t"
        w2138 = 0
        w2137 = 6
        w2133 = 6
        w2143 = 0
        w2144 = 6
        w2148 = 6
        w2157 = 0
        w2156 = 6
        w2151 = 6
        w2160 = 0
        w2161 = 6
        w2167 = 6
        # "Запись логов"
        n1284 = local read "P1 CH2_cur, A"() -> (w2078:dbl)
        n1285 = local read "P1 CH1_cur, A"() -> (w2155:dbl)
        n1286 = local read "P1 CH2, V"() -> (w2080:dbl)
        n1287 = local read "P1 CH2_counter"() -> (w2075:u32)
        n1288 = local read "P1 CH2_warning"() -> (w2079:bool)
        n1289 = local read "P2 CH1, V"() -> (w2140:dbl)
        n1290 = local read "P2 CH1_cur, A"() -> (w2136:dbl)
        n1291 = local read "P2 CH1_counter"() -> (w2139:u32)
        n1292 = local read "P2 CH1_warning"() -> (w2135:bool)
        n1293 = local read "P2 CH2, V"() -> (w2057:dbl)
        n1294 = local read "P2 CH2_cur, A"() -> (w2061:dbl)
        n1295 = local read "P2 CH2_counter"() -> (w2058:u32)
        n1296 = local read "P2 CH2_warning"() -> (w2062:bool)
        n1297 = local read "P1 CH0, V"() -> (w2165:dbl)
        n1298 = local read "P1 CH0_cur, A"() -> (w2162:dbl)
        n1299 = local read "P1 CH0_counter"() -> (w2159:u32)
        n1300 = local read "P1 CH0_warning"() -> (w2163:bool)
        n1301 = local read "P1 CH1, V"() -> (w2153:dbl)
        n1302 = local read "P1 CH1_counter"() -> (w2158:u32)
        n1303 = local read "P1 CH1_warning"() -> (w2154:bool)
        n1304 = local read "P2 CH0, V"() -> (w2141:dbl)
        n1305 = local read "P2 CH0_cur, A"() -> (w2145:dbl)
        n1306 = local read "P2 CH0_counter"() -> (w2142:u32)
        n1307 = local read "P2 CH0_warning"() -> (w2146:bool)
        n1308 = Number To Fractional String(number=w2080, width (-)=w2082, precision (6)=w2082) -> (F-format string=w2084:string)  [unwired: 1 in]
        n1309 = Number To Fractional String(number=w2078, width (-)=w2077, precision (6)=w2077) -> (F-format string=w2085:string)  [unwired: 1 in]
        n1310 = Number To Fractional String(number=w2075, width (-)=w2076, precision (6)=w2076) -> (F-format string=w2086:string)  [unwired: 1 in]
        n1311 = Number To Fractional String(number=w2140, width (-)=w2133, precision (6)=w2133) -> (F-format string=w2119:string)  [unwired: 1 in]
        n1312 = Number To Fractional String(number=w2136, width (-)=w2137, precision (6)=w2137) -> (F-format string=w2118:string)  [unwired: 1 in]
        n1313 = Number To Fractional String(number=w2139, width (-)=w2138, precision (6)=w2138) -> (F-format string=w2117:string)  [unwired: 1 in]
        n1314 = Number To Fractional String(number=w2057, width (-)=w2064, precision (6)=w2064) -> (F-format string=w2066:string)  [unwired: 1 in]
        n1315 = Number To Fractional String(number=w2061, width (-)=w2060, precision (6)=w2060) -> (F-format string=w2067:string)  [unwired: 1 in]
        n1316 = Number To Fractional String(number=w2058, width (-)=w2059, precision (6)=w2059) -> (F-format string=w2068:string)  [unwired: 1 in]
        n1317 = Number To Fractional String(number=w2165, width (-)=w2167, precision (6)=w2167) -> (F-format string=w2131:string)  [unwired: 1 in]
        n1318 = Number To Fractional String(number=w2162, width (-)=w2161, precision (6)=w2161) -> (F-format string=w2130:string)  [unwired: 1 in]
        n1319 = Number To Fractional String(number=w2159, width (-)=w2160, precision (6)=w2160) -> (F-format string=w2129:string)  [unwired: 1 in]
        n1320 = Number To Fractional String(number=w2153, width (-)=w2151, precision (6)=w2151) -> (F-format string=w2127:string)  [unwired: 1 in]
        n1321 = Number To Fractional String(number=w2155, width (-)=w2156, precision (6)=w2156) -> (F-format string=w2126:string)  [unwired: 1 in]
        n1322 = Number To Fractional String(number=w2158, width (-)=w2157, precision (6)=w2157) -> (F-format string=w2125:string)  [unwired: 1 in]
        n1323 = Number To Fractional String(number=w2141, width (-)=w2148, precision (6)=w2148) -> (F-format string=w2123:string)  [unwired: 1 in]
        n1324 = Number To Fractional String(number=w2145, width (-)=w2144, precision (6)=w2144) -> (F-format string=w2122:string)  [unwired: 1 in]
        n1325 = Number To Fractional String(number=w2142, width (-)=w2143, precision (6)=w2143) -> (F-format string=w2121:string)  [unwired: 1 in]
        n1326 = Select(t="!!!2", s=w2079, f="") -> (s? t:f=w2087:string)
        n1327 = Select(t="!!!4", s=w2135, f="") -> (s? t:f=w2116:string)
        n1328 = Select(t="!!!5", s=w2062, f="") -> (s? t:f=w2069:string)
        n1329 = Select(t="!!!0", s=w2163, f="") -> (s? t:f=w2128:string)
        n1330 = Select(t="!!!1", s=w2154, f="") -> (s? t:f=w2124:string)
        n1331 = Select(t="!!!3", s=w2146, f="") -> (s? t:f=w2120:string)
        n1332 = local read "P1 CH2 Used"() -> (w2089:bool)
        n1333 = local read "P1 CH0 Used"() -> (w2112:bool)
        n1334 = local read "P1 CH1 Used"() -> (w2111:bool)
        n1335 = local read "P2 CH0 Used"() -> (w2110:bool)
        n1336 = local read "P2 CH1 Used"() -> (w2109:bool)
        n1337 = local read "P2 CH2 Used"() -> (w2070:bool)
        n1338 = Concatenate Strings(w2074, w2084, w2074, w2085, w2074, w2086, w2074, w2087) -> (w2088:string)
        n1339 = Concatenate Strings(w2097, w2131, w2097, w2130, w2097, w2129, w2097, w2128) -> (w2114:string)
        n1340 = Concatenate Strings(w2096, w2127, w2096, w2126, w2096, w2125, w2096, w2124) -> (w2115:string)
        n1341 = Concatenate Strings(w2095, w2123, w2095, w2122, w2095, w2121, w2095, w2120) -> (w2113:string)
        n1342 = Concatenate Strings(w2094, w2119, w2094, w2118, w2094, w2117, w2094, w2116) -> (w2108:string)
        n1343 = Concatenate Strings(w2056, w2066, w2056, w2067, w2056, w2068, w2056, w2069) -> (w2071:string)
        n1344 = Concatenate Strings(w2090, w2090, w2090, w2090) -> (w2091:string)
        n1345 = Concatenate Strings(w2107, w2107, w2107, w2107) -> (w2106:string)
        n1346 = Concatenate Strings(w2105, w2105, w2105, w2105) -> (w2104:string)
        n1347 = Concatenate Strings(w2103, w2103, w2103, w2103) -> (w2102:string)
        n1348 = Concatenate Strings(w2093, w2093, w2093, w2093) -> (w2101:string)
        n1349 = Concatenate Strings(w2073, w2073, w2073, w2073) -> (w2072:string)
        n1350 = Select(t=w2088, s=w2089, f=w2091) -> (s? t:f=w2055:string)
        n1351 = Select(t=w2114, s=w2112, f=w2106) -> (s? t:f=w2100:string)
        n1352 = Select(t=w2115, s=w2111, f=w2104) -> (s? t:f=w2099:string)
        n1353 = Select(t=w2113, s=w2110, f=w2102) -> (s? t:f=w2054:string)
        n1354 = Select(t=w2108, s=w2109, f=w2101) -> (s? t:f=w2053:string)
        n1355 = Select(t=w2071, s=w2070, f=w2072) -> (s? t:f=w2052:string)
        n1356 = Get Date/Time In Seconds() -> (seconds since 1Jan1904=w2170:timestamp)
        n1357 = Format Date/Time String(time format string (%c)="%H:%M:%S:%3u", seconds (now)=w2170) -> (date/time string=w2168:string)  [unwired: 1 in]
        n1358 = local read "SEL output file refnum"() -> (w2092:refnum<file>)
        n1359 = Concatenate Strings(w2168, w2100, w2099, w2055, w2054, w2053, w2052, "\r\n") -> (w2098:string)
        n1360 = Format Into String(initial string=w2092, w2098) -> (resulting string=w2164:refnum<file>)  [unwired: 2 in, 1 out]
      }
      frame #2 {
        n1361 = local read "P1 CH0_warning"() -> (w2188:bool)
        "SEL" <- w2188
        n1362 = local read "P1 CH1_warning"() -> (w2180:bool)
        n1363 = local read "P2 CH0_warning"() -> (w2178:bool)
        n1364 = local read "P2 CH1_warning"() -> (w2179:bool)
        n1365 = local read "P1 CH2_warning"() -> (w2177:bool)
        n1366 = local read "P2 CH2_warning"() -> (w2176:bool)
        n1367 = local write "SEL"(w2178) -> ()
        n1368 = local write "SEL"(w2180) -> ()
        n1369 = local write "SEL"(w2179) -> ()
        n1370 = local write "SEL"(w2177) -> ()
        n1371 = local write "SEL"(w2176) -> ()
        n1372 = case shown="True" w2188 {
          tunnel: [w2220 w2221] -> w2189
          tunnel: w2181 -> [w2220 _]
          frame False {
          }
          frame True {
            n1373 = flat-sequence {
              tunnel: [FALSE] -> w2221
              frame #0 {
                n1374 = local write "P1 CH0"(FALSE ("Power")) -> ()
              }
              frame #1 {
                n1375 = Wait (ms)(milliseconds to wait=u32 100 ("Wait_parry, ms")) -> ()  [unwired: 1 out]
              }
              frame #2 {
                n1376 = local write "P1 CH0"(TRUE ("Power")) -> ()
              }
            }
          }
        }
        n1377 = case shown="True" w2180 {
          tunnel: [w2214 w2215] -> w2183
          tunnel: w2182 -> [w2214 _]
          frame False {
          }
          frame True {
            n1378 = flat-sequence {
              tunnel: [FALSE] -> w2215
              frame #0 {
                n1379 = local write "P1 CH1"(FALSE ("Power")) -> ()
              }
              frame #1 {
                n1380 = Wait (ms)(milliseconds to wait=u32 100 ("Wait_parry, ms")) -> ()  [unwired: 1 out]
              }
              frame #2 {
                n1381 = local write "P1 CH1"(TRUE ("Power")) -> ()
              }
            }
          }
        }
        n1382 = case shown="True" w2178 {
          tunnel: [w2208 w2209] -> w2185
          tunnel: w2184 -> [w2208 _]
          frame False {
          }
          frame True {
            n1383 = flat-sequence {
              tunnel: [FALSE] -> w2209
              frame #0 {
                n1384 = local write "P2 CH0"(FALSE ("Power")) -> ()
              }
              frame #1 {
                n1385 = Wait (ms)(milliseconds to wait=u32 100 ("Wait_parry, ms")) -> ()  [unwired: 1 out]
              }
              frame #2 {
                n1386 = local write "P2 CH0"(TRUE ("Power")) -> ()
              }
            }
          }
        }
        n1387 = case shown="True" w2179 {
          tunnel: [w2202 w2203] -> w2186
          tunnel: w2187 -> [w2202 _]
          frame False {
          }
          frame True {
            n1388 = flat-sequence {
              tunnel: [FALSE] -> w2203
              frame #0 {
                n1389 = local write "P2 CH1"(FALSE ("Power")) -> ()
              }
              frame #1 {
                n1390 = Wait (ms)(milliseconds to wait=u32 100 ("Wait_parry, ms")) -> ()  [unwired: 1 out]
              }
              frame #2 {
                n1391 = local write "P2 CH1"(TRUE ("Power")) -> ()
              }
            }
          }
        }
        n1392 = case shown="True" w2177 {
          tunnel: [w2196 w2197] -> w2173
          tunnel: w2174 -> [w2196 _]
          frame False {
          }
          frame True {
            n1393 = flat-sequence {
              tunnel: [FALSE] -> w2197
              frame #0 {
                n1394 = local write "P1 CH2"(FALSE ("Power")) -> ()
              }
              frame #1 {
                n1395 = Wait (ms)(milliseconds to wait=u32 100 ("Wait_parry, ms")) -> ()  [unwired: 1 out]
              }
              frame #2 {
                n1396 = local write "P1 CH2"(TRUE ("Power")) -> ()
              }
            }
          }
        }
        n1397 = case shown="True" w2176 {
          tunnel: [w2190 w2191] -> w2172
          tunnel: w2175 -> [w2190 _]
          frame False {
          }
          frame True {
            n1398 = flat-sequence {
              tunnel: [FALSE] -> w2191
              frame #0 {
                n1399 = local write "P2 CH2"(FALSE ("Power")) -> ()
              }
              frame #1 {
                n1400 = Wait (ms)(milliseconds to wait=u32 100 ("Wait_parry, ms")) -> ()  [unwired: 1 out]
              }
              frame #2 {
                n1401 = local write "P2 CH2"(TRUE ("Power")) -> ()
              }
            }
          }
        }
      }
      frame #3 {
        n1402 = local read "System Stop"() -> (w2226:bool)
      }
    }
  }
  n1403 = while {
    tunnel: w1 -> [_]
    stop <- w2229 stop-if-true
    n1404 = Wait (ms)(milliseconds to wait=u32 100) -> ()  [unwired: 1 out]
    n1405 = case shown="True" "HMI Stop" {
      selector: "HMI Stop" -> [w2230 _]
      tunnel: [w2230 w2231] -> w2229
      frame False {
      }
      frame True {
        n1406 = local read "Glass Meas Cycle Running"() -> (w2236:bool)
        n1407 = local read "Meas Running"() -> (w2234:bool)
        n1408 = Not(x=w2236) -> (.not. x?=w2233:bool)
        n1409 = Not(x=w2234) -> (.not. x?=w2235:bool)
        n1410 = Compound Arithmetic op=AND(w2233, w2235) -> (w2232:bool)
        n1411 = case shown="False" w2232 {
          selector: w2232 -> [w2237 w2242]
          tunnel: [w2237 w2242] -> w2231
          frame False {
            n1412 = One Button Dialog(message="Please, wait for the measurement to complete.", button name ("OK")="Oh, shit, I'm sorry.") -> (true=w2241:bool)
            n1413 = Not(x=w2241) -> (.not. x?=w2240:bool)
            n1414 = local write "HMI Stop"(w2240) -> ()
          }
          frame True {
            n1415 = local write "System Stop"(w2242) -> ()
          }
        }
      }
    }
  }
  n1416 = case shown="True" w16 {
    tunnel: w3 -> [_ w2244]
    frame False {
    }
    frame True {
      n1417 = local read "Ophir 2 dup Visa Session"() -> (w2246:refnum<visa-resource-name>)
      n1418 = local read "Ophir 2 error out"() -> (w2245:errorcluster)
      n1419 = while {
        tunnel: [w2257] -> w2248
        tunnel: [w2251] -> w2247
        tunnel: w2246 -> [w2255]
        tunnel: w2245 -> [w2254]
        tunnel: w2244 -> [_]
        shift-right: [w2252] -> _
        shift-left: 0.0 -> [w2253]
        stop <- w2256 stop-if-true
        n1420 = Wait (ms)(milliseconds to wait="Ophir 2 Wait") -> ()  [unwired: 1 out]
        n1421 = stacked-sequence {
          tunnel: [w2273] -> w2257
          tunnel: [w2258] -> w2256
          tunnel: w2255 -> [w2259]
          tunnel: w2254 -> [w2268]
          tunnel: w2253 -> [w2262]
          tunnel: [w2260] -> w2252
          tunnel: [w2259] -> w2251
          frame #0 {
            n1422 = Fract/Exp String To Number(string="Ophir 2 units") -> (number=w2261:dbl)  [unwired: 3 in, 1 out]
            n1423 = call "Ophir SendPower.vi"("Visa Session"=w2259, "error in (no error)"=w2268) -> ("Value Number"=w2270:dbl, "Value String"=w2271:string, "error out"=w2273:errorcluster)  [unwired: 1 out]
            "Ophir 2 Real Optical Power" <- w2270
            n1424 = call "Ophir Over.vi"("Value String"=w2271) -> ("Overrange"=→"Ophir 2 Over Range":bool)
            n1425 = Multiply(x=w2270, y=w2261) -> (x*y=w2266:dbl)
            "Ophir 2 Char" <- w2266
            "Ophir 2 Optical Power" <- w2266
            n1426 = Greater Or Equal?(x=w2266, y=w2262) -> (x >= y?=w2267:bool)
            n1427 = Select(t=0.0, s="Ophir 2 Clear", f=w2262) -> (s? t:f=w2265:dbl)
            n1428 = Select(t=w2266, s=w2267, f=w2265) -> (s? t:f=w2260:dbl)
            "Ophir 2 MAX" <- w2260
            n1429 = local read "System Stop"() -> (w2258:bool)
          }
        }
      }
      n1430 = VISA Close(VISA resource name=w2247, error in (no error)=w2248) -> (error out=w2249:errorcluster)
      n1431 = call "Ophir Error Message.vi"("error in (no error)"=w2249) -> ()  [unwired: 3 in, 4 out]
    }
  }
  n1432 = case shown="True" w17 {
    tunnel: w3 -> [_ w2275]
    frame False {
    }
    frame True {
      n1433 = local read "Ophir 1 dup Visa Session"() -> (w2277:refnum<visa-resource-name>)
      n1434 = local read "Ophir 1 error out"() -> (w2276:errorcluster)
      n1435 = while {
        tunnel: [w2288] -> w2279
        tunnel: [w2282] -> w2278
        tunnel: w2277 -> [w2286]
        tunnel: w2276 -> [w2285]
        tunnel: w2275 -> [_]
        shift-right: [w2283] -> _
        shift-left: 0.0 -> [w2284]
        stop <- w2287 stop-if-true
        n1436 = Wait (ms)(milliseconds to wait="Ophir 1 Wait") -> ()  [unwired: 1 out]
        n1437 = stacked-sequence {
          tunnel: [w2304] -> w2288
          tunnel: [w2289] -> w2287
          tunnel: w2286 -> [w2291]
          tunnel: w2285 -> [w2300]
          tunnel: w2284 -> [w2294]
          tunnel: [w2292] -> w2283
          tunnel: [w2291] -> w2282
          frame #0 {
            n1438 = Fract/Exp String To Number(string="Ophir 1 units") -> (number=w2293:dbl)  [unwired: 3 in, 1 out]
            n1439 = call "Ophir SendPower.vi"("Visa Session"=w2291, "error in (no error)"=w2300) -> ("Value Number"=w2290:dbl, "Value String"=w2302:string, "error out"=w2304:errorcluster)  [unwired: 1 out]
            "Ophir 1 Real Optical Power" <- w2290
            n1440 = call "Ophir Over.vi"("Value String"=w2302) -> ("Overrange"=→"Ophir 1 Over Range":bool)
            n1441 = Multiply(x=w2290, y=w2293) -> (x*y=w2298:dbl)
            "Ophir 1 Char" <- w2298
            "Ophir 1 Optical Power" <- w2298
            n1442 = Greater Or Equal?(x=w2298, y=w2294) -> (x >= y?=w2299:bool)
            n1443 = Select(t=0.0, s="Ophir 1 Clear", f=w2294) -> (s? t:f=w2297:dbl)
            n1444 = Select(t=w2298, s=w2299, f=w2297) -> (s? t:f=w2292:dbl)
            "Ophir 1 MAX" <- w2292
            n1445 = local read "System Stop"() -> (w2289:bool)
          }
        }
      }
      n1446 = VISA Close(VISA resource name=w2278, error in (no error)=w2279) -> (error out=w2280:errorcluster)
      n1447 = call "Ophir Error Message.vi"("error in (no error)"=w2280) -> ()  [unwired: 3 in, 4 out]
    }
  }
  n1448 = flat-sequence {
    tunnel: w40 -> [w2321]
    tunnel: w35 -> [w2320]
    tunnel: w34 -> [w2319]
    tunnel: w31 -> [_]
    tunnel: w30 -> [w2318]
    tunnel: w29 -> [w2317]
    frame #0 {
      # "STOP"
      n1449 = call <instrlib>:"niDCPower Close.vi"("error in (no error)"=w2317, "instrument handle"=w2319) -> ("error out"=w2315:errorcluster)  [unwired: 9 in]
      n1450 = call <instrlib>:"niDCPower Close.vi"("error in (no error)"=w2318, "instrument handle"=w2320) -> ("error out"=w2316:errorcluster)  [unwired: 9 in]
      n1451 = Close File(refnum=w2321) -> ()  [unwired: 1 in, 2 out]
      n1452 = call <vilib>:"Simple Error Handler.vi"("error in (no error)"=w2315) -> ("error out"=w2313:errorcluster)  [unwired: 1 in, 7 out]
      n1453 = local write "DC Power 2 error out"(w2313) -> ()
      n1454 = call <vilib>:"Simple Error Handler.vi"("error in (no error)"=w2316) -> ("error out"=w2314:errorcluster)  [unwired: 1 in, 7 out]
      n1455 = local write "DC Power 1 error out"(w2314) -> ()
      n1456 = Wait (ms)(milliseconds to wait=u32 1) -> ()  [unwired: 1 out]
      n1457 = property on="NI Scope Tab" class="TabCtl (strict)"("DisabledEnum"=T5."Enabled" ("Disabled")) -> ()  [unwired: 2 in, 2 out]
      n1458 = property on="NI DMM 1 Tab" class="TabCtl (strict)"("DisabledEnum"=T5."Enabled" ("Disabled")) -> ()  [unwired: 2 in, 2 out]
      n1459 = property on="NI DMM 2 Tab" class="TabCtl (strict)"("DisabledEnum"=T5."Enabled" ("Disabled")) -> ()  [unwired: 2 in, 2 out]
      n1460 = property on="NI DMM 3 Tab" class="TabCtl (strict)"("DisabledEnum"=T5."Enabled" ("Disabled")) -> ()  [unwired: 2 in, 2 out]
      n1461 = property on="Ophir 1 Tab" class="TabCtl (strict)"("DisabledEnum"=T5."Enabled" ("Disabled")) -> ()  [unwired: 2 in, 2 out]
      n1462 = property on="Ophir 2 Tab" class="TabCtl (strict)"("DisabledEnum"=T5."Enabled" ("Disabled")) -> ()  [unwired: 2 in, 2 out]
      n1463 = property on="Stepper Motor Control" class="TabCtl (strict)"("DisabledEnum"=T5."Enabled" ("Disabled")) -> ()  [unwired: 2 in, 2 out]
      n1464 = property on="Table Tab" class="TabCtl (strict)"("DisabledEnum"=T5."Enabled" ("Disabled")) -> ()  [unwired: 2 in, 2 out]
    }
  }
